vi "integrate_data view.vi"(8 "Y-column names":string[](array[string])=["col0"], 10 "column extension":string[](array[string])=["SCM1_2020Aug_AC.008.txt"], 11 "Graph array":cluster{"output":dbl[], "output":dbl[]}[](array[cluster])=[{"output"=array[591 elements], "output"=array[591 elements]}]) -> ()   [LabVIEW 2025]
uses:
  <vilib>/Analysis/2dsp.llb/Integral Method.ctl
  <vilib>/Analysis/1siggen.llb/Ramp Pattern by Samples.vi
  <vilib>/Analysis/NI_AALBase.lvlib
  <vilib>/gmath/NI_Gmath.lvlib
  <vilib>/Analysis/NI_AALPro.lvlib
panel:
  out "Raw-field, Raw-data, Subtracted, Bkg-field, Bkg-data":string
  out "Integrated (X_interpol. Integ_interpol)":string
  in  "+b":dbl
  in  "*a":dbl=1.0
  out "error":errorcluster
  in  "bkg = Y*a+b":string="-0.02\t1.7128E-5\n-0.02\t1.7128E-5\n-0.02\t1.7128E-5\n-0.02\t1.7128E-5\n-0.02\t1.7128E-5\n-0.02\t1.7128E-5\n-0.02\t1.7128E-5\n-0.02\t1.7128E-5\n-0.02\t1.7128E-5\n-0.02\t1.7128E-5\n-0.02\t1.7128E-5\n-0.0104\t1.7129E-5\n-0.01\t1.7129E-5\n-0.01\t1.7129E-5\n-0.01\t1.7129E-5\n-0.01\t1.7129E-5\n-0.01\t1.7129E-5\n-0.01\t1.7129E-5\n-0.01\t1.7129E-5\n-0.01\t1.7129E-5\n-0.01\t1.7129E-5\n-0.01\t1.7129E-5\n-4E-4\t1.7129E-5\n3.46945E-18\t1.7129E-5\n3.46945E-18\t1.7129E-5\n3.46945E-18\t1.7129E-5\n3.46945E-18\t1.7129E-5\n3.46945E-18\t1.7129E-5\n3.46945E-18\t1.7129E-5\n3.46945E-18\t1.7129E-5\n3.46945E-18\t1.7129E-5\n3.46945E-18\t1.7129E-5\n3.46945E-18\t1.7129E-5\n3.46945E-18\t1.7129E-5\n0.01\t1.713E-5\n0.01\t1.713E-5\n0.01\t1.713E-5\n0.01\t1.713E-5\n0.01\t1.713E-5\n0.01\t1.713E-5\n0.01\t1.713E-5\n0.01\t1.713E-5\n0.01\t1.713E-5\n0.01\t1.713E-5\n0.01\t1.713E-5\n0.02\t1.713E-5\n0.02\t1.713E-5\n0.02\t1.713E-5\n0.02\t1.713E-5\n0.02\t1.713E-5\n0.02\t1.713E-5\n0.02\t1.713E-5\n0.02\t1.713E-5\n0.02\t1.713E-5\n0.02\t1.713E-5\n0.02\t1.713E-5\n0.02\t1.713E-5\n0.02848\t1.7131E-5\n0.03\t1.7131E-5\n0.03\t1.7131E-5\n0.03\t1.7131E-5\n0.03\t1.7131E-5\n0.03\t1.7131E-5\n0.03\t1.7131E-5\n0.03\t1.7131E-5\n0.03\t1.7131E-5\n0.03\t1.7131E-5\n0.03\t1.7131E-5\n0.03\t1.7131E-5\n0.04\t1.7131E-5\n0.04\t1.7131E-5\n0.04\t1.7131E-5\n0.04\t1.7131E-5\n0.04\t1.7131E-5\n0.04\t1.7131E-5\n0.04\t1.7131E-5\n0.04\t1.7131E-5\n0.04\t1.7131E-5\n0.04\t1.7131E-5\n0.04\t1.7131E-5\n0.05\t1.7132E-5\n0.05\t1.7132E-5\n0.05\t1.7132E-5\n0.05\t1.7132E-5\n0.05\t1.7132E-5\n0.05\t1.7132E-5\n0.05\t1.7132E-5\n0.05\t1.7132E-5\n0.05\t1.7132E-5\n0.05\t1.7132E-5\n0.05\t1.7132E-5\n0.05\t1.7132E-5\n0.06\t1.7132E-5\n0.06\t1.7132E-5\n0.06\t1.7132E-5\n0.06\t1.7132E-5\n0.06\t1.7132E-5\n0.06\t1.7132E-5\n0.06\t1.7132E-5\n0.06\t1.7132E-5\n0.06\t1.7132E-5\n0.06\t1.7132E-5\n0.06\t1.7132E-5\n0.06\t1.7132E-5\n0.07\t1.7133E-5\n0.07\t1.7133E-5\n0.07\t1.7133E-5\n0.07\t1.7133E-5\n0.07\t1.7133E-5\n0.07\t1.7133E-5\n0.07\t1.7133E-5\n0.07\t1.7133E-5\n0.07\t1.7133E-5\n0.07\t1.7133E-5\n0.07\t1.7133E-5\n0.08\t1.7133E-5\n0.08\t1.7133E-5\n0.08\t1.7133E-5\n0.08\t1.7133E-5\n0.08\t1.7133E-5\n0.08\t1.7133E-5\n0.08\t1.7133E-5\n0.08\t1.7133E-5\n0.08\t1.7133E-5\n0.08\t1.7133E-5\n0.08\t1.7133E-5\n0.08952\t1.7134E-5\n0.09\t1.7134E-5\n0.09\t1.7134E-5\n0.09\t1.7134E-5\n0.09\t1.7134E-5\n0.09\t1.7134E-5\n0.09\t1.7134E-5\n0.09\t1.7134E-5\n0.09\t1.7134E-5\n0.09\t1.7134E-5\n0.09\t1.7134E-5\n0.09\t1.7134E-5\n0.1\t1.7134E-5\n0.1\t1.7134E-5\n0.1\t1.7134E-5\n0.1\t1.7134E-5\n0.1\t1.7134E-5\n0.1\t1.7134E-5\n0.1\t1.7134E-5\n0.1\t1.7134E-5\n0.1\t1.7134E-5\n0.1\t1.7134E-5\n0.1\t1.7134E-5\n0.1\t1.7134E-5\n0.10948\t1.7134E-5\n0.11\t1.7134E-5\n0.11\t1.7134E-5\n0.11\t1.7134E-5\n0.11\t1.7134E-5\n0.11\t1.7134E-5\n0.11\t1.7134E-5\n0.11\t1.7134E-5\n0.11\t1.7134E-5\n0.11\t1.7134E-5\n0.11\t1.7134E-5\n0.11\t1.7134E-5\n0.12\t1.7135E-5\n0.12\t1.7135E-5\n0.12\t1.7135E-5\n0.12\t1.7135E-5\n0.12\t1.7135E-5\n0.12\t1.7135E-5\n0.12\t1.7135E-5\n0.12\t1.7135E-5\n0.12\t1.7135E-5\n0.12\t1.7135E-5\n0.12\t1.7135E-5\n0.129\t1.7135E-5\n0.13\t1.7135E-5\n0.13\t1.7135E-5\n0.13\t1.7135E-5\n0.13\t1.7135E-5\n0.13\t1.7135E-5\n0.13\t1.7135E-5\n0.13\t1.7135E-5\n0.13\t1.7135E-5\n0.13\t1.7135E-5\n0.13\t1.7135E-5\n0.13\t1.7135E-5\n0.13948\t1.7135E-5\n0.14\t1.7135E-5\n0.14\t1.7135E-5\n0.14\t1.7135E-5\n0.14\t1.7135E-5\n0.14\t1.7135E-5\n0.14\t1.7135E-5\n0.14\t1.7135E-5\n0.14\t1.7135E-5\n0.14\t1.7135E-5\n0.14\t1.7135E-5\n0.14\t1.7135E-5\n0.1496\t1.7136E-5\n0.15\t1.7136E-5\n0.15\t1.7136E-5\n0.15\t1.7136E-5\n0.15\t1.7136E-5\n0.15\t1.7136E-5\n0.15\t1.7136E-5\n0.15\t1.7136E-5\n0.15\t1.7136E-5\n0.15\t1.7136E-5\n0.15\t1.7136E-5\n0.15\t1.7136E-5\n0.16\t1.7136E-5\n0.16\t1.7136E-5\n0.16\t1.7136E-5\n0.16\t1.7136E-5\n0.16\t1.7136E-5\n0.16\t1.7136E-5\n0.16\t1.7136E-5\n0.16\t1.7136E-5\n0.16\t1.7136E-5\n0.16\t1.7136E-5\n0.16\t1.7136E-5\n0.17\t1.7136E-5\n0.17\t1.7136E-5\n0.17\t1.7136E-5\n0.17\t1.7136E-5\n0.17\t1.7136E-5\n0.17\t1.7136E-5\n0.17\t1.7136E-5\n0.17\t1.7136E-5\n0.17\t1.7136E-5\n0.17\t1.7136E-5\n0.17\t1.7136E-5\n0.18\t1.7137E-5\n0.18\t1.7137E-5\n0.18\t1.7137E-5\n0.18\t1.7137E-5\n0.18\t1.7137E-5\n0.18\t1.7137E-5\n0.18\t1.7137E-5\n0.18\t1.7137E-5\n0.18\t1.7137E-5\n0.18\t1.7137E-5\n0.18\t1.7137E-5\n0.18\t1.7137E-5\n0.19\t1.7137E-5\n0.19\t1.7137E-5\n0.19\t1.7137E-5\n0.19\t1.7137E-5\n0.19\t1.7137E-5\n0.19\t1.7137E-5\n0.19\t1.7137E-5\n0.19\t1.7137E-5\n0.19\t1.7137E-5\n0.19\t1.7137E-5\n0.19\t1.7137E-5\n0.19\t1.7137E-5\n0.19952\t1.7137E-5\n0.2\t1.7137E-5\n0.2\t1.7137E-5\n0.2\t1.7137E-5\n0.2\t1.7137E-5\n0.2\t1.7137E-5\n0.2\t1.7137E-5\n0.2\t1.7137E-5\n0.2\t1.7137E-5\n0.2\t1.7137E-5\n0.2\t1.7137E-5\n0.2\t1.7137E-5\n0.20956\t1.7137E-5\n0.21\t1.7137E-5\n0.21\t1.7137E-5\n0.21\t1.7137E-5\n0.21\t1.7137E-5\n0.21\t1.7137E-5\n0.21\t1.7137E-5\n0.21\t1.7137E-5\n0.21\t1.7137E-5\n0.21\t1.7137E-5\n0.21\t1.7137E-5\n0.21\t1.7137E-5\n0.22\t1.7138E-5\n0.22\t1.7138E-5\n0.22\t1.7138E-5\n0.22\t1.7138E-5\n0.22\t1.7138E-5\n0.22\t1.7138E-5\n0.22\t1.7138E-5\n0.22\t1.7138E-5\n0.22\t1.7138E-5\n0.22\t1.7138E-5\n0.22\t1.7138E-5\n0.23\t1.7138E-5\n0.23\t1.7138E-5\n0.23\t1.7138E-5\n0.23\t1.7138E-5\n0.23\t1.7138E-5\n0.23\t1.7138E-5\n0.23\t1.7138E-5\n0.23\t1.7138E-5\n0.23\t1.7138E-5\n0.23\t1.7138E-5\n0.23\t1.7138E-5\n0.23948\t1.7138E-5\n0.24\t1.7138E-5\n0.24\t1.7138E-5\n0.24\t1.7138E-5\n0.24\t1.7138E-5\n0.24\t1.7138E-5\n0.24\t1.7138E-5\n0.24\t1.7138E-5\n0.24\t1.7138E-5\n0.24\t1.7138E-5\n0.24\t1.7138E-5\n0.24\t1.7138E-5\n0.25\t1.7138E-5\n0.25\t1.7138E-5\n0.25\t1.7138E-5\n0.25\t1.7138E-5\n0.25\t1.7138E-5\n0.25\t1.7138E-5\n0.25\t1.7138E-5\n0.25\t1.7138E-5\n0.25\t1.7138E-5\n0.25\t1.7138E-5\n0.25\t1.7138E-5\n0.26\t1.7139E-5\n0.26\t1.7139E-5\n0.26\t1.7139E-5\n0.26\t1.7139E-5\n0.26\t1.7139E-5\n0.26\t1.7139E-5\n0.26\t1.7139E-5\n0.26\t1.7139E-5\n0.26\t1.7139E-5\n0.26\t1.7139E-5\n0.26\t1.7139E-5\n0.26\t1.7139E-5\n0.27\t1.7139E-5\n0.27\t1.7139E-5\n0.27\t1.7139E-5\n0.27\t1.7139E-5\n0.27\t1.7139E-5\n0.27\t1.7139E-5\n0.27\t1.7139E-5\n0.27\t1.7139E-5\n0.27\t1.7139E-5\n0.27\t1.7139E-5\n0.27\t1.7139E-5\n0.27\t1.7139E-5\n0.28\t1.7139E-5\n0.28\t1.7139E-5\n0.28\t1.7139E-5\n0.28\t1.7139E-5\n0.28\t1.7139E-5\n0.28\t1.7139E-5\n0.28\t1.7139E-5\n0.28\t1.7139E-5\n0.28\t1.7139E-5\n0.28\t1.7139E-5\n0.28\t1.7139E-5\n0.28\t1.7139E-5\n0.28848\t1.7139E-5\n0.29\t1.7139E-5\n0.29\t1.7139E-5\n0.29\t1.7139E-5\n0.29\t1.7139E-5\n0.29\t1.7139E-5\n0.29\t1.7139E-5\n0.29\t1.7139E-5\n0.29\t1.7139E-5\n0.29\t1.7139E-5\n0.29\t1.7139E-5\n0.29\t1.7139E-5\n0.3\t1.7139E-5\n0.3\t1.7139E-5\n0.3\t1.7139E-5\n0.3\t1.7139E-5\n0.3\t1.7139E-5\n0.3\t1.7139E-5\n0.3\t1.7139E-5\n0.3\t1.7139E-5\n0.3\t1.7139E-5\n0.3\t1.7139E-5\n0.3\t1.7139E-5\n0.30956\t1.7139E-5\n0.31\t1.7139E-5\n0.31\t1.7139E-5\n0.31\t1.7139E-5\n0.31\t1.7139E-5\n0.31\t1.7139E-5\n0.31\t1.7139E-5\n0.31\t1.7139E-5\n0.31\t1.7139E-5\n0.31\t1.7139E-5\n0.31\t1.7139E-5\n0.31\t1.7139E-5\n0.32\t1.7139E-5\n0.32\t1.7139E-5\n0.32\t1.7139E-5\n0.32\t1.7139E-5\n0.32\t1.7139E-5\n0.32\t1.7139E-5\n0.32\t1.7139E-5\n0.32\t1.7139E-5\n0.32\t1.7139E-5\n0.32\t1.7139E-5\n0.32\t1.7139E-5\n0.33\t1.7139E-5\n0.33\t1.7139E-5\n0.33\t1.7139E-5\n0.33\t1.7139E-5\n0.33\t1.7139E-5\n0.33\t1.7139E-5\n0.33\t1.7139E-5\n0.33\t1.7139E-5\n0.33\t1.7139E-5\n0.33\t1.7139E-5\n0.33\t1.7139E-5\n0.33\t1.7139E-5\n0.33952\t1.714E-5\n0.34\t1.714E-5\n0.34\t1.714E-5\n0.34\t1.714E-5\n0.34\t1.714E-5\n0.34\t1.714E-5\n0.34\t1.714E-5\n0.34\t1.714E-5\n0.34\t1.714E-5\n0.34\t1.714E-5\n0.34\t1.714E-5\n0.34\t1.714E-5\n0.35\t1.714E-5\n0.35\t1.714E-5\n0.35\t1.714E-5\n0.35\t1.714E-5\n0.35\t1.714E-5\n0.35\t1.714E-5\n0.35\t1.714E-5\n0.35\t1.714E-5\n0.35\t1.714E-5\n0.35\t1.714E-5\n0.35\t1.714E-5\n0.36\t1.714E-5\n0.36\t1.714E-5\n0.36\t1.714E-5\n0.36\t1.714E-5\n0.36\t1.714E-5\n0.36\t1.714E-5\n0.36\t1.714E-5\n0.36\t1.714E-5\n0.36\t1.714E-5\n0.36\t1.714E-5\n0.36\t1.714E-5\n0.36\t1.714E-5\n0.37\t1.714E-5\n0.37\t1.714E-5\n0.37\t1.714E-5\n0.37\t1.714E-5\n0.37\t1.714E-5\n0.37\t1.714E-5\n0.37\t1.714E-5\n0.37\t1.714E-5\n0.37\t1.714E-5\n0.37\t1.714E-5\n0.37\t1.714E-5\n0.37\t1.714E-5\n0.3796\t1.714E-5\n0.38\t1.714E-5\n0.38\t1.714E-5\n0.38\t1.714E-5\n0.38\t1.714E-5\n0.38\t1.714E-5\n0.38\t1.714E-5\n0.38\t1.714E-5\n0.38\t1.714E-5\n0.38\t1.714E-5\n0.38\t1.714E-5\n0.38\t1.714E-5\n0.39\t1.714E-5\n0.39\t1.714E-5\n0.39\t1.714E-5\n0.39\t1.714E-5\n0.39\t1.714E-5\n0.39\t1.714E-5\n0.39\t1.714E-5\n0.39\t1.714E-5\n0.39\t1.714E-5\n0.39\t1.714E-5\n0.39\t1.714E-5\n0.39\t1.714E-5\n0.4\t1.714E-5\n0.4\t1.714E-5\n0.4\t1.714E-5\n0.4\t1.714E-5\n0.4\t1.714E-5\n0.4\t1.714E-5\n0.4\t1.714E-5\n0.4\t1.714E-5\n0.4\t1.714E-5\n0.4\t1.714E-5\n0.4\t1.714E-5\n0.41\t1.714E-5\n0.41\t1.714E-5\n0.41\t1.714E-5\n0.41\t1.714E-5\n0.41\t1.714E-5\n0.41\t1.714E-5\n0.41\t1.714E-5\n0.41\t1.714E-5\n0.41\t1.714E-5\n0.41\t1.714E-5\n0.41\t1.714E-5\n0.4196\t1.714E-5\n0.42\t1.714E-5\n0.42\t1.714E-5\n0.42\t1.714E-5\n0.42\t1.714E-5\n0.42\t1.714E-5\n0.42\t1.714E-5\n0.42\t1.714E-5\n0.42\t1.714E-5\n0.42\t1.714E-5\n0.42\t1.714E-5\n0.43\t1.714E-5\n0.43\t1.714E-5\n0.43\t1.714E-5\n0.43\t1.714E-5\n0.43\t1.714E-5\n0.43\t1.714E-5\n0.43\t1.714E-5\n0.43\t1.714E-5\n0.43\t1.714E-5\n0.43\t1.714E-5\n0.43\t1.714E-5\n0.43\t1.714E-5\n0.44\t1.714E-5\n0.44\t1.714E-5\n0.44\t1.714E-5\n0.44\t1.714E-5\n0.44\t1.714E-5\n0.44\t1.714E-5\n0.44\t1.714E-5\n0.44\t1.714E-5\n0.44\t1.714E-5\n0.44\t1.714E-5\n0.44\t1.714E-5\n0.45\t1.714E-5\n0.45\t1.714E-5\n0.45\t1.714E-5\n0.45\t1.714E-5\n0.45\t1.714E-5\n0.45\t1.714E-5\n0.45\t1.714E-5\n0.45\t1.714E-5\n0.45\t1.714E-5\n0.45\t1.714E-5\n0.45\t1.714E-5\n0.45952\t1.714E-5\n0.46\t1.714E-5\n0.46\t1.714E-5\n0.46\t1.714E-5\n0.46\t1.714E-5\n0.46\t1.714E-5\n0.46\t1.714E-5\n0.46\t1.714E-5\n0.46\t1.714E-5\n0.46\t1.714E-5\n0.46\t1.714E-5\n0.46\t1.714E-5\n0.47\t1.7139E-5\n0.47\t1.7139E-5\n0.47\t1.7139E-5\n0.47\t1.7139E-5\n0.47\t1.7139E-5\n0.47\t1.7139E-5\n0.47\t1.7139E-5\n0.47\t1.7139E-5\n0.47\t1.7139E-5\n0.47\t1.7139E-5\n0.47\t1.7139E-5\n0.47\t1.7139E-5\n0.48\t1.7139E-5\n0.48\t1.7139E-5\n0.48\t1.7139E-5\n0.48\t1.7139E-5\n0.48\t1.7139E-5\n0.48\t1.7139E-5\n0.48\t1.7139E-5\n0.48\t1.7139E-5\n0.48\t1.7139E-5\n0.48\t1.7139E-5\n0.48\t1.7139E-5\n0.49\t1.7139E-5\n0.49\t1.7139E-5\n0.49\t1.7139E-5\n0.49\t1.7139E-5\n0.49\t1.7139E-5\n0.49\t1.7139E-5\n0.49\t1.7139E-5\n0.49\t1.7139E-5\n0.49\t1.7139E-5\n0.49\t1.7139E-5\n0.49\t1.7139E-5\n0.49\t1.7139E-5\n0.5\t1.7139E-5\n0.5\t1.7139E-5\n0.5\t1.7139E-5\n0.5\t1.7139E-5\n0.5\t1.7139E-5\n0.5\t1.7139E-5\n0.5\t1.7139E-5\n0.5\t1.7139E-5\n0.5\t1.7139E-5\n0.5\t1.7139E-5\n0.5\t1.7139E-5\n0.51\t1.7139E-5\n0.51\t1.7139E-5\n0.51\t1.7139E-5\n0.51\t1.7139E-5\n0.51\t1.7139E-5\n0.51\t1.7139E-5\n0.51\t1.7139E-5\n0.51\t1.7139E-5\n0.51\t1.7139E-5\n0.51\t1.7139E-5\n0.51\t1.7139E-5\n0.52\t1.7139E-5\n0.52\t1.7139E-5\n0.52\t1.7139E-5\n0.52\t1.7139E-5\n0.52\t1.7139E-5\n0.52\t1.7139E-5\n0.52\t1.7139E-5\n0.52\t1.7139E-5\n0.52\t1.7139E-5\n0.52\t1.7139E-5\n0.52\t1.7139E-5\n0.52\t1.7139E-5\n0.53\t1.7139E-5\n0.53\t1.7139E-5\n0.53\t1.7139E-5\n0.53\t1.7139E-5\n0.53\t1.7139E-5\n0.53\t1.7139E-5\n0.53\t1.7139E-5\n0.53\t1.7139E-5\n0.53\t1.7139E-5\n0.53\t1.7139E-5\n0.53\t1.7139E-5\n0.54\t1.7138E-5\n0.54\t1.7138E-5\n0.54\t1.7138E-5\n0.54\t1.7138E-5\n0.54\t1.7138E-5\n0.54\t1.7138E-5\n0.54\t1.7138E-5\n0.54\t1.7138E-5\n0.54\t1.7138E-5\n0.54\t1.7138E-5\n0.54\t1.7138E-5\n0.5496\t1.7138E-5\n0.55\t1.7138E-5\n0.55\t1.7138E-5\n0.55\t1.7138E-5\n0.55\t1.7138E-5\n0.55\t1.7138E-5\n0.55\t1.7138E-5\n0.55\t1.7138E-5\n0.55\t1.7138E-5\n0.55\t1.7138E-5\n0.55\t1.7138E-5\n0.55\t1.7138E-5\n0.56\t1.7138E-5\n0.56\t1.7138E-5\n0.56\t1.7138E-5\n0.56\t1.7138E-5\n0.56\t1.7138E-5\n0.56\t1.7138E-5\n0.56\t1.7138E-5\n0.56\t1.7138E-5\n0.56\t1.7138E-5\n0.56\t1.7138E-5\n0.56\t1.7138E-5\n0.56952\t1.7138E-5\n0.57\t1.7138E-5\n0.57\t1.7138E-5\n0.57\t1.7138E-5\n0.57\t1.7138E-5\n0.57\t1.7138E-5\n0.57\t1.7138E-5\n0.57\t1.7138E-5\n0.57\t1.7138E-5\n0.57\t1.7138E-5\n0.57\t1.7138E-5\n0.57\t1.7138E-5\n0.57952\t1.7138E-5\n0.58\t1.7138E-5\n0.58\t1.7138E-5\n0.58\t1.7138E-5\n0.58\t1.7138E-5\n0.58\t1.7138E-5\n0.58\t1.7138E-5\n0.58\t1.7138E-5\n0.58\t1.7138E-5\n0.58\t1.7138E-5\n0.58\t1.7138E-5\n0.58\t1.7138E-5\n0.59\t1.7137E-5\n0.59\t1.7137E-5\n0.59\t1.7137E-5\n0.59\t1.7137E-5\n0.59\t1.7137E-5\n0.59\t1.7137E-5\n0.59\t1.7137E-5\n0.59\t1.7137E-5\n0.59\t1.7137E-5\n0.59\t1.7137E-5\n0.59\t1.7137E-5\n0.6\t1.7137E-5\n0.6\t1.7137E-5\n0.6\t1.7137E-5\n0.6\t1.7137E-5\n0.6\t1.7137E-5\n0.6\t1.7137E-5\n0.6\t1.7137E-5\n0.6\t1.7137E-5\n0.6\t1.7137E-5\n0.6\t1.7137E-5\n0.6\t1.7137E-5\n0.60952\t1.7137E-5\n0.61\t1.7137E-5\n0.61\t1.7137E-5\n0.61\t1.7137E-5\n0.61\t1.7137E-5\n0.61\t1.7137E-5\n0.61\t1.7137E-5\n0.61\t1.7137E-5\n0.61\t1.7137E-5\n0.61\t1.7137E-5\n0.61\t1.7137E-5\n0.61\t1.7137E-5\n0.61952\t1.7137E-5\n0.62\t1.7137E-5\n0.62\t1.7137E-5\n0.62\t1.7137E-5\n0.62\t1.7137E-5\n0.62\t1.7137E-5\n0.62\t1.7137E-5\n0.62\t1.7137E-5\n0.62\t1.7137E-5\n0.62\t1.7137E-5\n0.62\t1.7137E-5\n0.62\t1.7137E-5\n0.62956\t1.7136E-5\n0.63\t1.7136E-5\n0.63\t1.7136E-5\n0.63\t1.7136E-5\n0.63\t1.7136E-5\n0.63\t1.7136E-5\n0.63\t1.7136E-5\n0.63\t1.7136E-5\n0.63\t1.7136E-5\n0.63\t1.7136E-5\n0.63\t1.7136E-5\n0.63\t1.7136E-5\n0.63952\t1.7136E-5\n0.64\t1.7136E-5\n0.64\t1.7136E-5\n0.64\t1.7136E-5\n0.64\t1.7136E-5\n0.64\t1.7136E-5\n0.64\t1.7136E-5\n0.64\t1.7136E-5\n0.64\t1.7136E-5\n0.64\t1.7136E-5\n0.64\t1.7136E-5\n0.64\t1.7136E-5\n0.65\t1.7136E-5\n0.65\t1.7136E-5\n0.65\t1.7136E-5\n0.65\t1.7136E-5\n0.65\t1.7136E-5\n0.65\t1.7136E-5\n0.65\t1.7136E-5\n0.65\t1.7136E-5\n0.65\t1.7136E-5\n0.65\t1.7136E-5\n0.65\t1.7136E-5\n0.66\t1.7135E-5\n0.66\t1.7135E-5\n0.66\t1.7135E-5\n0.66\t1.7135E-5\n0.66\t1.7135E-5\n0.66\t1.7135E-5\n0.66\t1.7135E-5\n0.66\t1.7135E-5\n0.66\t1.7135E-5\n0.66\t1.7135E-5\n0.66\t1.7135E-5\n0.66\t1.7135E-5\n0.67\t1.7135E-5\n0.67\t1.7135E-5\n0.67\t1.7135E-5\n0.67\t1.7135E-5\n0.67\t1.7135E-5\n0.67\t1.7135E-5\n0.67\t1.7135E-5\n0.67\t1.7135E-5\n0.67\t1.7135E-5\n0.67\t1.7135E-5\n0.67\t1.7135E-5\n0.67\t1.7135E-5\n0.68\t1.7135E-5\n0.68\t1.7135E-5\n0.68\t1.7135E-5\n0.68\t1.7135E-5\n0.68\t1.7135E-5\n0.68\t1.7135E-5\n0.68\t1.7135E-5\n0.68\t1.7135E-5\n0.68\t1.7135E-5\n0.68\t1.7135E-5\n0.68\t1.7135E-5\n0.69\t1.7134E-5\n0.69\t1.7134E-5\n0.69\t1.7134E-5\n0.69\t1.7134E-5\n0.69\t1.7134E-5\n0.69\t1.7134E-5\n0.69\t1.7134E-5\n0.69\t1.7134E-5\n0.69\t1.7134E-5\n0.69\t1.7134E-5\n0.69\t1.7134E-5\n0.69944\t1.7134E-5\n0.7\t1.7134E-5\n0.7\t1.7134E-5\n0.7\t1.7134E-5\n0.7\t1.7134E-5\n0.7\t1.7134E-5\n0.7\t1.7134E-5\n0.7\t1.7134E-5\n0.7\t1.7134E-5\n0.7\t1.7134E-5\n0.7\t1.7134E-5\n0.7\t1.7134E-5\n0.71\t1.7133E-5\n0.71\t1.7133E-5\n0.71\t1.7133E-5\n0.71\t1.7133E-5\n0.71\t1.7133E-5\n0.71\t1.7133E-5\n0.71\t1.7133E-5\n0.71\t1.7133E-5\n0.71\t1.7133E-5\n0.71\t1.7133E-5\n0.71\t1.7133E-5\n0.71\t1.7133E-5\n0.72\t1.7133E-5\n0.72\t1.7133E-5\n0.72\t1.7133E-5\n0.72\t1.7133E-5\n0.72\t1.7133E-5\n0.72\t1.7133E-5\n0.72\t1.7133E-5\n0.72\t1.7133E-5\n0.72\t1.7133E-5\n0.72\t1.7133E-5\n0.72\t1.7133E-5\n0.72\t1.7133E-5\n0.7296\t1.7133E-5\n0.73\t1.7133E-5\n0.73\t1.7133E-5\n0.73\t1.7133E-5\n0.73\t1.7133E-5\n0.73\t1.7133E-5\n0.73\t1.7133E-5\n0.73\t1.7133E-5\n0.73\t1.7133E-5\n0.73\t1.7133E-5\n0.73\t1.7133E-5\n0.74\t1.7132E-5\n0.74\t1.7132E-5\n0.74\t1.7132E-5\n0.74\t1.7132E-5\n0.74\t1.7132E-5\n0.74\t1.7132E-5\n0.74\t1.7132E-5\n0.74\t1.7132E-5\n0.74\t1.7132E-5\n0.74\t1.7132E-5\n0.74\t1.7132E-5\n0.74952\t1.7132E-5\n0.75\t1.7132E-5\n0.75\t1.7132E-5\n0.75\t1.7132E-5\n0.75\t1.7132E-5\n0.75\t1.7132E-5\n0.75\t1.7132E-5\n0.75\t1.7132E-5\n0.75\t1.7132E-5\n0.75\t1.7132E-5\n0.75\t1.7132E-5\n0.75\t1.7132E-5\n0.76\t1.7131E-5\n0.76\t1.7131E-5\n0.76\t1.7131E-5\n0.76\t1.7131E-5\n0.76\t1.7131E-5\n0.76\t1.7131E-5\n0.76\t1.7131E-5\n0.76\t1.7131E-5\n0.76\t1.7131E-5\n0.76\t1.7131E-5\n0.76\t1.7131E-5\n0.76952\t1.7131E-5\n0.77\t1.7131E-5\n0.77\t1.7131E-5\n0.77\t1.7131E-5\n0.77\t1.7131E-5\n0.77\t1.7131E-5\n0.77\t1.7131E-5\n0.77\t1.7131E-5\n0.77\t1.7131E-5\n0.77\t1.7131E-5\n0.77\t1.7131E-5\n0.77\t1.7131E-5\n0.78\t1.713E-5\n0.78\t1.713E-5\n0.78\t1.713E-5\n0.78\t1.713E-5\n0.78\t1.713E-5\n0.78\t1.713E-5\n0.78\t1.713E-5\n0.78\t1.713E-5\n0.78\t1.713E-5\n0.78\t1.713E-5\n0.78\t1.713E-5\n0.7896\t1.713E-5\n0.79\t1.713E-5\n0.79\t1.713E-5\n0.79\t1.713E-5\n0.79\t1.713E-5\n0.79\t1.713E-5\n0.79\t1.713E-5\n0.79\t1.713E-5\n0.79\t1.713E-5\n0.79\t1.713E-5\n0.79\t1.713E-5\n0.79\t1.713E-5\n0.8\t1.7129E-5\n0.8\t1.7129E-5\n0.8\t1.7129E-5\n0.8\t1.7129E-5\n0.8\t1.7129E-5\n0.8\t1.7129E-5\n0.8\t1.7129E-5\n0.8\t1.7129E-5\n0.8\t1.7129E-5\n0.8\t1.7129E-5\n0.8\t1.7129E-5\n0.80944\t1.7129E-5\n0.81\t1.7129E-5\n0.81\t1.7129E-5\n0.81\t1.7129E-5\n0.81\t1.7129E-5\n0.81\t1.7129E-5\n0.81\t1.7129E-5\n0.81\t1.7129E-5\n0.81\t1.7129E-5\n0.81\t1.7129E-5\n0.81\t1.7129E-5\n0.81\t1.7129E-5\n0.82\t1.7128E-5\n0.82\t1.7128E-5\n0.82\t1.7128E-5\n0.82\t1.7128E-5\n0.82\t1.7128E-5\n0.82\t1.7128E-5\n0.82\t1.7128E-5\n0.82\t1.7128E-5\n0.82\t1.7128E-5\n0.82\t1.7128E-5\n0.82\t1.7128E-5\n0.8296\t1.7128E-5\n0.83\t1.7128E-5\n0.83\t1.7128E-5\n0.83\t1.7128E-5\n0.83\t1.7128E-5\n0.83\t1.7128E-5\n0.83\t1.7128E-5\n0.83\t1.7128E-5\n0.83\t1.7128E-5\n0.83\t1.7128E-5\n0.83\t1.7128E-5\n0.83\t1.7128E-5\n0.84\t1.7127E-5\n0.84\t1.7127E-5\n0.84\t1.7127E-5\n0.84\t1.7127E-5\n0.84\t1.7127E-5\n0.84\t1.7127E-5\n0.84\t1.7127E-5\n0.84\t1.7127E-5\n0.84\t1.7127E-5\n0.84\t1.7127E-5\n0.84\t1.7127E-5\n0.84952\t1.7126E-5\n0.85\t1.7126E-5\n0.85\t1.7126E-5\n0.85\t1.7126E-5\n0.85\t1.7126E-5\n0.85\t1.7126E-5\n0.85\t1.7126E-5\n0.85\t1.7126E-5\n0.85\t1.7126E-5\n0.85\t1.7126E-5\n0.85\t1.7126E-5\n0.85\t1.7126E-5\n0.85944\t1.7126E-5\n0.86\t1.7126E-5\n0.86\t1.7126E-5\n0.86\t1.7126E-5\n0.86\t1.7126E-5\n0.86\t1.7126E-5\n0.86\t1.7126E-5\n0.86\t1.7126E-5\n0.86\t1.7126E-5\n0.86\t1.7126E-5\n0.86\t1.7126E-5\n0.86\t1.7126E-5\n0.87\t1.7125E-5\n0.87\t1.7125E-5\n0.87\t1.7125E-5\n0.87\t1.7125E-5\n0.87\t1.7125E-5\n0.87\t1.7125E-5\n0.87\t1.7125E-5\n0.87\t1.7125E-5\n0.87\t1.7125E-5\n0.87\t1.7125E-5\n0.87\t1.7125E-5\n0.88\t1.7125E-5\n0.88\t1.7125E-5\n0.88\t1.7125E-5\n0.88\t1.7125E-5\n0.88\t1.7125E-5\n0.88\t1.7125E-5\n0.88\t1.7125E-5\n0.88\t1.7125E-5\n0.88\t1.7125E-5\n0.88\t1.7125E-5\n0.88\t1.7125E-5\n0.88952\t1.7124E-5\n0.89\t1.7124E-5\n0.89\t1.7124E-5\n0.89\t1.7124E-5\n0.89\t1.7124E-5\n0.89\t1.7124E-5\n0.89\t1.7124E-5\n0.89\t1.7124E-5\n0.89\t1.7124E-5\n0.89\t1.7124E-5\n0.89\t1.7124E-5\n0.89\t1.7124E-5\n0.9\t1.7123E-5\n0.9\t1.7123E-5\n0.9\t1.7123E-5\n0.9\t1.7123E-5\n0.9\t1.7123E-5\n0.9\t1.7123E-5\n0.9\t1.7123E-5\n0.9\t1.7123E-5\n0.9\t1.7123E-5\n0.9\t1.7123E-5\n0.9\t1.7123E-5\n0.90996\t1.7123E-5\n0.91\t1.7123E-5\n0.91\t1.7123E-5\n0.91\t1.7123E-5\n0.91\t1.7123E-5\n0.91\t1.7123E-5\n0.91\t1.7123E-5\n0.91\t1.7123E-5\n0.91\t1.7123E-5\n0.91\t1.7123E-5\n0.91\t1.7123E-5\n0.91\t1.7123E-5\n0.92\t1.7122E-5\n0.92\t1.7122E-5\n0.92\t1.7122E-5\n0.92\t1.7122E-5\n0.92\t1.7122E-5\n0.92\t1.7122E-5\n0.92\t1.7122E-5\n0.92\t1.7122E-5\n0.92\t1.7122E-5\n0.92\t1.7122E-5\n0.92\t1.7122E-5\n0.92\t1.7122E-5\n0.92948\t1.7121E-5\n0.93\t1.7121E-5\n0.93\t1.7121E-5\n0.93\t1.7121E-5\n0.93\t1.7121E-5\n0.93\t1.7121E-5\n0.93\t1.7121E-5\n0.93\t1.7121E-5\n0.93\t1.7121E-5\n0.93\t1.7121E-5\n0.93\t1.7121E-5\n0.93\t1.7121E-5\n0.93832\t1.7121E-5\n0.94\t1.7121E-5\n0.94\t1.7121E-5\n0.94\t1.7121E-5\n0.94\t1.7121E-5\n0.94\t1.7121E-5\n0.94\t1.7121E-5\n0.94\t1.7121E-5\n0.94\t1.7121E-5\n0.94\t1.7121E-5\n0.94\t1.7121E-5\n0.94\t1.7121E-5\n0.95\t1.712E-5\n0.95\t1.712E-5\n0.95\t1.712E-5\n0.95\t1.712E-5\n0.95\t1.712E-5\n0.95\t1.712E-5\n0.95\t1.712E-5\n0.95\t1.712E-5\n0.95\t1.712E-5\n0.95\t1.712E-5\n0.95\t1.712E-5\n0.95\t1.712E-5\n0.95896\t1.7119E-5\n0.96\t1.7119E-5\n0.96\t1.7119E-5\n0.96\t1.7119E-5\n0.96\t1.7119E-5\n0.96\t1.7119E-5\n0.96\t1.7119E-5\n0.96\t1.7119E-5\n0.96\t1.7119E-5\n0.96\t1.7119E-5\n0.96\t1.7119E-5\n0.96\t1.7119E-5\n0.96952\t1.7118E-5\n0.97\t1.7118E-5\n0.97\t1.7118E-5\n0.97\t1.7118E-5\n0.97\t1.7118E-5\n0.97\t1.7118E-5\n0.97\t1.7118E-5\n0.97\t1.7118E-5\n0.97\t1.7118E-5\n0.97\t1.7118E-5\n0.97\t1.7118E-5\n0.97\t1.7118E-5\n0.98\t1.7118E-5\n0.98\t1.7118E-5\n0.98\t1.7118E-5\n0.98\t1.7118E-5\n0.98\t1.7118E-5\n0.98\t1.7118E-5\n0.98\t1.7118E-5\n0.98\t1.7118E-5\n0.98\t1.7118E-5\n0.98\t1.7118E-5\n0.98\t1.7118E-5\n0.99\t1.7117E-5\n0.99\t1.7117E-5\n0.99\t1.7117E-5\n0.99\t1.7117E-5\n0.99\t1.7117E-5\n0.99\t1.7117E-5\n0.99\t1.7117E-5\n0.99\t1.7117E-5\n0.99\t1.7117E-5\n0.99\t1.7117E-5\n0.99\t1.7117E-5\n0.99\t1.7117E-5\n0.99956\t1.7116E-5\n1\t1.7116E-5\n1\t1.7116E-5\n1\t1.7116E-5\n1\t1.7116E-5\n1\t1.7116E-5\n1\t1.7116E-5\n1\t1.7116E-5\n1\t1.7116E-5\n1\t1.7116E-5\n1\t1.7116E-5\n1\t1.7116E-5\n1.01\t1.7115E-5\n1.01\t1.7115E-5\n1.01\t1.7115E-5\n1.01\t1.7115E-5\n1.01\t1.7115E-5\n1.01\t1.7115E-5\n1.01\t1.7115E-5\n1.01\t1.7115E-5\n1.01\t1.7115E-5\n1.01\t1.7115E-5\n1.01\t1.7115E-5\n1.02\t1.7115E-5\n1.02\t1.7115E-5\n1.02\t1.7115E-5\n1.02\t1.7115E-5\n1.02\t1.7115E-5\n1.02\t1.7115E-5\n1.02\t1.7115E-5\n1.02\t1.7115E-5\n1.02\t1.7115E-5\n1.02\t1.7115E-5\n1.02\t1.7115E-5\n1.03\t1.7114E-5\n1.03\t1.7114E-5\n1.03\t1.7114E-5\n1.03\t1.7114E-5\n1.03\t1.7114E-5\n1.03\t1.7114E-5\n1.03\t1.7114E-5\n1.03\t1.7114E-5\n1.03\t1.7114E-5\n1.03\t1.7114E-5\n1.03\t1.7114E-5\n1.04\t1.7113E-5\n1.04\t1.7113E-5\n1.04\t1.7113E-5\n1.04\t1.7113E-5\n1.04\t1.7113E-5\n1.04\t1.7113E-5\n1.04\t1.7113E-5\n1.04\t1.7113E-5\n1.04\t1.7113E-5\n1.04\t1.7113E-5\n1.04\t1.7113E-5\n1.04956\t1.7112E-5\n1.05\t1.7112E-5\n1.05\t1.7112E-5\n1.05\t1.7112E-5\n1.05\t1.7112E-5\n1.05\t1.7112E-5\n1.05\t1.7112E-5\n1.05\t1.7112E-5\n1.05\t1.7112E-5\n1.05\t1.7112E-5\n1.05\t1.7112E-5\n1.05\t1.7112E-5\n1.06\t1.7111E-5\n1.06\t1.7111E-5\n1.06\t1.7111E-5\n1.06\t1.7111E-5\n1.06\t1.7111E-5\n1.06\t1.7111E-5\n1.06\t1.7111E-5\n1.06\t1.7111E-5\n1.06\t1.7111E-5\n1.06\t1.7111E-5\n1.06\t1.7111E-5\n1.07\t1.711E-5\n1.07\t1.711E-5\n1.07\t1.711E-5\n1.07\t1.711E-5\n1.07\t1.711E-5\n1.07\t1.711E-5\n1.07\t1.711E-5\n1.07\t1.711E-5\n1.07\t1.711E-5\n1.07\t1.711E-5\n1.07\t1.711E-5\n1.08\t1.7109E-5\n1.08\t1.7109E-5\n1.08\t1.7109E-5\n1.08\t1.7109E-5\n1.08\t1.7109E-5\n1.08\t1.7109E-5\n1.08\t1.7109E-5\n1.08\t1.7109E-5\n1.08\t1.7109E-5\n1.08\t1.7109E-5\n1.08\t1.7109E-5\n1.08\t1.7109E-5\n1.08956\t1.7109E-5\n1.09\t1.7109E-5\n1.09\t1.7109E-5\n1.09\t1.7109E-5\n1.09\t1.7109E-5\n1.09\t1.7109E-5\n1.09\t1.7109E-5\n1.09\t1.7109E-5\n1.09\t1.7109E-5\n1.09\t1.7109E-5\n1.09\t1.7109E-5\n1.1\t1.7108E-5\n1.1\t1.7108E-5\n1.1\t1.7108E-5\n1.1\t1.7108E-5\n1.1\t1.7108E-5\n1.1\t1.7108E-5\n1.1\t1.7108E-5\n1.1\t1.7108E-5\n1.1\t1.7108E-5\n1.1\t1.7108E-5\n1.1\t1.7108E-5\n1.1\t1.7108E-5\n1.10952\t1.7107E-5\n1.11\t1.7107E-5\n1.11\t1.7107E-5\n1.11\t1.7107E-5\n1.11\t1.7107E-5\n1.11\t1.7107E-5\n1.11\t1.7107E-5\n1.11\t1.7107E-5\n1.11\t1.7107E-5\n1.11\t1.7107E-5\n1.11\t1.7107E-5\n1.11\t1.7107E-5\n1.12\t1.7106E-5\n1.12\t1.7106E-5\n1.12\t1.7106E-5\n1.12\t1.7106E-5\n1.12\t1.7106E-5\n1.12\t1.7106E-5\n1.12\t1.7106E-5\n1.12\t1.7106E-5\n1.12\t1.7106E-5\n1.12\t1.7106E-5\n1.12\t1.7106E-5\n1.12948\t1.7105E-5\n1.13\t1.7105E-5\n1.13\t1.7105E-5\n1.13\t1.7105E-5\n1.13\t1.7105E-5\n1.13\t1.7105E-5\n1.13\t1.7105E-5\n1.13\t1.7105E-5\n1.13\t1.7105E-5\n1.13\t1.7105E-5\n1.13\t1.7105E-5\n1.13\t1.7105E-5\n1.13948\t1.7104E-5\n1.14\t1.7104E-5\n1.14\t1.7104E-5\n1.14\t1.7104E-5\n1.14\t1.7104E-5\n1.14\t1.7104E-5\n1.14\t1.7104E-5\n1.14\t1.7104E-5\n1.14\t1.7104E-5\n1.14\t1.7104E-5\n1.14\t1.7104E-5\n1.14\t1.7104E-5\n1.15\t1.7103E-5\n1.15\t1.7103E-5\n1.15\t1.7103E-5\n1.15\t1.7103E-5\n1.15\t1.7103E-5\n1.15\t1.7103E-5\n1.15\t1.7103E-5\n1.15\t1.7103E-5\n1.15\t1.7103E-5\n1.15\t1.7103E-5\n1.15\t1.7103E-5\n1.16\t1.7102E-5\n1.16\t1.7102E-5\n1.16\t1.7102E-5\n1.16\t1.7102E-5\n1.16\t1.7102E-5\n1.16\t1.7102E-5\n1.16\t1.7102E-5\n1.16\t1.7102E-5\n1.16\t1.7102E-5\n1.16\t1.7102E-5\n1.16\t1.7102E-5\n1.16952\t1.7101E-5\n1.17\t1.7101E-5\n1.17\t1.7101E-5\n1.17\t1.7101E-5\n1.17\t1.7101E-5\n1.17\t1.7101E-5\n1.17\t1.7101E-5\n1.17\t1.7101E-5\n1.17\t1.7101E-5\n1.17\t1.7101E-5\n1.17\t1.7101E-5\n1.17\t1.7101E-5\n1.18\t1.71E-5\n1.18\t1.71E-5\n1.18\t1.71E-5\n1.18\t1.71E-5\n1.18\t1.71E-5\n1.18\t1.71E-5\n1.18\t1.71E-5\n1.18\t1.71E-5\n1.18\t1.71E-5\n1.18\t1.71E-5\n1.18\t1.71E-5\n1.1896\t1.7099E-5\n1.19\t1.7099E-5\n1.19\t1.7099E-5\n1.19\t1.7099E-5\n1.19\t1.7099E-5\n1.19\t1.7099E-5\n1.19\t1.7099E-5\n1.19\t1.7099E-5\n1.19\t1.7099E-5\n1.19\t1.7099E-5\n1.19\t1.7099E-5\n1.19\t1.7099E-5\n1.2\t1.7098E-5\n1.2\t1.7098E-5\n1.2\t1.7098E-5\n1.2\t1.7098E-5\n1.2\t1.7098E-5\n1.2\t1.7098E-5\n1.2\t1.7098E-5\n1.2\t1.7098E-5\n1.2\t1.7098E-5\n1.2\t1.7098E-5\n1.2\t1.7098E-5\n1.21\t1.7097E-5\n1.21\t1.7097E-5\n1.21\t1.7097E-5\n1.21\t1.7097E-5\n1.21\t1.7097E-5\n1.21\t1.7097E-5\n1.21\t1.7097E-5\n1.21\t1.7097E-5\n1.21\t1.7097E-5\n1.21\t1.7097E-5\n1.21\t1.7097E-5\n1.21\t1.7097E-5\n1.22\t1.7096E-5\n1.22\t1.7096E-5\n1.22\t1.7096E-5\n1.22\t1.7096E-5\n1.22\t1.7096E-5\n1.22\t1.7096E-5\n1.22\t1.7096E-5\n1.22\t1.7096E-5\n1.22\t1.7096E-5\n1.22\t1.7096E-5\n1.22\t1.7096E-5\n1.23\t1.7095E-5\n1.23\t1.7095E-5\n1.23\t1.7095E-5\n1.23\t1.7095E-5\n1.23\t1.7095E-5\n1.23\t1.7095E-5\n1.23\t1.7095E-5\n1.23\t1.7095E-5\n1.23\t1.7095E-5\n1.23\t1.7095E-5\n1.23\t1.7095E-5\n1.24\t1.7093E-5\n1.24\t1.7093E-5\n1.24\t1.7093E-5\n1.24\t1.7093E-5\n1.24\t1.7093E-5\n1.24\t1.7093E-5\n1.24\t1.7093E-5\n1.24\t1.7093E-5\n1.24\t1.7093E-5\n1.24\t1.7093E-5\n1.24\t1.7093E-5\n1.25\t1.7092E-5\n1.25\t1.7092E-5\n1.25\t1.7092E-5\n1.25\t1.7092E-5\n1.25\t1.7092E-5\n1.25\t1.7092E-5\n1.25\t1.7092E-5\n1.25\t1.7092E-5\n1.25\t1.7092E-5\n1.25\t1.7092E-5\n1.25\t1.7092E-5\n1.26\t1.7091E-5\n1.26\t1.7091E-5\n1.26\t1.7091E-5\n1.26\t1.7091E-5\n1.26\t1.7091E-5\n1.26\t1.7091E-5\n1.26\t1.7091E-5\n1.26\t1.7091E-5\n1.26\t1.7091E-5\n1.26\t1.7091E-5\n1.26\t1.7091E-5\n1.26948\t1.709E-5\n1.27\t1.709E-5\n1.27\t1.709E-5\n1.27\t1.709E-5\n1.27\t1.709E-5\n1.27\t1.709E-5\n1.27\t1.709E-5\n1.27\t1.709E-5\n1.27\t1.709E-5\n1.27\t1.709E-5\n1.27\t1.709E-5\n1.27\t1.709E-5\n1.28\t1.7089E-5\n1.28\t1.7089E-5\n1.28\t1.7089E-5\n1.28\t1.7089E-5\n1.28\t1.7089E-5\n1.28\t1.7089E-5\n1.28\t1.7089E-5\n1.28\t1.7089E-5\n1.28\t1.7089E-5\n1.28\t1.7089E-5\n1.28\t1.7089E-5\n1.28\t1.7089E-5\n1.29\t1.7088E-5\n1.29\t1.7088E-5\n1.29\t1.7088E-5\n1.29\t1.7088E-5\n1.29\t1.7088E-5\n1.29\t1.7088E-5\n1.29\t1.7088E-5\n1.29\t1.7088E-5\n1.29\t1.7088E-5\n1.29\t1.7088E-5\n1.29\t1.7088E-5\n1.3\t1.7087E-5\n1.3\t1.7087E-5\n1.3\t1.7087E-5\n1.3\t1.7087E-5\n1.3\t1.7087E-5\n1.3\t1.7087E-5\n1.3\t1.7087E-5\n1.3\t1.7087E-5\n1.3\t1.7087E-5\n1.3\t1.7087E-5\n1.3\t1.7087E-5\n1.31\t1.7085E-5\n1.31\t1.7085E-5\n1.31\t1.7085E-5\n1.31\t1.7085E-5\n1.31\t1.7085E-5\n1.31\t1.7085E-5\n1.31\t1.7085E-5\n1.31\t1.7085E-5\n1.31\t1.7085E-5\n1.31\t1.7085E-5\n1.31\t1.7085E-5\n1.31\t1.7085E-5\n1.32\t1.7084E-5\n1.32\t1.7084E-5\n1.32\t1.7084E-5\n1.32\t1.7084E-5\n1.32\t1.7084E-5\n1.32\t1.7084E-5\n1.32\t1.7084E-5\n1.32\t1.7084E-5\n1.32\t1.7084E-5\n1.32\t1.7084E-5\n1.32\t1.7084E-5\n1.32952\t1.7083E-5\n1.33\t1.7083E-5\n1.33\t1.7083E-5\n1.33\t1.7083E-5\n1.33\t1.7083E-5\n1.33\t1.7083E-5\n1.33\t1.7083E-5\n1.33\t1.7083E-5\n1.33\t1.7083E-5\n1.33\t1.7083E-5\n1.33\t1.7083E-5\n1.33\t1.7083E-5\n1.34\t1.7082E-5\n1.34\t1.7082E-5\n1.34\t1.7082E-5\n1.34\t1.7082E-5\n1.34\t1.7082E-5\n1.34\t1.7082E-5\n1.34\t1.7082E-5\n1.34\t1.7082E-5\n1.34\t1.7082E-5\n1.34\t1.7082E-5\n1.34\t1.7082E-5\n1.34\t1.7082E-5\n1.35\t1.7081E-5\n1.35\t1.7081E-5\n1.35\t1.7081E-5\n1.35\t1.7081E-5\n1.35\t1.7081E-5\n1.35\t1.7081E-5\n1.35\t1.7081E-5\n1.35\t1.7081E-5\n1.35\t1.7081E-5\n1.35\t1.7081E-5\n1.35\t1.7081E-5\n1.35\t1.7081E-5\n1.36\t1.7079E-5\n1.36\t1.7079E-5\n1.36\t1.7079E-5\n1.36\t1.7079E-5\n1.36\t1.7079E-5\n1.36\t1.7079E-5\n1.36\t1.7079E-5\n1.36\t1.7079E-5\n1.36\t1.7079E-5\n1.36\t1.7079E-5\n1.36\t1.7079E-5\n1.37\t1.7078E-5\n1.37\t1.7078E-5\n1.37\t1.7078E-5\n1.37\t1.7078E-5\n1.37\t1.7078E-5\n1.37\t1.7078E-5\n1.37\t1.7078E-5\n1.37\t1.7078E-5\n1.37\t1.7078E-5\n1.37\t1.7078E-5\n1.37\t1.7078E-5\n1.38\t1.7077E-5\n1.38\t1.7077E-5\n1.38\t1.7077E-5\n1.38\t1.7077E-5\n1.38\t1.7077E-5\n1.38\t1.7077E-5\n1.38\t1.7077E-5\n1.38\t1.7077E-5\n1.38\t1.7077E-5\n1.38\t1.7077E-5\n1.38\t1.7077E-5\n1.38948\t1.7076E-5\n1.39\t1.7076E-5\n1.39\t1.7076E-5\n1.39\t1.7076E-5\n1.39\t1.7076E-5\n1.39\t1.7076E-5\n1.39\t1.7076E-5\n1.39\t1.7076E-5\n1.39\t1.7076E-5\n1.39\t1.7076E-5\n1.39\t1.7076E-5\n1.39\t1.7076E-5\n1.3996\t1.7074E-5\n1.4\t1.7074E-5\n1.4\t1.7074E-5\n1.4\t1.7074E-5\n1.4\t1.7074E-5\n1.4\t1.7074E-5\n1.4\t1.7074E-5\n1.4\t1.7074E-5\n1.4\t1.7074E-5\n1.4\t1.7074E-5\n1.4\t1.7074E-5\n1.4\t1.7074E-5\n1.41\t1.7073E-5\n1.41\t1.7073E-5\n1.41\t1.7073E-5\n1.41\t1.7073E-5\n1.41\t1.7073E-5\n1.41\t1.7073E-5\n1.41\t1.7073E-5\n1.41\t1.7073E-5\n1.41\t1.7073E-5\n1.41\t1.7073E-5\n1.41\t1.7073E-5\n1.42\t1.7072E-5\n1.42\t1.7072E-5\n1.42\t1.7072E-5\n1.42\t1.7072E-5\n1.42\t1.7072E-5\n1.42\t1.7072E-5\n1.42\t1.7072E-5\n1.42\t1.7072E-5\n1.42\t1.7072E-5\n1.42\t1.7072E-5\n1.42\t1.7072E-5\n1.42952\t1.707E-5\n1.43\t1.707E-5\n1.43\t1.707E-5\n1.43\t1.707E-5\n1.43\t1.707E-5\n1.43\t1.707E-5\n1.43\t1.707E-5\n1.43\t1.707E-5\n1.43\t1.707E-5\n1.43\t1.707E-5\n1.43\t1.707E-5\n1.43\t1.707E-5\n1.44\t1.7069E-5\n1.44\t1.7069E-5\n1.44\t1.7069E-5\n1.44\t1.7069E-5\n1.44\t1.7069E-5\n1.44\t1.7069E-5\n1.44\t1.7069E-5\n1.44\t1.7069E-5\n1.44\t1.7069E-5\n1.44\t1.7069E-5\n1.44\t1.7069E-5\n1.45\t1.7068E-5\n1.45\t1.7068E-5\n1.45\t1.7068E-5\n1.45\t1.7068E-5\n1.45\t1.7068E-5\n1.45\t1.7068E-5\n1.45\t1.7068E-5\n1.45\t1.7068E-5\n1.45\t1.7068E-5\n1.45\t1.7068E-5\n1.45\t1.7068E-5\n1.45956\t1.7066E-5\n1.46\t1.7066E-5\n1.46\t1.7066E-5\n1.46\t1.7066E-5\n1.46\t1.7066E-5\n1.46\t1.7066E-5\n1.46\t1.7066E-5\n1.46\t1.7066E-5\n1.46\t1.7066E-5\n1.46\t1.7066E-5\n1.46\t1.7066E-5\n1.46\t1.7066E-5\n1.47\t1.7065E-5\n1.47\t1.7065E-5\n1.47\t1.7065E-5\n1.47\t1.7065E-5\n1.47\t1.7065E-5\n1.47\t1.7065E-5\n1.47\t1.7065E-5\n1.47\t1.7065E-5\n1.47\t1.7065E-5\n1.47\t1.7065E-5\n1.47\t1.7065E-5\n1.48\t1.7063E-5\n1.48\t1.7063E-5\n1.48\t1.7063E-5\n1.48\t1.7063E-5\n1.48\t1.7063E-5\n1.48\t1.7063E-5\n1.48\t1.7063E-5\n1.48\t1.7063E-5\n1.48\t1.7063E-5\n1.48\t1.7063E-5\n1.48\t1.7063E-5\n1.49\t1.7062E-5\n1.49\t1.7062E-5\n1.49\t1.7062E-5\n1.49\t1.7062E-5\n1.49\t1.7062E-5\n1.49\t1.7062E-5\n1.49\t1.7062E-5\n1.49\t1.7062E-5\n1.49\t1.7062E-5\n1.49\t1.7062E-5\n1.49\t1.7062E-5\n1.49\t1.7062E-5\n1.5\t1.706E-5\n1.5\t1.706E-5\n1.5\t1.706E-5\n1.5\t1.706E-5\n1.5\t1.706E-5\n1.5\t1.706E-5\n1.5\t1.706E-5\n1.5\t1.706E-5\n1.5\t1.706E-5\n1.5\t1.706E-5\n1.5\t1.706E-5\n1.51\t1.7059E-5\n1.51\t1.7059E-5\n1.51\t1.7059E-5\n1.51\t1.7059E-5\n1.51\t1.7059E-5\n1.51\t1.7059E-5\n1.51\t1.7059E-5\n1.51\t1.7059E-5\n1.51\t1.7059E-5\n1.51\t1.7059E-5\n1.51\t1.7059E-5\n1.51952\t1.7058E-5\n1.52\t1.7058E-5\n1.52\t1.7058E-5\n1.52\t1.7058E-5\n1.52\t1.7058E-5\n1.52\t1.7058E-5\n1.52\t1.7058E-5\n1.52\t1.7058E-5\n1.52\t1.7058E-5\n1.52\t1.7058E-5\n1.52\t1.7058E-5\n1.52\t1.7058E-5\n1.53\t1.7056E-5\n1.53\t1.7056E-5\n1.53\t1.7056E-5\n1.53\t1.7056E-5\n1.53\t1.7056E-5\n1.53\t1.7056E-5\n1.53\t1.7056E-5\n1.53\t1.7056E-5\n1.53\t1.7056E-5\n1.53\t1.7056E-5\n1.53\t1.7056E-5\n1.54\t1.7055E-5\n1.54\t1.7055E-5\n1.54\t1.7055E-5\n1.54\t1.7055E-5\n1.54\t1.7055E-5\n1.54\t1.7055E-5\n1.54\t1.7055E-5\n1.54\t1.7055E-5\n1.54\t1.7055E-5\n1.54\t1.7055E-5\n1.54\t1.7055E-5\n1.55\t1.7053E-5\n1.55\t1.7053E-5\n1.55\t1.7053E-5\n1.55\t1.7053E-5\n1.55\t1.7053E-5\n1.55\t1.7053E-5\n1.55\t1.7053E-5\n1.55\t1.7053E-5\n1.55\t1.7053E-5\n1.55\t1.7053E-5\n1.55\t1.7053E-5\n1.55952\t1.7052E-5\n1.56\t1.7052E-5\n1.56\t1.7052E-5\n1.56\t1.7052E-5\n1.56\t1.7052E-5\n1.56\t1.7052E-5\n1.56\t1.7052E-5\n1.56\t1.7052E-5\n1.56\t1.7052E-5\n1.56\t1.7052E-5\n1.56\t1.7052E-5\n1.56\t1.7052E-5\n1.56948\t1.705E-5\n1.57\t1.705E-5\n1.57\t1.705E-5\n1.57\t1.705E-5\n1.57\t1.705E-5\n1.57\t1.705E-5\n1.57\t1.705E-5\n1.57\t1.705E-5\n1.57\t1.705E-5\n1.57\t1.705E-5\n1.57\t1.705E-5\n1.57\t1.705E-5\n1.58\t1.7049E-5\n1.58\t1.7049E-5\n1.58\t1.7049E-5\n1.58\t1.7049E-5\n1.58\t1.7049E-5\n1.58\t1.7049E-5\n1.58\t1.7049E-5\n1.58\t1.7049E-5\n1.58\t1.7049E-5\n1.58\t1.7049E-5\n1.58\t1.7049E-5\n1.58\t1.7049E-5\n1.63\t1.7041E-5\n1.63\t1.7041E-5\n1.63\t1.7041E-5\n1.63\t1.7041E-5\n1.63\t1.7041E-5\n1.63\t1.7041E-5\n1.63\t1.7041E-5\n1.63\t1.7041E-5\n1.63\t1.7041E-5\n1.63\t1.7041E-5\n1.63\t1.7041E-5\n1.68\t1.7032E-5\n1.68\t1.7032E-5\n1.68\t1.7032E-5\n1.68\t1.7032E-5\n1.68\t1.7032E-5\n1.68\t1.7032E-5\n1.68\t1.7032E-5\n1.68\t1.7032E-5\n1.68\t1.7032E-5\n1.68\t1.7032E-5\n1.68\t1.7032E-5\n1.73\t1.7024E-5\n1.73\t1.7024E-5\n1.73\t1.7024E-5\n1.73\t1.7024E-5\n1.73\t1.7024E-5\n1.73\t1.7024E-5\n1.73\t1.7024E-5\n1.73\t1.7024E-5\n1.73\t1.7024E-5\n1.73\t1.7024E-5\n1.73\t1.7024E-5\n1.78\t1.7015E-5\n1.78\t1.7015E-5\n1.78\t1.7015E-5\n1.78\t1.7015E-5\n1.78\t1.7015E-5\n1.78\t1.7015E-5\n1.78\t1.7015E-5\n1.78\t1.7015E-5\n1.78\t1.7015E-5\n1.78\t1.7015E-5\n1.78\t1.7015E-5\n1.78\t1.7015E-5\n1.83\t1.7006E-5\n1.83\t1.7006E-5\n1.83\t1.7006E-5\n1.83\t1.7006E-5\n1.83\t1.7006E-5\n1.83\t1.7006E-5\n1.83\t1.7006E-5\n1.83\t1.7006E-5\n1.83\t1.7006E-5\n1.83\t1.7006E-5\n1.83\t1.7006E-5\n1.88\t1.6996E-5\n1.88\t1.6996E-5\n1.88\t1.6996E-5\n1.88\t1.6996E-5\n1.88\t1.6996E-5\n1.88\t1.6996E-5\n1.88\t1.6996E-5\n1.88\t1.6996E-5\n1.88\t1.6996E-5\n1.88\t1.6996E-5\n1.88\t1.6996E-5\n1.93\t1.6987E-5\n1.93\t1.6987E-5\n1.93\t1.6987E-5\n1.93\t1.6987E-5\n1.93\t1.6987E-5\n1.93\t1.6987E-5\n1.93\t1.6987E-5\n1.93\t1.6987E-5\n1.93\t1.6987E-5\n1.93\t1.6987E-5\n1.93\t1.6987E-5\n1.98\t1.6976E-5\n1.98\t1.6976E-5\n1.98\t1.6976E-5\n1.98\t1.6976E-5\n1.98\t1.6976E-5\n1.98\t1.6976E-5\n1.98\t1.6976E-5\n1.98\t1.6976E-5\n1.98\t1.6976E-5\n1.98\t1.6976E-5\n1.98\t1.6976E-5\n1.98\t1.6976E-5\n2.03\t1.6966E-5\n2.03\t1.6966E-5\n2.03\t1.6966E-5\n2.03\t1.6966E-5\n2.03\t1.6966E-5\n2.03\t1.6966E-5\n2.03\t1.6966E-5\n2.03\t1.6966E-5\n2.03\t1.6966E-5\n2.03\t1.6966E-5\n2.03\t1.6966E-5\n2.08\t1.6955E-5\n2.08\t1.6955E-5\n2.08\t1.6955E-5\n2.08\t1.6955E-5\n2.08\t1.6955E-5\n2.08\t1.6955E-5\n2.08\t1.6955E-5\n2.08\t1.6955E-5\n2.08\t1.6955E-5\n2.08\t1.6955E-5\n2.08\t1.6955E-5\n2.08\t1.6955E-5\n2.13\t1.6944E-5\n2.13\t1.6944E-5\n2.13\t1.6944E-5\n2.13\t1.6944E-5\n2.13\t1.6944E-5\n2.13\t1.6944E-5\n2.13\t1.6944E-5\n2.13\t1.6944E-5\n2.13\t1.6944E-5\n2.13\t1.6944E-5\n2.13\t1.6944E-5\n2.17948\t1.6933E-5\n2.18\t1.6932E-5\n2.18\t1.6932E-5\n2.18\t1.6932E-5\n2.18\t1.6932E-5\n2.18\t1.6932E-5\n2.18\t1.6932E-5\n2.18\t1.6932E-5\n2.18\t1.6932E-5\n2.18\t1.6932E-5\n2.18\t1.6932E-5\n2.18\t1.6932E-5\n2.23\t1.6921E-5\n2.23\t1.6921E-5\n2.23\t1.6921E-5\n2.23\t1.6921E-5\n2.23\t1.6921E-5\n2.23\t1.6921E-5\n2.23\t1.6921E-5\n2.23\t1.6921E-5\n2.23\t1.6921E-5\n2.23\t1.6921E-5\n2.23\t1.6921E-5\n2.23\t1.6921E-5\n2.28\t1.6909E-5\n2.28\t1.6909E-5\n2.28\t1.6909E-5\n2.28\t1.6909E-5\n2.28\t1.6909E-5\n2.28\t1.6909E-5\n2.28\t1.6909E-5\n2.28\t1.6909E-5\n2.28\t1.6909E-5\n2.28\t1.6909E-5\n2.28\t1.6909E-5\n2.28\t1.6909E-5\n2.33\t1.6896E-5\n2.33\t1.6896E-5\n2.33\t1.6896E-5\n2.33\t1.6896E-5\n2.33\t1.6896E-5\n2.33\t1.6896E-5\n2.33\t1.6896E-5\n2.33\t1.6896E-5\n2.33\t1.6896E-5\n2.33\t1.6896E-5\n2.33\t1.6896E-5\n2.3796\t1.6883E-5\n2.38\t1.6883E-5\n2.38\t1.6883E-5\n2.38\t1.6883E-5\n2.38\t1.6883E-5\n2.38\t1.6883E-5\n2.38\t1.6883E-5\n2.38\t1.6883E-5\n2.38\t1.6883E-5\n2.38\t1.6883E-5\n2.38\t1.6883E-5\n2.38\t1.6883E-5\n2.43\t1.687E-5\n2.43\t1.687E-5\n2.43\t1.687E-5\n2.43\t1.687E-5\n2.43\t1.687E-5\n2.43\t1.687E-5\n2.43\t1.687E-5\n2.43\t1.687E-5\n2.43\t1.687E-5\n2.43\t1.687E-5\n2.43\t1.687E-5\n2.48\t1.6857E-5\n2.48\t1.6857E-5\n2.48\t1.6857E-5\n2.48\t1.6857E-5\n2.48\t1.6857E-5\n2.48\t1.6857E-5\n2.48\t1.6857E-5\n2.48\t1.6857E-5\n2.48\t1.6857E-5\n2.48\t1.6857E-5\n2.48\t1.6857E-5\n2.52952\t1.6843E-5\n2.53\t1.6843E-5\n2.53\t1.6843E-5\n2.53\t1.6843E-5\n2.53\t1.6843E-5\n2.53\t1.6843E-5\n2.53\t1.6843E-5\n2.53\t1.6843E-5\n2.53\t1.6843E-5\n2.53\t1.6843E-5\n2.53\t1.6843E-5\n2.53\t1.6843E-5\n2.58\t1.6829E-5\n2.58\t1.6829E-5\n2.58\t1.6829E-5\n2.58\t1.6829E-5\n2.58\t1.6829E-5\n2.58\t1.6829E-5\n2.58\t1.6829E-5\n2.58\t1.6829E-5\n2.58\t1.6829E-5\n2.58\t1.6829E-5\n2.58\t1.6829E-5\n2.63\t1.6814E-5\n2.63\t1.6814E-5\n2.63\t1.6814E-5\n2.63\t1.6814E-5\n2.63\t1.6814E-5\n2.63\t1.6814E-5\n2.63\t1.6814E-5\n2.63\t1.6814E-5\n2.63\t1.6814E-5\n2.63\t1.6814E-5\n2.63\t1.6814E-5\n2.67956\t1.68E-5\n2.68\t1.68E-5\n2.68\t1.68E-5\n2.68\t1.68E-5\n2.68\t1.68E-5\n2.68\t1.68E-5\n2.68\t1.68E-5\n2.68\t1.68E-5\n2.68\t1.68E-5\n2.68\t1.68E-5\n2.68\t1.68E-5\n2.68\t1.68E-5\n2.73\t1.6785E-5\n2.73\t1.6785E-5\n2.73\t1.6785E-5\n2.73\t1.6785E-5\n2.73\t1.6785E-5\n2.73\t1.6785E-5\n2.73\t1.6785E-5\n2.73\t1.6785E-5\n2.73\t1.6785E-5\n2.73\t1.6785E-5\n2.73\t1.6785E-5\n2.78\t1.6769E-5\n2.78\t1.6769E-5\n2.78\t1.6769E-5\n2.78\t1.6769E-5\n2.78\t1.6769E-5\n2.78\t1.6769E-5\n2.78\t1.6769E-5\n2.78\t1.6769E-5\n2.78\t1.6769E-5\n2.78\t1.6769E-5\n2.78\t1.6769E-5\n2.78\t1.6769E-5\n2.83\t1.6754E-5\n2.83\t1.6754E-5\n2.83\t1.6754E-5\n2.83\t1.6754E-5\n2.83\t1.6754E-5\n2.83\t1.6754E-5\n2.83\t1.6754E-5\n2.83\t1.6754E-5\n2.83\t1.6754E-5\n2.83\t1.6754E-5\n2.83\t1.6754E-5\n2.88\t1.6738E-5\n2.88\t1.6738E-5\n2.88\t1.6738E-5\n2.88\t1.6738E-5\n2.88\t1.6738E-5\n2.88\t1.6738E-5\n2.88\t1.6738E-5\n2.88\t1.6738E-5\n2.88\t1.6738E-5\n2.88\t1.6738E-5\n2.88\t1.6738E-5\n2.88\t1.6738E-5\n2.93\t1.6721E-5\n2.93\t1.6721E-5\n2.93\t1.6721E-5\n2.93\t1.6721E-5\n2.93\t1.6721E-5\n2.93\t1.6721E-5\n2.93\t1.6721E-5\n2.93\t1.6721E-5\n2.93\t1.6721E-5\n2.93\t1.6721E-5\n2.93\t1.6721E-5\n2.93\t1.6721E-5\n2.98\t1.6704E-5\n2.98\t1.6704E-5\n2.98\t1.6704E-5\n2.98\t1.6704E-5\n2.98\t1.6704E-5\n2.98\t1.6704E-5\n2.98\t1.6704E-5\n2.98\t1.6704E-5\n2.98\t1.6704E-5\n2.98\t1.6704E-5\n2.98\t1.6704E-5\n2.98\t1.6704E-5\n2.98\t1.6704E-5\n2.98\t1.6704E-5\n2.98\t1.6704E-5\n2.98\t1.6704E-5\n2.98\t1.6704E-5\n2.98\t1.6704E-5\n2.98\t1.6704E-5\n2.98\t1.6704E-5\n2.98\t1.6704E-5\n2.98\t1.6704E-5\n2.98\t1.6704E-5\n2.98\t1.6704E-5\n2.98\t1.6704E-5\n2.98\t1.6704E-5\n2.98\t1.6704E-5\n2.98\t1.6704E-5\n2.98\t1.6704E-5\n2.98\t1.6704E-5\n2.98\t1.6704E-5\n2.98\t1.6704E-5\n2.98\t1.6704E-5\n2.98\t1.6704E-5\n2.98\t1.6704E-5\n2.98\t1.6704E-5\n2.98\t1.6704E-5\n2.98\t1.6704E-5\n2.98\t1.6704E-5\n2.98\t1.6704E-5\n2.98\t1.6704E-5\n2.98\t1.6704E-5\n2.98\t1.6704E-5\n2.98\t1.6704E-5\n2.98\t1.6704E-5\n2.98\t1.6704E-5\n2.98\t1.6704E-5\n2.98145\t1.6704E-5\n2.98441\t1.6703E-5\n2.98633\t1.6702E-5\n2.98885\t1.6701E-5\n2.99181\t1.67E-5\n2.99421\t1.67E-5\n2.99709\t1.6699E-5\n2.99913\t1.6698E-5\n3.00157\t1.6697E-5\n3.00445\t1.6696E-5\n3.00689\t1.6695E-5\n3.00893\t1.6695E-5\n3.01149\t1.6694E-5\n3.01577\t1.6692E-5\n3.01766\t1.6692E-5\n3.02133\t1.669E-5\n3.0231\t1.669E-5\n3.02653\t1.6689E-5\n3.0287\t1.6688E-5\n3.03094\t1.6687E-5\n3.0329\t1.6686E-5\n3.03678\t1.6685E-5\n3.03774\t1.6685E-5\n3.04014\t1.6684E-5\n3.04342\t1.6683E-5\n3.04586\t1.6682E-5\n3.0483\t1.6681E-5\n3.05054\t1.668E-5\n3.0531\t1.6679E-5\n3.05546\t1.6679E-5\n3.0593\t1.6677E-5\n3.0603\t1.6677E-5\n3.06234\t1.6676E-5\n3.06558\t1.6675E-5\n3.0681\t1.6674E-5\n3.07058\t1.6673E-5\n3.07494\t1.6672E-5\n3.0759\t1.6672E-5\n3.07774\t1.6671E-5\n3.08222\t1.6669E-5\n3.08322\t1.6669E-5\n3.08526\t1.6668E-5\n3.08714\t1.6668E-5\n3.08922\t1.6667E-5\n3.09222\t1.6666E-5\n3.0947\t1.6665E-5\n3.09698\t1.6664E-5\n3.09894\t1.6663E-5\n3.1015\t1.6663E-5\n3.10466\t1.6661E-5\n3.10706\t1.6661E-5\n3.10898\t1.666E-5\n3.11158\t1.6659E-5\n3.11406\t1.6658E-5\n3.11686\t1.6657E-5\n3.11942\t1.6656E-5\n3.12138\t1.6655E-5\n3.12418\t1.6654E-5\n3.1267\t1.6654E-5\n3.1297\t1.6653E-5\n3.13222\t1.6652E-5\n3.13466\t1.6651E-5\n3.1365\t1.665E-5\n3.1395\t1.6649E-5\n3.14142\t1.6648E-5\n3.14482\t1.6647E-5\n3.1467\t1.6646E-5\n3.14974\t1.6645E-5\n3.15214\t1.6644E-5\n3.15402\t1.6644E-5\n3.15762\t1.6643E-5\n3.15951\t1.6642E-5\n3.16142\t1.6641E-5\n3.1639\t1.664E-5\n3.16678\t1.6639E-5\n3.17019\t1.6638E-5\n3.17179\t1.6637E-5\n3.17479\t1.6636E-5\n3.17719\t1.6635E-5\n3.17919\t1.6635E-5\n3.18263\t1.6633E-5\n3.18451\t1.6633E-5\n3.18647\t1.6632E-5\n3.18891\t1.6631E-5\n3.19187\t1.663E-5\n3.19539\t1.6629E-5\n3.19719\t1.6628E-5\n3.19907\t1.6627E-5\n3.20159\t1.6627E-5\n3.20455\t1.6625E-5\n3.20643\t1.6625E-5\n3.20895\t1.6624E-5\n3.21187\t1.6623E-5\n3.21427\t1.6622E-5\n3.21623\t1.6621E-5\n3.21919\t1.662E-5\n3.22155\t1.6619E-5\n3.22459\t1.6618E-5\n3.22699\t1.6617E-5\n3.22887\t1.6616E-5\n3.23183\t1.6615E-5\n3.23431\t1.6614E-5\n3.23627\t1.6614E-5\n3.23987\t1.6612E-5\n3.24171\t1.6612E-5\n3.24463\t1.6611E-5\n3.24727\t1.661E-5\n3.24911\t1.6609E-5\n3.25255\t1.6608E-5\n3.25447\t1.6607E-5\n3.25707\t1.6606E-5\n3.25939\t1.6605E-5\n3.26155\t1.6604E-5\n3.26403\t1.6603E-5\n3.26691\t1.6602E-5\n3.26887\t1.6602E-5\n3.27135\t1.6601E-5\n3.27427\t1.66E-5\n3.27679\t1.6599E-5\n3.27935\t1.6598E-5\n3.28239\t1.6597E-5\n3.28435\t1.6596E-5\n3.28632\t1.6595E-5\n3.28964\t1.6594E-5\n3.29159\t1.6593E-5\n3.29508\t1.6592E-5\n3.29691\t1.6591E-5\n3.29888\t1.659E-5\n3.30143\t1.6589E-5\n3.30383\t1.6588E-5\n3.30736\t1.6587E-5\n3.30895\t1.6586E-5\n3.3118\t1.6585E-5\n3.31388\t1.6585E-5\n3.3168\t1.6583E-5\n3.31916\t1.6583E-5\n3.3222\t1.6581E-5\n3.32524\t1.658E-5\n3.32712\t1.658E-5\n3.32904\t1.6579E-5\n3.33156\t1.6578E-5\n3.33396\t1.6577E-5\n3.33828\t1.6575E-5\n3.33916\t1.6575E-5\n3.34212\t1.6574E-5\n3.34476\t1.6573E-5\n3.3466\t1.6572E-5\n3.34904\t1.6571E-5\n3.35156\t1.657E-5\n3.35456\t1.6569E-5\n3.35696\t1.6568E-5\n3.35868\t1.6567E-5\n3.3616\t1.6566E-5\n3.36452\t1.6565E-5\n3.36664\t1.6564E-5\n3.36904\t1.6563E-5\n3.37208\t1.6562E-5\n3.37516\t1.6561E-5\n3.37664\t1.656E-5\n3.37952\t1.6559E-5\n3.38212\t1.6558E-5\n3.384\t1.6558E-5\n3.38744\t1.6556E-5\n3.3894\t1.6555E-5\n3.3914\t1.6555E-5\n3.39476\t1.6553E-5\n3.39676\t1.6553E-5\n3.4002\t1.6551E-5\n3.40204\t1.6551E-5\n3.40396\t1.655E-5\n3.40652\t1.6549E-5\n3.4094\t1.6548E-5\n3.4114\t1.6547E-5\n3.41456\t1.6546E-5\n3.41652\t1.6545E-5\n3.41904\t1.6544E-5\n3.42208\t1.6543E-5\n3.4248\t1.6542E-5\n3.42736\t1.6541E-5\n3.4292\t1.654E-5\n3.43213\t1.6539E-5\n3.43409\t1.6538E-5\n3.43713\t1.6537E-5\n3.43912\t1.6536E-5\n3.44221\t1.6535E-5\n3.44461\t1.6534E-5\n3.44653\t1.6533E-5\n3.44961\t1.6532E-5\n3.45209\t1.6531E-5\n3.45393\t1.653E-5\n3.45749\t1.6529E-5\n3.45897\t1.6528E-5\n3.46177\t1.6527E-5\n3.46425\t1.6526E-5\n3.46717\t1.6525E-5\n3.46961\t1.6524E-5\n3.47157\t1.6523E-5\n3.47457\t1.6522E-5\n3.47697\t1.6521E-5\n3.47893\t1.652E-5\n3.48237\t1.6519E-5\n3.48393\t1.6518E-5\n3.48689\t1.6517E-5\n3.48937\t1.6516E-5\n3.49181\t1.6515E-5\n3.49441\t1.6514E-5\n3.49637\t1.6513E-5\n3.49945\t1.6512E-5\n3.50181\t1.6511E-5\n3.50473\t1.651E-5\n3.50709\t1.6509E-5\n3.50909\t1.6508E-5\n3.51209\t1.6507E-5\n3.51485\t1.6505E-5\n3.51689\t1.6505E-5\n3.51893\t1.6504E-5\n3.52217\t1.6502E-5\n3.52429\t1.6502E-5\n3.52673\t1.6501E-5\n3.52957\t1.6499E-5\n3.53329\t1.6498E-5\n3.53417\t1.6498E-5\n3.53709\t1.6496E-5\n3.53965\t1.6495E-5\n3.54157\t1.6494E-5\n3.54465\t1.6493E-5\n3.54729\t1.6492E-5\n3.54917\t1.6491E-5\n3.55169\t1.649E-5\n3.55425\t1.6489E-5\n3.55777\t1.6488E-5\n3.55925\t1.6487E-5\n3.56233\t1.6486E-5\n3.56473\t1.6485E-5\n3.56661\t1.6484E-5\n3.5709\t1.6482E-5\n3.57246\t1.6482E-5\n3.57578\t1.648E-5\n3.57774\t1.648E-5\n3.58082\t1.6478E-5\n3.5817\t1.6478E-5\n3.58426\t1.6477E-5\n3.58674\t1.6476E-5\n3.59022\t1.6474E-5\n3.5923\t1.6473E-5\n3.59414\t1.6473E-5\n3.59666\t1.6472E-5\n3.59982\t1.647E-5\n3.60174\t1.647E-5\n3.60414\t1.6469E-5\n3.60722\t1.6467E-5\n3.60966\t1.6466E-5\n3.61154\t1.6465E-5\n3.61462\t1.6464E-5\n3.61702\t1.6463E-5\n3.6189\t1.6462E-5\n3.6229\t1.6461E-5\n3.62438\t1.646E-5\n3.62686\t1.6459E-5\n3.6293\t1.6458E-5\n3.63186\t1.6457E-5\n3.6339\t1.6456E-5\n3.63694\t1.6455E-5\n3.6389\t1.6454E-5\n3.64186\t1.6453E-5\n3.64446\t1.6452E-5\n3.64694\t1.6451E-5\n3.6497\t1.6449E-5\n3.65222\t1.6448E-5\n3.6541\t1.6447E-5\n3.65698\t1.6446E-5\n3.65962\t1.6445E-5\n3.6615\t1.6444E-5\n3.66498\t1.6443E-5\n3.66694\t1.6442E-5\n3.66894\t1.6441E-5\n3.67102\t1.644E-5\n3.6749\t1.6439E-5\n3.67682\t1.6438E-5\n3.67966\t1.6437E-5\n3.68174\t1.6436E-5\n3.68414\t1.6435E-5\n3.68706\t1.6433E-5\n3.68966\t1.6432E-5\n3.69154\t1.6431E-5\n3.69443\t1.643E-5\n3.69694\t1.6429E-5\n3.69854\t1.6428E-5\n3.70191\t1.6427E-5\n3.70495\t1.6426E-5\n3.70643\t1.6425E-5\n3.70935\t1.6424E-5\n3.71267\t1.6422E-5\n3.71603\t1.6421E-5\n3.71835\t1.642E-5\n3.72139\t1.6419E-5\n3.72283\t1.6418E-5\n3.72675\t1.6416E-5\n3.72815\t1.6416E-5\n3.73107\t1.6414E-5\n3.73371\t1.6413E-5\n3.73539\t1.6412E-5\n3.73783\t1.6411E-5\n3.74223\t1.6409E-5\n3.74307\t1.6409E-5\n3.74595\t1.6408E-5\n3.74939\t1.6406E-5\n3.75031\t1.6406E-5\n3.75315\t1.6405E-5\n3.75591\t1.6403E-5\n3.75843\t1.6402E-5\n3.76027\t1.6402E-5\n3.76299\t1.64E-5\n3.76547\t1.6399E-5\n3.76839\t1.6398E-5\n3.77179\t1.6397E-5\n3.77275\t1.6396E-5\n3.77535\t1.6395E-5\n3.77671\t1.6394E-5\n3.77975\t1.6393E-5\n3.78163\t1.6392E-5\n3.78367\t1.6391E-5\n3.78887\t1.6389E-5\n3.79023\t1.6388E-5\n3.79415\t1.6387E-5\n3.79511\t1.6386E-5\n3.79827\t1.6385E-5\n3.79911\t1.6384E-5\n3.80211\t1.6383E-5\n3.80451\t1.6382E-5\n3.80639\t1.6381E-5\n3.80991\t1.638E-5\n3.81175\t1.6379E-5\n3.81475\t1.6377E-5\n3.81739\t1.6376E-5\n3.81923\t1.6375E-5\n3.82263\t1.6374E-5\n3.82471\t1.6373E-5\n3.82659\t1.6372E-5\n3.82899\t1.6371E-5\n3.83152\t1.637E-5\n3.835\t1.6368E-5\n3.83688\t1.6368E-5\n3.83996\t1.6366E-5\n3.8414\t1.6366E-5\n3.84419\t1.6364E-5\n3.84788\t1.6363E-5\n3.8498\t1.6362E-5\n3.85168\t1.6361E-5\n3.85416\t1.636E-5\n3.85664\t1.6359E-5\n3.86008\t1.6357E-5\n3.86208\t1.6356E-5\n3.864\t1.6355E-5\n3.867\t1.6354E-5\n3.86896\t1.6353E-5\n3.87244\t1.6352E-5\n3.87392\t1.6351E-5\n3.87696\t1.6349E-5\n3.87904\t1.6349E-5\n3.882\t1.6347E-5\n3.88444\t1.6346E-5\n3.88656\t1.6345E-5\n3.8894\t1.6344E-5\n3.892\t1.6343E-5\n3.894\t1.6342E-5\n3.89652\t1.6341E-5\n3.899\t1.6339E-5\n3.902\t1.6338E-5\n3.904\t1.6337E-5\n3.90704\t1.6336E-5\n3.909\t1.6335E-5\n3.91136\t1.6334E-5\n3.91436\t1.6332E-5\n3.91688\t1.6331E-5\n3.91972\t1.633E-5\n3.92164\t1.6329E-5\n3.92404\t1.6328E-5\n3.92692\t1.6327E-5\n3.92912\t1.6326E-5\n3.93156\t1.6324E-5\n3.9344\t1.6323E-5\n3.93696\t1.6322E-5\n3.93892\t1.6321E-5\n3.9418\t1.632E-5\n3.945\t1.6318E-5\n3.9468\t1.6317E-5\n3.9492\t1.6316E-5\n3.9518\t1.6315E-5\n3.95424\t1.6314E-5\n3.95704\t1.6313E-5\n3.959\t1.6312E-5\n3.96144\t1.6311E-5\n3.96429\t1.6309E-5\n3.9668\t1.6308E-5\n3.96973\t1.6307E-5\n3.97168\t1.6306E-5\n3.97429\t1.6305E-5\n3.9764\t1.6304E-5\n3.97933\t1.6302E-5\n3.98329\t1.63E-5\n3.98473\t1.63E-5\n3.98713\t1.6299E-5\n3.98909\t1.6298E-5\n3.99225\t1.6296E-5\n3.99417\t1.6295E-5\n3.99721\t1.6294E-5\n3.99957\t1.6293E-5\n4.00145\t1.6292E-5\n4.00565\t1.629E-5\n4.00833\t1.6289E-5\n4.00921\t1.6288E-5\n4.01173\t1.6287E-5\n4.01465\t1.6286E-5\n4.01653\t1.6285E-5\n4.01901\t1.6284E-5\n4.02193\t1.6282E-5\n4.02429\t1.6281E-5\n4.02741\t1.628E-5\n4.02889\t1.6279E-5\n4.03213\t1.6277E-5\n4.03493\t1.6276E-5\n4.03729\t1.6275E-5\n4.03917\t1.6274E-5\n4.04281\t1.6272E-5\n4.04389\t1.6272E-5\n4.04673\t1.627E-5\n4.04929\t1.6269E-5\n4.05221\t1.6268E-5\n4.05409\t1.6267E-5\n4.05665\t1.6266E-5\n4.05921\t1.6264E-5\n4.06181\t1.6263E-5\n4.06493\t1.6262E-5\n4.06677\t1.6261E-5\n4.06917\t1.626E-5\n4.07225\t1.6258E-5\n4.07469\t1.6257E-5\n4.07657\t1.6256E-5\n4.07945\t1.6255E-5\n4.08153\t1.6254E-5\n4.08441\t1.6252E-5\n4.08749\t1.6251E-5\n4.08937\t1.625E-5\n4.09221\t1.6249E-5\n4.09481\t1.6247E-5\n4.09669\t1.6246E-5\n4.10014\t1.6245E-5\n4.1029\t1.6243E-5\n4.10573\t1.6242E-5\n4.1091\t1.624E-5\n4.1103\t1.624E-5\n4.11317\t1.6238E-5\n4.11598\t1.6237E-5\n4.11802\t1.6236E-5\n4.12142\t1.6234E-5\n4.12434\t1.6233E-5\n4.1253\t1.6233E-5\n4.12874\t1.6231E-5\n4.12958\t1.6231E-5\n4.13334\t1.6229E-5\n4.1357\t1.6228E-5\n4.13962\t1.6226E-5\n4.1405\t1.6225E-5\n4.1429\t1.6224E-5\n4.14682\t1.6222E-5\n4.14778\t1.6222E-5\n4.15082\t1.622E-5\n4.15314\t1.6219E-5\n4.15562\t1.6218E-5\n4.15778\t1.6217E-5\n4.16166\t1.6215E-5\n4.1627\t1.6214E-5\n4.16578\t1.6213E-5\n4.16666\t1.6212E-5\n4.17022\t1.6211E-5\n4.17214\t1.621E-5\n4.17402\t1.6209E-5\n4.17658\t1.6207E-5\n4.17958\t1.6206E-5\n4.18146\t1.6205E-5\n4.18398\t1.6204E-5\n4.18694\t1.6202E-5\n4.18934\t1.6201E-5\n4.19242\t1.62E-5\n4.19394\t1.6199E-5\n4.19642\t1.6198E-5\n4.20018\t1.6196E-5\n4.2031\t1.6194E-5\n4.20694\t1.6192E-5\n4.2079\t1.6192E-5\n4.2103\t1.6191E-5\n4.21286\t1.6189E-5\n4.21606\t1.6188E-5\n4.21834\t1.6187E-5\n4.22082\t1.6185E-5\n4.2239\t1.6184E-5\n4.22574\t1.6183E-5\n4.2281\t1.6182E-5\n4.23091\t1.618E-5\n4.23282\t1.6179E-5\n4.23638\t1.6178E-5\n4.23807\t1.6177E-5\n4.24094\t1.6175E-5\n4.24319\t1.6174E-5\n4.24547\t1.6173E-5\n4.24835\t1.6172E-5\n4.25067\t1.6171E-5\n4.25267\t1.617E-5\n4.25547\t1.6168E-5\n4.25991\t1.6166E-5\n4.26083\t1.6165E-5\n4.26275\t1.6164E-5\n4.26671\t1.6162E-5\n4.26767\t1.6162E-5\n4.27075\t1.616E-5\n4.27423\t1.6159E-5\n4.27523\t1.6158E-5\n4.27671\t1.6157E-5\n4.27911\t1.6156E-5\n4.28283\t1.6154E-5\n4.28615\t1.6153E-5\n4.28843\t1.6151E-5\n4.29095\t1.615E-5\n4.29335\t1.6149E-5\n4.29567\t1.6148E-5\n4.29827\t1.6146E-5\n4.30059\t1.6145E-5\n4.30447\t1.6143E-5\n4.30583\t1.6143E-5\n4.30727\t1.6142E-5\n4.30915\t1.6141E-5\n4.31171\t1.614E-5\n4.31415\t1.6138E-5\n4.31703\t1.6137E-5\n4.31955\t1.6136E-5\n4.32151\t1.6135E-5\n4.32451\t1.6133E-5\n4.32695\t1.6132E-5\n4.32891\t1.6131E-5\n4.33187\t1.6129E-5\n4.33559\t1.6127E-5\n4.33895\t1.6126E-5\n4.34175\t1.6124E-5\n4.34291\t1.6124E-5\n4.34515\t1.6122E-5\n4.34955\t1.612E-5\n4.35047\t1.612E-5\n4.35387\t1.6118E-5\n4.35671\t1.6116E-5\n4.35779\t1.6116E-5\n4.35931\t1.6115E-5\n4.36175\t1.6114E-5\n4.36479\t1.6112E-5\n4.36715\t1.6111E-5\n4.36903\t1.611E-5\n4.37199\t1.6109E-5\n4.37456\t1.6107E-5\n4.37643\t1.6106E-5\n4.38007\t1.6104E-5\n4.38196\t1.6103E-5\n4.38408\t1.6102E-5\n4.38792\t1.61E-5\n4.3908\t1.6099E-5\n4.39424\t1.6097E-5\n4.3952\t1.6096E-5\n4.39804\t1.6095E-5\n4.40088\t1.6093E-5\n4.40332\t1.6092E-5\n4.40532\t1.6091E-5\n4.40764\t1.609E-5\n4.40964\t1.6089E-5\n4.41152\t1.6088E-5\n4.41396\t1.6087E-5\n4.41696\t1.6085E-5\n4.41892\t1.6084E-5\n4.42188\t1.6082E-5\n4.42492\t1.6081E-5\n4.42732\t1.608E-5\n4.42924\t1.6079E-5\n4.43344\t1.6076E-5\n4.43432\t1.6076E-5\n4.43736\t1.6074E-5\n4.44\t1.6073E-5\n4.44144\t1.6072E-5\n4.44432\t1.6071E-5\n4.44652\t1.6069E-5\n4.44944\t1.6068E-5\n4.45148\t1.6067E-5\n4.45448\t1.6065E-5\n4.45764\t1.6064E-5\n4.45912\t1.6063E-5\n4.46232\t1.6061E-5\n4.46372\t1.606E-5\n4.46656\t1.6059E-5\n4.47024\t1.6057E-5\n4.47168\t1.6056E-5\n4.47464\t1.6055E-5\n4.47716\t1.6053E-5\n4.47908\t1.6052E-5\n4.48256\t1.605E-5\n4.4846\t1.6049E-5\n4.48652\t1.6048E-5\n4.48892\t1.6047E-5\n4.49188\t1.6045E-5\n4.49385\t1.6044E-5\n4.49672\t1.6043E-5\n4.49897\t1.6042E-5\n4.50156\t1.604E-5\n4.50384\t1.6039E-5\n4.50692\t1.6037E-5\n4.50885\t1.6036E-5\n4.512\t1.6035E-5\n4.51457\t1.6033E-5\n4.51648\t1.6032E-5\n4.51997\t1.603E-5\n4.52149\t1.6029E-5\n4.52441\t1.6028E-5\n4.52685\t1.6027E-5\n4.52985\t1.6025E-5\n4.53221\t1.6024E-5\n4.53417\t1.6023E-5\n4.53713\t1.6021E-5\n4.53917\t1.602E-5\n4.54209\t1.6018E-5\n4.54477\t1.6017E-5\n4.54673\t1.6016E-5\n4.54917\t1.6015E-5\n4.55337\t1.6012E-5\n4.55493\t1.6011E-5\n4.55925\t1.6009E-5\n4.56017\t1.6009E-5\n4.56297\t1.6007E-5\n4.56581\t1.6005E-5\n4.56829\t1.6004E-5\n4.57021\t1.6003E-5\n4.57453\t1.6001E-5\n4.57545\t1.6E-5\n4.57865\t1.5998E-5\n4.57989\t1.5998E-5\n4.58185\t1.5997E-5\n4.58405\t1.5996E-5\n4.58653\t1.5994E-5\n4.59009\t1.5992E-5\n4.59197\t1.5991E-5\n4.59481\t1.599E-5\n4.59733\t1.5988E-5\n4.59921\t1.5987E-5\n4.60269\t1.5985E-5\n4.60473\t1.5984E-5\n4.60661\t1.5983E-5\n4.60901\t1.5982E-5\n4.61213\t1.598E-5\n4.61437\t1.5979E-5\n4.61677\t1.5978E-5\n4.61989\t1.5976E-5\n4.62225\t1.5975E-5\n4.62417\t1.5973E-5\n4.62721\t1.5972E-5\n4.62966\t1.597E-5\n4.63157\t1.5969E-5\n4.63513\t1.5967E-5\n4.63665\t1.5967E-5\n4.63954\t1.5965E-5\n4.64205\t1.5964E-5\n4.64402\t1.5963E-5\n4.64702\t1.5961E-5\n4.64918\t1.596E-5\n4.65218\t1.5958E-5\n4.65414\t1.5957E-5\n4.65726\t1.5955E-5\n4.65926\t1.5954E-5\n4.66214\t1.5952E-5\n4.66418\t1.5951E-5\n4.6663\t1.595E-5\n4.6689\t1.5949E-5\n4.67162\t1.5947E-5\n4.6735\t1.5946E-5\n4.6755\t1.5945E-5\n4.67834\t1.5943E-5\n4.6793\t1.5943E-5\n4.68214\t1.5941E-5\n4.68462\t1.594E-5\n4.68666\t1.5939E-5\n4.69022\t1.5937E-5\n4.6921\t1.5936E-5\n4.69414\t1.5935E-5\n4.69658\t1.5933E-5\n4.69938\t1.5932E-5\n4.70298\t1.593E-5\n4.70486\t1.5929E-5\n4.70694\t1.5927E-5\n4.70946\t1.5926E-5\n4.7123\t1.5924E-5\n4.71418\t1.5923E-5\n4.71674\t1.5922E-5\n4.71966\t1.592E-5\n4.72202\t1.5919E-5\n4.72406\t1.5918E-5\n4.72694\t1.5916E-5\n4.72902\t1.5915E-5\n4.73198\t1.5913E-5\n4.73414\t1.5912E-5\n4.7367\t1.5911E-5\n4.7403\t1.5909E-5\n4.74178\t1.5908E-5\n4.74466\t1.5906E-5\n4.74746\t1.5904E-5\n4.74898\t1.5904E-5\n4.75218\t1.5902E-5\n4.75494\t1.59E-5\n4.75678\t1.5899E-5\n4.75918\t1.5898E-5\n4.76234\t1.5896E-5\n4.76474\t1.5895E-5\n4.76666\t1.5894E-5\n4.76934\t1.5892E-5\n4.77183\t1.5891E-5\n4.77475\t1.5889E-5\n4.77743\t1.5887E-5\n4.77927\t1.5886E-5\n4.78214\t1.5885E-5\n4.78467\t1.5883E-5\n4.78723\t1.5882E-5\n4.78959\t1.588E-5\n4.79167\t1.5879E-5\n4.79471\t1.5877E-5\n4.79711\t1.5876E-5\n4.79907\t1.5875E-5\n4.80255\t1.5873E-5\n4.80435\t1.5872E-5\n4.80707\t1.587E-5\n4.80951\t1.5869E-5\n4.81143\t1.5868E-5\n4.81495\t1.5866E-5\n4.81679\t1.5865E-5\n4.81967\t1.5863E-5\n4.82219\t1.5862E-5\n4.82411\t1.5861E-5\n4.82707\t1.5859E-5\n4.82903\t1.5858E-5\n4.83199\t1.5856E-5\n4.83399\t1.5855E-5\n4.83707\t1.5853E-5\n4.83943\t1.5852E-5\n4.84231\t1.585E-5\n4.84431\t1.5849E-5\n4.84639\t1.5848E-5\n4.84923\t1.5846E-5\n4.85179\t1.5844E-5\n4.85415\t1.5843E-5\n4.85663\t1.5842E-5\n4.85907\t1.584E-5\n4.86191\t1.5839E-5\n4.86427\t1.5837E-5\n4.86727\t1.5835E-5\n4.87027\t1.5834E-5\n4.87215\t1.5833E-5\n4.87411\t1.5831E-5\n4.87659\t1.583E-5\n4.87951\t1.5828E-5\n4.88151\t1.5827E-5\n4.88399\t1.5826E-5\n4.88679\t1.5824E-5\n4.88931\t1.5823E-5\n4.89223\t1.5821E-5\n4.89416\t1.582E-5\n4.89667\t1.5818E-5\n4.89967\t1.5816E-5\n4.90207\t1.5815E-5\n4.90404\t1.5814E-5\n4.90704\t1.5812E-5\n4.9094\t1.5811E-5\n4.91227\t1.5809E-5\n4.91476\t1.5808E-5\n4.91668\t1.5806E-5\n4.91972\t1.5805E-5\n4.92168\t1.5804E-5\n4.92456\t1.5802E-5\n4.9272\t1.58E-5\n4.92908\t1.5799E-5\n4.93152\t1.5798E-5\n4.934\t1.5796E-5\n4.93688\t1.5795E-5\n4.93928\t1.5793E-5\n4.94232\t1.5791E-5\n4.9442\t1.579E-5\n4.94656\t1.5789E-5\n4.94976\t1.5787E-5\n4.95172\t1.5786E-5\n4.95468\t1.5784E-5\n4.95668\t1.5783E-5\n4.95912\t1.5781E-5\n4.96204\t1.578E-5\n4.96452\t1.5778E-5\n4.96656\t1.5777E-5\n4.96904\t1.5775E-5\n4.97152\t1.5774E-5\n4.97452\t1.5772E-5\n4.97692\t1.5771E-5\n4.97864\t1.577E-5\n4.98156\t1.5768E-5\n4.984\t1.5766E-5\n4.98688\t1.5765E-5\n4.98936\t1.5763E-5\n4.99224\t1.5761E-5\n4.9942\t1.576E-5\n4.99728\t1.5758E-5\n4.9992\t1.5757E-5\n5.00232\t1.5755E-5\n5.00516\t1.5754E-5\n5.00892\t1.5751E-5\n5.01064\t1.575E-5\n5.01336\t1.5749E-5\n5.01472\t1.5748E-5\n5.01672\t1.5747E-5\n5.01968\t1.5745E-5\n5.02208\t1.5744E-5\n5.02404\t1.5742E-5\n5.02744\t1.574E-5\n5.02928\t1.5739E-5\n5.03248\t1.5737E-5\n5.03408\t1.5736E-5\n5.03693\t1.5735E-5\n5.04013\t1.5733E-5\n5.04197\t1.5731E-5\n5.04489\t1.573E-5\n5.04701\t1.5728E-5\n5.04897\t1.5727E-5\n5.05225\t1.5725E-5\n5.05433\t1.5724E-5\n5.05725\t1.5722E-5\n5.05961\t1.5721E-5\n5.06293\t1.5719E-5\n5.06505\t1.5717E-5\n5.06657\t1.5717E-5\n5.06977\t1.5715E-5\n5.07217\t1.5713E-5\n5.07405\t1.5712E-5\n5.07773\t1.571E-5\n5.07961\t1.5709E-5\n5.08153\t1.5707E-5\n5.08361\t1.5706E-5\n5.08653\t1.5704E-5\n5.08949\t1.5703E-5\n5.09249\t1.5701E-5\n5.09433\t1.57E-5\n5.09641\t1.5698E-5\n5.09945\t1.5696E-5\n5.10201\t1.5695E-5\n5.10401\t1.5694E-5\n5.10697\t1.5692E-5\n5.10937\t1.569E-5\n5.11225\t1.5689E-5\n5.11485\t1.5687E-5\n5.11677\t1.5686E-5\n5.11925\t1.5684E-5\n5.12177\t1.5683E-5\n5.12477\t1.5681E-5\n5.12713\t1.5679E-5\n5.12917\t1.5678E-5\n5.13209\t1.5676E-5\n5.13449\t1.5675E-5\n5.13609\t1.5674E-5\n5.13945\t1.5672E-5\n5.14189\t1.567E-5\n5.14549\t1.5668E-5\n5.14729\t1.5667E-5\n5.14917\t1.5666E-5\n5.15169\t1.5664E-5\n5.15469\t1.5662E-5\n5.15677\t1.5661E-5\n5.15933\t1.5659E-5\n5.16229\t1.5658E-5\n5.16421\t1.5656E-5\n5.16725\t1.5654E-5\n5.16914\t1.5653E-5\n5.17169\t1.5652E-5\n5.17478\t1.565E-5\n5.17709\t1.5648E-5\n5.17962\t1.5647E-5\n5.18157\t1.5646E-5\n5.18402\t1.5644E-5\n5.1869\t1.5642E-5\n5.1897\t1.564E-5\n5.19162\t1.5639E-5\n5.19446\t1.5637E-5\n5.19666\t1.5636E-5\n5.19962\t1.5634E-5\n5.20194\t1.5633E-5\n5.20414\t1.5631E-5\n5.20714\t1.563E-5\n5.2097\t1.5628E-5\n5.2119\t1.5627E-5\n5.21458\t1.5625E-5\n5.2165\t1.5624E-5\n5.22006\t1.5621E-5\n5.22194\t1.562E-5\n5.22482\t1.5618E-5\n5.22738\t1.5617E-5\n5.22926\t1.5616E-5\n5.2327\t1.5613E-5\n5.23478\t1.5612E-5\n5.23666\t1.5611E-5\n5.23906\t1.5609E-5\n5.24162\t1.5608E-5\n5.24514\t1.5606E-5\n5.24694\t1.5604E-5\n5.24958\t1.5603E-5\n5.25198\t1.5601E-5\n5.25446\t1.56E-5\n5.25746\t1.5598E-5\n5.25898\t1.5597E-5\n5.26174\t1.5595E-5\n5.26426\t1.5593E-5\n5.26726\t1.5592E-5\n5.26922\t1.559E-5\n5.27226\t1.5588E-5\n5.27418\t1.5587E-5\n5.27626\t1.5586E-5\n5.27922\t1.5584E-5\n5.2817\t1.5582E-5\n5.28414\t1.5581E-5\n5.28774\t1.5578E-5\n5.28962\t1.5577E-5\n5.2915\t1.5576E-5\n5.29454\t1.5574E-5\n5.2965\t1.5573E-5\n5.29978\t1.5571E-5\n5.30315\t1.5569E-5\n5.30611\t1.5567E-5\n5.30846\t1.5565E-5\n5.31095\t1.5564E-5\n5.31346\t1.5562E-5\n5.31678\t1.556E-5\n5.31783\t1.5559E-5\n5.31967\t1.5558E-5\n5.32207\t1.5556E-5\n5.32403\t1.5555E-5\n5.32751\t1.5553E-5\n5.32939\t1.5552E-5\n5.33195\t1.555E-5\n5.33411\t1.5549E-5\n5.33739\t1.5547E-5\n5.34015\t1.5545E-5\n5.34199\t1.5544E-5\n5.34395\t1.5542E-5\n5.34699\t1.554E-5\n5.34899\t1.5539E-5\n5.35239\t1.5537E-5\n5.35439\t1.5536E-5\n5.35727\t1.5534E-5\n5.35927\t1.5532E-5\n5.36191\t1.5531E-5\n5.36443\t1.5529E-5\n5.36735\t1.5527E-5\n5.36935\t1.5526E-5\n5.37183\t1.5524E-5\n5.37479\t1.5522E-5\n5.37747\t1.5521E-5\n5.37935\t1.5519E-5\n5.38215\t1.5518E-5\n5.38587\t1.5515E-5\n5.38779\t1.5514E-5\n5.39203\t1.5511E-5\n5.39275\t1.5511E-5\n5.39423\t1.551E-5\n5.39755\t1.5508E-5\n5.40035\t1.5506E-5\n5.40283\t1.5504E-5\n5.40567\t1.5502E-5\n5.40839\t1.55E-5\n5.40927\t1.55E-5\n5.41131\t1.5499E-5\n5.41387\t1.5497E-5\n5.41731\t1.5495E-5\n5.41919\t1.5493E-5\n5.42227\t1.5491E-5\n5.42467\t1.549E-5\n5.42659\t1.5489E-5\n5.43015\t1.5486E-5\n5.43199\t1.5485E-5\n5.43491\t1.5483E-5\n5.43679\t1.5482E-5\n5.43891\t1.548E-5\n5.44175\t1.5479E-5\n5.44395\t1.5477E-5\n5.44652\t1.5475E-5\n5.44896\t1.5474E-5\n5.45184\t1.5472E-5\n5.45536\t1.547E-5\n5.45683\t1.5469E-5\n5.45996\t1.5467E-5\n5.462\t1.5465E-5\n5.46484\t1.5463E-5\n5.46832\t1.5461E-5\n5.4692\t1.546E-5\n5.47196\t1.5459E-5\n5.47404\t1.5457E-5\n5.4766\t1.5456E-5\n5.47972\t1.5453E-5\n5.48164\t1.5452E-5\n5.48468\t1.545E-5\n5.48704\t1.5449E-5\n5.48912\t1.5447E-5\n5.49264\t1.5445E-5\n5.49416\t1.5444E-5\n5.49728\t1.5442E-5\n5.49976\t1.544E-5\n5.50168\t1.5439E-5\n5.50532\t1.5436E-5\n5.50724\t1.5435E-5\n5.50912\t1.5434E-5\n5.51188\t1.5432E-5\n5.51484\t1.543E-5\n5.51676\t1.5429E-5\n5.51936\t1.5427E-5\n5.52152\t1.5426E-5\n5.52412\t1.5424E-5\n5.52712\t1.5422E-5\n5.52912\t1.5421E-5\n5.53152\t1.5419E-5\n5.53444\t1.5417E-5\n5.53688\t1.5415E-5\n5.53976\t1.5413E-5\n5.54176\t1.5412E-5\n5.54432\t1.541E-5\n5.5468\t1.5409E-5\n5.54936\t1.5407E-5\n5.55228\t1.5405E-5\n5.55416\t1.5404E-5\n5.55668\t1.5402E-5\n5.55972\t1.54E-5\n5.56172\t1.5399E-5\n5.5648\t1.5397E-5\n5.56668\t1.5395E-5\n5.56908\t1.5394E-5\n5.57273\t1.5391E-5\n5.57605\t1.5389E-5\n5.578\t1.5388E-5\n5.58057\t1.5386E-5\n5.58293\t1.5384E-5\n5.58689\t1.5382E-5\n5.58784\t1.5381E-5\n5.59045\t1.5379E-5\n5.59401\t1.5377E-5\n5.59633\t1.5375E-5\n5.59813\t1.5374E-5\n5.60141\t1.5372E-5\n5.60309\t1.5371E-5\n5.60593\t1.5369E-5\n5.60829\t1.5367E-5\n5.61033\t1.5366E-5\n5.61325\t1.5364E-5\n5.61797\t1.536E-5\n5.61797\t1.536E-5\n5.62041\t1.5359E-5\n5.62477\t1.5356E-5\n5.62561\t1.5355E-5\n5.62853\t1.5353E-5\n5.63165\t1.5351E-5\n5.63353\t1.535E-5\n5.63545\t1.5349E-5\n5.63833\t1.5347E-5\n5.64085\t1.5345E-5\n5.64277\t1.5344E-5\n5.64705\t1.5341E-5\n5.64801\t1.534E-5\n5.65049\t1.5338E-5\n5.65301\t1.5337E-5\n5.65561\t1.5335E-5\n5.65905\t1.5332E-5\n5.66165\t1.5331E-5\n5.66361\t1.5329E-5\n5.66601\t1.5328E-5\n5.66797\t1.5326E-5\n5.67057\t1.5324E-5\n5.67297\t1.5323E-5\n5.67693\t1.532E-5\n5.67797\t1.5319E-5\n5.68037\t1.5318E-5\n5.68417\t1.5315E-5\n5.68589\t1.5314E-5\n5.68729\t1.5313E-5\n5.68917\t1.5312E-5\n5.69229\t1.5309E-5\n5.69469\t1.5308E-5\n5.69657\t1.5306E-5\n5.70017\t1.5304E-5\n5.70209\t1.5303E-5\n5.70397\t1.5301E-5\n5.70642\t1.53E-5\n5.70901\t1.5298E-5\n5.7127\t1.5295E-5\n5.71473\t1.5294E-5\n5.71666\t1.5293E-5\n5.71906\t1.5291E-5\n5.72198\t1.5289E-5\n5.72397\t1.5287E-5\n5.72637\t1.5286E-5\n5.72938\t1.5284E-5\n5.73194\t1.5282E-5\n5.73382\t1.5281E-5\n5.73638\t1.5279E-5\n5.73886\t1.5277E-5\n5.74138\t1.5275E-5\n5.7449\t1.5273E-5\n5.74674\t1.5272E-5\n5.75018\t1.5269E-5\n5.75222\t1.5268E-5\n5.7541\t1.5266E-5\n5.7565\t1.5265E-5\n5.76026\t1.5262E-5\n5.76366\t1.526E-5\n5.7669\t1.5257E-5\n5.76786\t1.5257E-5\n5.77126\t1.5254E-5\n5.77374\t1.5253E-5\n5.77594\t1.5251E-5\n5.77842\t1.5249E-5\n5.78038\t1.5248E-5\n5.78254\t1.5247E-5\n5.78458\t1.5245E-5\n5.78654\t1.5244E-5\n5.78958\t1.5242E-5\n5.79194\t1.524E-5\n5.79482\t1.5238E-5\n5.7969\t1.5236E-5\n5.7999\t1.5234E-5\n5.80214\t1.5233E-5\n5.80478\t1.5231E-5\n5.8067\t1.5229E-5\n5.80966\t1.5227E-5\n5.81134\t1.5226E-5\n5.81426\t1.5224E-5\n5.81722\t1.5222E-5\n5.81914\t1.5221E-5\n5.82162\t1.5219E-5\n5.82462\t1.5217E-5\n5.82654\t1.5215E-5\n5.82898\t1.5214E-5\n5.83182\t1.5212E-5\n5.83434\t1.521E-5\n5.83691\t1.5208E-5\n5.84002\t1.5206E-5\n5.84195\t1.5204E-5\n5.84454\t1.5203E-5\n5.84739\t1.5201E-5\n5.84934\t1.5199E-5\n5.85283\t1.5197E-5\n5.8547\t1.5195E-5\n5.85663\t1.5194E-5\n5.85915\t1.5192E-5\n5.86203\t1.519E-5\n5.86639\t1.5187E-5\n5.86827\t1.5186E-5\n5.87223\t1.5183E-5\n5.87359\t1.5182E-5\n5.87547\t1.5181E-5\n5.88003\t1.5177E-5\n5.88095\t1.5177E-5\n5.88283\t1.5175E-5\n5.88739\t1.5172E-5\n5.88843\t1.5171E-5\n5.88927\t1.5171E-5\n5.89223\t1.5169E-5\n5.89479\t1.5167E-5\n5.89667\t1.5165E-5\n5.90011\t1.5163E-5\n5.90207\t1.5162E-5\n5.90407\t1.516E-5\n5.90647\t1.5158E-5\n5.90947\t1.5156E-5\n5.91147\t1.5155E-5\n5.91439\t1.5153E-5\n5.91703\t1.5151E-5\n5.91951\t1.5149E-5\n5.92215\t1.5147E-5\n5.92271\t1.5147E-5\n5.92595\t1.5144E-5\n5.92787\t1.5143E-5\n5.93215\t1.514E-5\n5.93307\t1.5139E-5\n5.93615\t1.5137E-5\n5.93963\t1.5134E-5\n5.94055\t1.5134E-5\n5.94303\t1.5132E-5\n5.94587\t1.513E-5\n5.94835\t1.5128E-5\n5.95027\t1.5127E-5\n5.95315\t1.5125E-5\n5.95571\t1.5123E-5\n5.95875\t1.5121E-5\n5.96131\t1.5119E-5\n5.96351\t1.5117E-5\n5.96599\t1.5115E-5\n5.96799\t1.5114E-5\n5.97059\t1.5112E-5\n5.97304\t1.511E-5\n5.97664\t1.5108E-5\n5.97823\t1.5106E-5\n5.98063\t1.5105E-5\n5.98288\t1.5103E-5\n5.9854\t1.5101E-5\n5.98727\t1.51E-5\n5.98916\t1.5098E-5\n5.99164\t1.5097E-5\n5.9946\t1.5094E-5\n5.99648\t1.5093E-5\n6.00004\t1.509E-5\n6.00184\t1.5089E-5\n6.00424\t1.5087E-5\n6.00732\t1.5085E-5\n6.0092\t1.5084E-5\n6.0116\t1.5082E-5\n6.01416\t1.508E-5\n6.0172\t1.5078E-5\n6.01912\t1.5076E-5\n6.0234\t1.5073E-5\n6.02432\t1.5073E-5\n6.0272\t1.5071E-5\n6.0298\t1.5069E-5\n6.03164\t1.5067E-5\n6.03444\t1.5065E-5\n6.03704\t1.5063E-5\n6.039\t1.5062E-5\n6.04232\t1.5059E-5\n6.04436\t1.5058E-5\n6.04728\t1.5056E-5\n6.04968\t1.5054E-5\n6.05168\t1.5053E-5\n6.05516\t1.505E-5\n6.05696\t1.5049E-5\n6.06008\t1.5046E-5\n6.06148\t1.5045E-5\n6.06404\t1.5043E-5\n6.06596\t1.5042E-5\n6.068\t1.504E-5\n6.06992\t1.5039E-5\n6.07276\t1.5037E-5\n6.076\t1.5035E-5\n6.07792\t1.5033E-5\n6.08236\t1.503E-5\n6.08324\t1.5029E-5\n6.08608\t1.5027E-5\n6.08916\t1.5025E-5\n6.09112\t1.5023E-5\n6.09304\t1.5022E-5\n6.09584\t1.502E-5\n6.09848\t1.5018E-5\n6.10036\t1.5016E-5\n6.10356\t1.5014E-5\n6.10585\t1.5012E-5\n6.10788\t1.5011E-5\n6.10896\t1.501E-5\n6.11189\t1.5008E-5\n6.11536\t1.5005E-5\n6.11721\t1.5004E-5\n6.11929\t1.5002E-5\n6.12173\t1.5E-5\n6.1246\t1.4998E-5\n6.12625\t1.4997E-5\n6.12925\t1.4995E-5\n6.13213\t1.4993E-5\n6.13469\t1.4991E-5\n6.13661\t1.4989E-5\n6.13993\t1.4987E-5\n6.14205\t1.4985E-5\n6.14401\t1.4984E-5\n6.14653\t1.4982E-5\n6.14949\t1.498E-5\n6.15153\t1.4978E-5\n6.15493\t1.4976E-5\n6.15749\t1.4974E-5\n6.15989\t1.4972E-5\n6.16145\t1.4971E-5\n6.16401\t1.4969E-5\n6.16653\t1.4967E-5\n6.16941\t1.4965E-5\n6.17193\t1.4963E-5\n6.17397\t1.4961E-5\n6.17681\t1.4959E-5\n6.17933\t1.4957E-5\n6.18185\t1.4955E-5\n6.18429\t1.4953E-5\n6.18669\t1.4952E-5\n6.18921\t1.495E-5\n6.19165\t1.4948E-5\n6.19529\t1.4945E-5\n6.19829\t1.4943E-5\n6.20225\t1.494E-5\n6.20313\t1.4939E-5\n6.20549\t1.4937E-5\n6.20917\t1.4935E-5\n6.21161\t1.4933E-5\n6.21341\t1.4931E-5\n6.21665\t1.4929E-5\n6.21813\t1.4928E-5\n6.22101\t1.4926E-5\n6.22329\t1.4924E-5\n6.22541\t1.4922E-5\n6.22725\t1.4921E-5\n6.22913\t1.4919E-5\n6.23329\t1.4916E-5\n6.23593\t1.4914E-5\n6.23681\t1.4914E-5\n6.23933\t1.4912E-5\n6.2423\t1.4909E-5\n6.24473\t1.4908E-5\n6.24685\t1.4906E-5\n6.24982\t1.4904E-5\n6.25229\t1.4902E-5\n6.25434\t1.49E-5\n6.25738\t1.4898E-5\n6.25925\t1.4896E-5\n6.26226\t1.4894E-5\n6.26461\t1.4892E-5\n6.26718\t1.489E-5\n6.2697\t1.4888E-5\n6.27158\t1.4887E-5\n6.27406\t1.4885E-5\n6.27658\t1.4883E-5\n6.27954\t1.4881E-5\n6.28186\t1.4879E-5\n6.2849\t1.4877E-5\n6.28678\t1.4875E-5\n6.28882\t1.4874E-5\n6.29178\t1.4871E-5\n6.2943\t1.487E-5\n6.29718\t1.4867E-5\n6.29914\t1.4866E-5\n6.30166\t1.4864E-5\n6.30446\t1.4862E-5\n6.30706\t1.486E-5\n6.30866\t1.4858E-5\n6.31298\t1.4855E-5\n6.31502\t1.4854E-5\n6.31686\t1.4852E-5\n6.31926\t1.485E-5\n6.3227\t1.4848E-5\n6.32462\t1.4846E-5\n6.32702\t1.4844E-5\n6.33014\t1.4842E-5\n6.33278\t1.484E-5\n6.33426\t1.4839E-5\n6.33686\t1.4837E-5\n6.3393\t1.4835E-5\n6.34178\t1.4833E-5\n6.34426\t1.4831E-5\n6.34726\t1.4829E-5\n6.34914\t1.4827E-5\n6.35162\t1.4825E-5\n6.35454\t1.4823E-5\n6.35698\t1.4821E-5\n6.35938\t1.4819E-5\n6.36238\t1.4817E-5\n6.36482\t1.4815E-5\n6.36686\t1.4813E-5\n6.37038\t1.4811E-5\n6.37218\t1.4809E-5\n6.3747\t1.4807E-5\n6.37674\t1.4806E-5\n6.37959\t1.4803E-5\n6.38167\t1.4802E-5\n6.38471\t1.4799E-5\n6.38659\t1.4798E-5\n6.38867\t1.4796E-5\n6.39155\t1.4794E-5\n6.39403\t1.4792E-5\n6.39695\t1.479E-5\n6.39999\t1.4787E-5\n6.40183\t1.4786E-5\n6.40487\t1.4784E-5\n6.40683\t1.4782E-5\n6.40963\t1.478E-5\n6.41219\t1.4778E-5\n6.41415\t1.4776E-5\n6.41699\t1.4774E-5\n6.41947\t1.4772E-5\n6.42247\t1.477E-5\n6.42511\t1.4768E-5\n6.42715\t1.4766E-5\n6.42907\t1.4765E-5\n6.43239\t1.4762E-5\n6.43451\t1.476E-5\n6.43655\t1.4759E-5\n6.43987\t1.4756E-5\n6.44235\t1.4754E-5\n6.44479\t1.4752E-5\n6.44667\t1.4751E-5\n6.44975\t1.4748E-5\n6.45227\t1.4746E-5\n6.45427\t1.4745E-5\n6.45859\t1.4741E-5\n6.46051\t1.474E-5\n6.46443\t1.4737E-5\n6.46587\t1.4735E-5\n6.46787\t1.4734E-5\n6.46979\t1.4732E-5\n6.47231\t1.473E-5\n6.47423\t1.4729E-5\n6.47707\t1.4727E-5\n6.48075\t1.4724E-5\n6.48343\t1.4722E-5\n6.48431\t1.4721E-5\n6.48683\t1.4719E-5\n6.48983\t1.4716E-5\n6.49219\t1.4715E-5\n6.49427\t1.4713E-5\n6.49715\t1.4711E-5\n6.49947\t1.4709E-5\n6.50247\t1.4706E-5\n6.50451\t1.4705E-5\n6.50739\t1.4702E-5\n6.50899\t1.4701E-5\n6.51156\t1.4699E-5\n6.51439\t1.4697E-5\n6.51692\t1.4695E-5\n6.51988\t1.4692E-5\n6.52176\t1.4691E-5\n6.52427\t1.4689E-5\n6.52676\t1.4687E-5\n6.52911\t1.4685E-5\n6.53224\t1.4683E-5\n6.53412\t1.4681E-5\n6.53676\t1.4679E-5\n6.5398\t1.4677E-5\n6.54224\t1.4675E-5\n6.54416\t1.4673E-5\n6.54672\t1.4671E-5\n6.54944\t1.4669E-5\n6.55228\t1.4667E-5\n6.55444\t1.4665E-5\n6.55736\t1.4662E-5\n6.55976\t1.466E-5\n6.56176\t1.4659E-5\n6.56472\t1.4656E-5\n6.56716\t1.4655E-5\n6.56908\t1.4653E-5\n6.57176\t1.4651E-5\n6.57468\t1.4648E-5\n6.57664\t1.4647E-5\n6.57912\t1.4645E-5\n6.58208\t1.4642E-5\n6.58464\t1.464E-5\n6.5866\t1.4639E-5\n6.5894\t1.4637E-5\n6.59196\t1.4635E-5\n6.59432\t1.4633E-5\n6.59776\t1.463E-5\n6.59984\t1.4628E-5\n6.60172\t1.4627E-5\n6.60476\t1.4624E-5\n6.60704\t1.4622E-5\n6.609\t1.4621E-5\n6.6124\t1.4618E-5\n6.6148\t1.4616E-5\n6.61732\t1.4614E-5\n6.6192\t1.4612E-5\n6.62224\t1.461E-5\n6.6242\t1.4608E-5\n6.62716\t1.4606E-5\n6.62984\t1.4604E-5\n6.63172\t1.4602E-5\n6.63456\t1.46E-5\n6.63668\t1.4598E-5\n6.63968\t1.4596E-5\n6.64201\t1.4594E-5\n6.64596\t1.4591E-5\n6.64684\t1.459E-5\n6.64928\t1.4588E-5\n6.6524\t1.4585E-5\n6.65433\t1.4584E-5\n6.65673\t1.4582E-5\n6.66005\t1.4579E-5\n6.6634\t1.4576E-5\n6.66577\t1.4574E-5\n6.66845\t1.4572E-5\n6.66985\t1.4571E-5\n6.67177\t1.457E-5\n6.67437\t1.4567E-5\n6.67685\t1.4565E-5\n6.67973\t1.4563E-5\n6.68181\t1.4561E-5\n6.68481\t1.4559E-5\n6.68669\t1.4557E-5\n6.68885\t1.4556E-5\n6.69177\t1.4553E-5\n6.69417\t1.4551E-5\n6.69717\t1.4549E-5\n6.69973\t1.4547E-5\n6.70153\t1.4545E-5\n6.70505\t1.4542E-5\n6.70697\t1.4541E-5\n6.70869\t1.4539E-5\n6.71213\t1.4536E-5\n6.71409\t1.4535E-5\n6.71749\t1.4532E-5\n6.71953\t1.453E-5\n6.72153\t1.4529E-5\n6.72497\t1.4526E-5\n6.72701\t1.4524E-5\n6.73053\t1.4521E-5\n6.73161\t1.452E-5\n6.73513\t1.4517E-5\n6.73717\t1.4516E-5\n6.73909\t1.4514E-5\n6.74245\t1.4511E-5\n6.74489\t1.4509E-5\n6.74677\t1.4508E-5\n6.75037\t1.4505E-5\n6.75213\t1.4503E-5\n6.75425\t1.4502E-5\n6.75661\t1.45E-5\n6.75917\t1.4497E-5\n6.76225\t1.4495E-5\n6.76429\t1.4493E-5\n6.76693\t1.4491E-5\n6.76989\t1.4489E-5\n6.77185\t1.4487E-5\n6.77433\t1.4485E-5\n6.77722\t1.4482E-5\n6.77981\t1.448E-5\n6.78174\t1.4479E-5\n6.78421\t1.4477E-5\n6.78669\t1.4475E-5\n6.78965\t1.4472E-5\n6.79205\t1.447E-5\n6.79406\t1.4468E-5\n6.79634\t1.4466E-5\n6.7997\t1.4464E-5\n6.80178\t1.4462E-5\n6.80426\t1.446E-5\n6.80722\t1.4457E-5\n6.80918\t1.4456E-5\n6.8123\t1.4453E-5\n6.81418\t1.4452E-5\n6.81666\t1.4449E-5\n6.81958\t1.4447E-5\n6.82302\t1.4444E-5\n6.82454\t1.4443E-5\n6.82654\t1.4441E-5\n6.82982\t1.4438E-5\n6.8335\t1.4435E-5\n6.83582\t1.4433E-5\n6.83974\t1.443E-5\n6.84062\t1.4429E-5\n6.84302\t1.4427E-5\n6.84658\t1.4424E-5\n6.84838\t1.4423E-5\n6.8509\t1.4421E-5\n6.85322\t1.4419E-5\n6.85598\t1.4416E-5\n6.85738\t1.4415E-5\n6.85926\t1.4414E-5\n6.86238\t1.4411E-5\n6.86478\t1.4409E-5\n6.8667\t1.4407E-5\n6.87022\t1.4404E-5\n6.8721\t1.4403E-5\n6.87418\t1.4401E-5\n6.8767\t1.4399E-5\n6.87918\t1.4397E-5\n6.88258\t1.4394E-5\n6.88454\t1.4392E-5\n6.88654\t1.4391E-5\n6.88934\t1.4388E-5\n6.89246\t1.4386E-5\n6.89454\t1.4384E-5\n6.8969\t1.4382E-5\n6.89994\t1.4379E-5\n6.90234\t1.4377E-5\n6.90422\t1.4376E-5\n6.9073\t1.4373E-5\n6.9097\t1.4371E-5\n6.91162\t1.4369E-5\n6.91543\t1.4366E-5\n6.91847\t1.4363E-5\n6.91931\t1.4363E-5\n6.9219\t1.436E-5\n6.92439\t1.4358E-5\n6.92827\t1.4355E-5\n6.92887\t1.4355E-5\n6.93178\t1.4352E-5\n6.93475\t1.435E-5\n6.93655\t1.4348E-5\n6.93959\t1.4345E-5\n6.94247\t1.4343E-5\n6.94447\t1.4341E-5\n6.94659\t1.4339E-5\n6.94943\t1.4337E-5\n6.95195\t1.4335E-5\n6.95499\t1.4332E-5\n6.95703\t1.433E-5\n6.95951\t1.4328E-5\n6.96235\t1.4326E-5\n6.96471\t1.4324E-5\n6.96671\t1.4322E-5\n6.97031\t1.4319E-5\n6.97235\t1.4317E-5\n6.97435\t1.4316E-5\n6.97683\t1.4313E-5\n6.97975\t1.4311E-5\n6.98179\t1.4309E-5\n6.98423\t1.4307E-5\n6.98703\t1.4305E-5\n6.98963\t1.4302E-5\n6.99155\t1.4301E-5\n6.99435\t1.4298E-5\n6.99687\t1.4296E-5\n6.99983\t1.4294E-5\n7.00223\t1.4292E-5\n7.00427\t1.429E-5\n7.00719\t1.4287E-5\n7.00971\t1.4285E-5\n7.01163\t1.4284E-5\n7.01535\t1.428E-5\n7.01731\t1.4279E-5\n7.01931\t1.4277E-5\n7.02175\t1.4275E-5\n7.02423\t1.4273E-5\n7.02775\t1.427E-5\n7.02967\t1.4268E-5\n7.03127\t1.4267E-5\n7.03427\t1.4264E-5\n7.03727\t1.4261E-5\n7.03979\t1.4259E-5\n7.04179\t1.4257E-5\n7.04427\t1.4255E-5\n7.04719\t1.4253E-5\n7.04948\t1.4251E-5\n7.05235\t1.4248E-5\n7.05424\t1.4247E-5\n7.05771\t1.4244E-5\n7.0596\t1.4242E-5\n7.06248\t1.4239E-5\n7.065\t1.4237E-5\n7.06652\t1.4236E-5\n7.06992\t1.4233E-5\n7.07196\t1.4231E-5\n7.07392\t1.4229E-5\n7.07736\t1.4226E-5\n7.07944\t1.4225E-5\n7.08172\t1.4223E-5\n7.08376\t1.4221E-5\n7.08668\t1.4218E-5\n7.08916\t1.4216E-5\n7.0922\t1.4213E-5\n7.09416\t1.4212E-5\n7.09664\t1.421E-5\n7.09956\t1.4207E-5\n7.10208\t1.4205E-5\n7.10412\t1.4203E-5\n7.107\t1.4201E-5\n7.10948\t1.4198E-5\n7.11144\t1.4197E-5\n7.11476\t1.4194E-5\n7.1164\t1.4192E-5\n7.11932\t1.419E-5\n7.12172\t1.4188E-5\n7.12476\t1.4185E-5\n7.1272\t1.4183E-5\n7.12908\t1.4181E-5\n7.13228\t1.4178E-5\n7.13404\t1.4177E-5\n7.13684\t1.4174E-5\n7.14036\t1.4171E-5\n7.14224\t1.417E-5\n7.14416\t1.4168E-5\n7.1466\t1.4166E-5\n7.14968\t1.4163E-5\n7.15156\t1.4161E-5\n7.15508\t1.4158E-5\n7.15704\t1.4157E-5\n7.15908\t1.4155E-5\n7.16212\t1.4152E-5\n7.16404\t1.415E-5\n7.16752\t1.4147E-5\n7.16952\t1.4146E-5\n7.17196\t1.4143E-5\n7.17488\t1.4141E-5\n7.17693\t1.4139E-5\n7.17933\t1.4137E-5\n7.1822\t1.4134E-5\n7.18477\t1.4132E-5\n7.18664\t1.413E-5\n7.18953\t1.4128E-5\n7.19204\t1.4126E-5\n7.19401\t1.4124E-5\n7.19741\t1.4121E-5\n7.19941\t1.4119E-5\n7.20233\t1.4116E-5\n7.20473\t1.4114E-5\n7.20669\t1.4113E-5\n7.21021\t1.4109E-5\n7.21213\t1.4108E-5\n7.21369\t1.4106E-5\n7.21709\t1.4103E-5\n7.21985\t1.4101E-5\n7.22245\t1.4099E-5\n7.22433\t1.4097E-5\n7.22725\t1.4094E-5\n7.22985\t1.4092E-5\n7.23177\t1.409E-5\n7.23557\t1.4087E-5\n7.23765\t1.4085E-5\n7.23913\t1.4084E-5\n7.24153\t1.4081E-5\n7.24449\t1.4079E-5\n7.24657\t1.4077E-5\n7.24989\t1.4074E-5\n7.25185\t1.4072E-5\n7.25433\t1.407E-5\n7.25713\t1.4068E-5\n7.25997\t1.4065E-5\n7.26245\t1.4063E-5\n7.26433\t1.4061E-5\n7.26685\t1.4059E-5\n7.26973\t1.4056E-5\n7.27209\t1.4054E-5\n7.27481\t1.4052E-5\n7.27689\t1.405E-5\n7.27933\t1.4048E-5\n7.28253\t1.4045E-5\n7.28493\t1.4043E-5\n7.28681\t1.4041E-5\n7.28973\t1.4038E-5\n7.29177\t1.4036E-5\n7.29469\t1.4034E-5\n7.29729\t1.4031E-5\n7.29921\t1.403E-5\n7.30213\t1.4027E-5\n7.30461\t1.4025E-5\n7.30665\t1.4023E-5\n7.31001\t1.402E-5\n7.31197\t1.4018E-5\n7.31426\t1.4016E-5\n7.31666\t1.4014E-5\n7.31921\t1.4012E-5\n7.3227\t1.4008E-5\n7.32461\t1.4007E-5\n7.32658\t1.4005E-5\n7.32962\t1.4002E-5\n7.33153\t1.4001E-5\n7.33506\t1.3997E-5\n7.33689\t1.3996E-5\n7.33982\t1.3993E-5\n7.34246\t1.3991E-5\n7.34434\t1.3989E-5\n7.34778\t1.3986E-5\n7.34934\t1.3984E-5\n7.35226\t1.3982E-5\n7.35474\t1.3979E-5\n7.35678\t1.3978E-5\n7.36026\t1.3974E-5\n7.36186\t1.3973E-5\n7.36498\t1.397E-5\n7.36658\t1.3969E-5\n7.36926\t1.3966E-5\n7.37286\t1.3963E-5\n7.37434\t1.3962E-5\n7.37726\t1.3959E-5\n7.37982\t1.3957E-5\n7.38138\t1.3955E-5\n7.3847\t1.3952E-5\n7.38666\t1.395E-5\n7.38926\t1.3948E-5\n7.39166\t1.3946E-5\n7.39422\t1.3943E-5\n7.39666\t1.3941E-5\n7.39918\t1.3939E-5\n7.40278\t1.3936E-5\n7.40458\t1.3934E-5\n7.40702\t1.3932E-5\n7.4103\t1.3929E-5\n7.41326\t1.3926E-5\n7.41634\t1.3923E-5\n7.41858\t1.3921E-5\n7.4205\t1.3919E-5\n7.4233\t1.3917E-5\n7.42554\t1.3915E-5\n7.42742\t1.3913E-5\n7.42982\t1.3911E-5\n7.4319\t1.3909E-5\n7.43538\t1.3906E-5\n7.43726\t1.3904E-5\n7.4393\t1.3902E-5\n7.44166\t1.39E-5\n7.44474\t1.3897E-5\n7.44766\t1.3894E-5\n7.44947\t1.3893E-5\n7.45238\t1.389E-5\n7.45498\t1.3888E-5\n7.45686\t1.3886E-5\n7.46023\t1.3883E-5\n7.46183\t1.3881E-5\n7.46439\t1.3879E-5\n7.46674\t1.3877E-5\n7.46983\t1.3874E-5\n7.47223\t1.3872E-5\n7.47411\t1.387E-5\n7.47711\t1.3867E-5\n7.47967\t1.3865E-5\n7.48123\t1.3863E-5\n7.48475\t1.386E-5\n7.48635\t1.3859E-5\n7.48763\t1.3858E-5\n7.48967\t1.3856E-5\n7.49163\t1.3854E-5\n7.49415\t1.3852E-5\n7.49655\t1.3849E-5\n7.49955\t1.3847E-5\n7.50227\t1.3844E-5\n7.50415\t1.3842E-5\n7.50715\t1.3839E-5\n7.50951\t1.3837E-5\n7.51227\t1.3835E-5\n7.51491\t1.3832E-5\n7.51679\t1.3831E-5\n7.51971\t1.3828E-5\n7.52231\t1.3825E-5\n7.52423\t1.3824E-5\n7.52719\t1.3821E-5\n7.52915\t1.3819E-5\n7.53235\t1.3816E-5\n7.53475\t1.3814E-5\n7.53671\t1.3812E-5\n7.54015\t1.3809E-5\n7.54163\t1.3807E-5\n7.54463\t1.3805E-5\n7.54715\t1.3802E-5\n7.54911\t1.38E-5\n7.55271\t1.3797E-5\n7.55459\t1.3795E-5\n7.55679\t1.3793E-5\n7.56059\t1.379E-5\n7.56351\t1.3787E-5\n7.56691\t1.3784E-5\n7.56795\t1.3783E-5\n7.56987\t1.3781E-5\n7.57175\t1.3779E-5\n7.57427\t1.3777E-5\n7.57724\t1.3774E-5\n7.57964\t1.3772E-5\n7.58163\t1.377E-5\n7.58419\t1.3768E-5\n7.58719\t1.3765E-5\n7.58875\t1.3763E-5\n7.59179\t1.376E-5\n7.59492\t1.3757E-5\n7.59751\t1.3755E-5\n7.5994\t1.3753E-5\n7.60227\t1.3751E-5\n7.60488\t1.3748E-5\n7.60675\t1.3746E-5\n7.6102\t1.3743E-5\n7.61216\t1.3741E-5\n7.61416\t1.3739E-5\n7.6166\t1.3737E-5\n7.61952\t1.3734E-5\n7.62152\t1.3732E-5\n7.62484\t1.3729E-5\n7.62652\t1.3728E-5\n7.62956\t1.3725E-5\n7.63244\t1.3722E-5\n7.63508\t1.372E-5\n7.63676\t1.3718E-5\n7.63984\t1.3715E-5\n7.6424\t1.3713E-5\n7.64428\t1.3711E-5\n7.64772\t1.3708E-5\n7.64976\t1.3706E-5\n7.65164\t1.3704E-5\n7.65408\t1.3702E-5\n7.6566\t1.3699E-5\n7.66004\t1.3696E-5\n7.66192\t1.3694E-5\n7.665\t1.3691E-5\n7.6674\t1.3689E-5\n7.66928\t1.3687E-5\n7.67288\t1.3684E-5\n7.67432\t1.3682E-5\n7.67716\t1.368E-5\n7.67932\t1.3678E-5\n7.68236\t1.3675E-5\n7.68476\t1.3672E-5\n7.68672\t1.3671E-5\n7.68972\t1.3668E-5\n7.69216\t1.3665E-5\n7.69412\t1.3664E-5\n7.69756\t1.366E-5\n7.69908\t1.3659E-5\n7.70208\t1.3656E-5\n7.70448\t1.3654E-5\n7.70696\t1.3651E-5\n7.70948\t1.3649E-5\n7.71244\t1.3646E-5\n7.71432\t1.3644E-5\n7.71684\t1.3642E-5\n7.71988\t1.3639E-5\n7.72237\t1.3637E-5\n7.72436\t1.3635E-5\n7.72693\t1.3632E-5\n7.72936\t1.363E-5\n7.73244\t1.3627E-5\n7.7348\t1.3625E-5\n7.73673\t1.3623E-5\n7.74161\t1.3618E-5\n7.74305\t1.3617E-5\n7.74689\t1.3613E-5\n7.74841\t1.3612E-5\n7.75033\t1.361E-5\n7.75357\t1.3607E-5\n7.75517\t1.3605E-5\n7.75801\t1.3602E-5\n7.76181\t1.3599E-5\n7.76273\t1.3598E-5\n7.76553\t1.3595E-5\n7.76805\t1.3593E-5\n7.77113\t1.359E-5\n7.77301\t1.3588E-5\n7.77549\t1.3586E-5\n7.77809\t1.3583E-5\n7.78149\t1.358E-5\n7.78441\t1.3577E-5\n7.78533\t1.3576E-5\n7.78829\t1.3573E-5\n7.79209\t1.357E-5\n7.79305\t1.3569E-5\n7.79553\t1.3566E-5\n7.79833\t1.3564E-5\n7.80073\t1.3561E-5\n7.80313\t1.3559E-5\n7.80669\t1.3555E-5\n7.80865\t1.3554E-5\n7.81101\t1.3551E-5\n7.81449\t1.3548E-5\n7.81549\t1.3547E-5\n7.81801\t1.3545E-5\n7.81989\t1.3543E-5\n7.82193\t1.3541E-5\n7.82445\t1.3538E-5\n7.82733\t1.3535E-5\n7.82945\t1.3533E-5\n7.83237\t1.3531E-5\n7.83425\t1.3529E-5\n7.83673\t1.3526E-5\n7.83901\t1.3524E-5\n7.84109\t1.3522E-5\n7.84309\t1.352E-5\n7.84569\t1.3518E-5\n7.84813\t1.3515E-5\n7.85173\t1.3512E-5\n7.8537\t1.351E-5\n7.85606\t1.3508E-5\n7.85837\t1.3505E-5\n7.86086\t1.3503E-5\n7.86322\t1.3501E-5\n7.8671\t1.3497E-5\n7.86806\t1.3496E-5\n7.8705\t1.3493E-5\n7.87362\t1.349E-5\n7.8771\t1.3487E-5\n7.87798\t1.3486E-5\n7.88086\t1.3483E-5\n7.88394\t1.348E-5\n7.88586\t1.3478E-5\n7.88962\t1.3475E-5\n7.89066\t1.3474E-5\n7.89354\t1.3471E-5\n7.8955\t1.3469E-5\n7.89846\t1.3466E-5\n7.90046\t1.3464E-5\n7.90198\t1.3463E-5\n7.90446\t1.346E-5\n7.90738\t1.3457E-5\n7.90942\t1.3455E-5\n7.91254\t1.3452E-5\n7.91438\t1.3451E-5\n7.91678\t1.3448E-5\n7.91978\t1.3445E-5\n7.92182\t1.3443E-5\n7.9247\t1.344E-5\n7.92678\t1.3438E-5\n7.92926\t1.3436E-5\n7.93218\t1.3433E-5\n7.9347\t1.3431E-5\n7.93666\t1.3429E-5\n7.93954\t1.3426E-5\n7.94206\t1.3423E-5\n7.94502\t1.342E-5\n7.9475\t1.3418E-5\n7.94954\t1.3416E-5\n7.95246\t1.3413E-5\n7.95446\t1.3411E-5\n7.95706\t1.3409E-5\n7.95914\t1.3406E-5\n7.9617\t1.3404E-5\n7.96534\t1.34E-5\n7.96722\t1.3398E-5\n7.96934\t1.3396E-5\n7.97186\t1.3394E-5\n7.97494\t1.3391E-5\n7.97686\t1.3389E-5\n7.97942\t1.3386E-5\n7.98235\t1.3383E-5\n7.98475\t1.3381E-5\n7.98678\t1.3379E-5\n7.98934\t1.3377E-5\n7.99234\t1.3374E-5\n7.99431\t1.3372E-5\n7.99679\t1.3369E-5\n7.99975\t1.3366E-5\n8.00175\t1.3364E-5\n8.00423\t1.3362E-5\n8.00671\t1.3359E-5\n8.00915\t1.3357E-5\n8.01239\t1.3354E-5\n8.01463\t1.3351E-5\n8.01675\t1.3349E-5\n8.01931\t1.3347E-5\n8.02171\t1.3344E-5\n8.02411\t1.3342E-5\n8.02703\t1.3339E-5\n8.02943\t1.3337E-5\n8.03247\t1.3334E-5\n8.03491\t1.3331E-5\n8.03687\t1.3329E-5\n8.03995\t1.3326E-5\n8.04235\t1.3324E-5\n8.04423\t1.3322E-5\n8.04847\t1.3318E-5\n8.05047\t1.3316E-5\n8.05239\t1.3314E-5\n8.05587\t1.331E-5\n8.05739\t1.3309E-5\n8.05927\t1.3307E-5\n8.06355\t1.3303E-5\n8.06543\t1.3301E-5\n8.06943\t1.3297E-5\n8.07039\t1.3296E-5\n8.07287\t1.3293E-5\n8.07715\t1.3289E-5\n8.07811\t1.3288E-5\n8.08103\t1.3285E-5\n8.08443\t1.3282E-5\n8.08539\t1.3281E-5\n8.08851\t1.3278E-5\n8.08995\t1.3276E-5\n8.09195\t1.3274E-5\n8.09443\t1.3272E-5\n8.09687\t1.3269E-5\n8.09991\t1.3266E-5\n8.10235\t1.3264E-5\n8.10459\t1.3261E-5\n8.10735\t1.3259E-5\n8.10975\t1.3256E-5\n8.11167\t1.3254E-5\n8.11527\t1.3251E-5\n8.11723\t1.3249E-5\n8.11911\t1.3247E-5\n8.12268\t1.3243E-5\n8.12452\t1.3241E-5\n8.12759\t1.3238E-5\n8.1296\t1.3236E-5\n8.1316\t1.3234E-5\n8.13451\t1.3231E-5\n8.13684\t1.3229E-5\n8.14032\t1.3225E-5\n8.14224\t1.3223E-5\n8.1442\t1.3221E-5\n8.14672\t1.3219E-5\n8.14956\t1.3216E-5\n8.15284\t1.3213E-5\n8.15476\t1.3211E-5\n8.15664\t1.3209E-5\n8.15916\t1.3206E-5\n8.16216\t1.3203E-5\n8.16408\t1.3201E-5\n8.16744\t1.3198E-5\n8.16932\t1.3196E-5\n8.17172\t1.3194E-5\n8.1748\t1.319E-5\n8.17632\t1.3189E-5\n8.17932\t1.3186E-5\n8.18236\t1.3183E-5\n8.18476\t1.318E-5\n8.18664\t1.3178E-5\n8.19036\t1.3175E-5\n8.1916\t1.3173E-5\n8.19444\t1.317E-5\n8.19696\t1.3168E-5\n8.19996\t1.3165E-5\n8.2018\t1.3163E-5\n8.20428\t1.316E-5\n8.20732\t1.3157E-5\n8.20972\t1.3155E-5\n8.21164\t1.3153E-5\n8.21464\t1.315E-5\n8.21664\t1.3148E-5\n8.2192\t1.3145E-5\n8.2218\t1.3143E-5\n8.22472\t1.314E-5\n8.22668\t1.3138E-5\n8.22916\t1.3135E-5\n8.23204\t1.3132E-5\n8.23452\t1.313E-5\n8.23704\t1.3127E-5\n8.24048\t1.3123E-5\n8.2426\t1.3121E-5\n8.24468\t1.3119E-5\n8.24712\t1.3117E-5\n8.24912\t1.3115E-5\n8.25204\t1.3112E-5\n8.25444\t1.3109E-5\n8.25752\t1.3106E-5\n8.25992\t1.3104E-5\n8.26177\t1.3102E-5\n8.26485\t1.3098E-5\n8.26728\t1.3096E-5\n8.26921\t1.3094E-5\n8.27276\t1.309E-5\n8.27457\t1.3088E-5\n8.27681\t1.3086E-5\n8.27889\t1.3084E-5\n8.28113\t1.3082E-5\n8.28305\t1.308E-5\n8.28585\t1.3077E-5\n8.28829\t1.3074E-5\n8.29077\t1.3072E-5\n8.29281\t1.307E-5\n8.29601\t1.3066E-5\n8.29689\t1.3065E-5\n8.29925\t1.3063E-5\n8.30217\t1.306E-5\n8.30465\t1.3057E-5\n8.30661\t1.3055E-5\n8.30957\t1.3052E-5\n8.31173\t1.305E-5\n8.31417\t1.3048E-5\n8.31665\t1.3045E-5\n8.31953\t1.3042E-5\n8.32253\t1.3039E-5\n8.32461\t1.3037E-5\n8.32657\t1.3035E-5\n8.33005\t1.3031E-5\n8.33205\t1.3029E-5\n8.33405\t1.3027E-5\n8.33697\t1.3024E-5\n8.34001\t1.3021E-5\n8.34249\t1.3018E-5\n8.34441\t1.3016E-5\n8.34793\t1.3013E-5\n8.34969\t1.3011E-5\n8.35177\t1.3009E-5\n8.35429\t1.3006E-5\n8.35725\t1.3003E-5\n8.35977\t1.3E-5\n8.36173\t1.2998E-5\n8.36461\t1.2995E-5\n8.36665\t1.2993E-5\n8.36965\t1.299E-5\n8.37205\t1.2988E-5\n8.37489\t1.2985E-5\n8.37697\t1.2982E-5\n8.37945\t1.298E-5\n8.38241\t1.2977E-5\n8.38497\t1.2974E-5\n8.38746\t1.2971E-5\n8.38977\t1.2969E-5\n8.39237\t1.2966E-5\n8.3943\t1.2964E-5\n8.39773\t1.2961E-5\n8.39978\t1.2959E-5\n8.40169\t1.2957E-5\n8.40462\t1.2954E-5\n8.40769\t1.295E-5\n8.41005\t1.2948E-5\n8.41194\t1.2946E-5\n8.41502\t1.2943E-5\n8.41746\t1.294E-5\n8.41938\t1.2938E-5\n8.4229\t1.2934E-5\n8.42474\t1.2933E-5\n8.42666\t1.293E-5\n8.42918\t1.2928E-5\n8.43218\t1.2925E-5\n8.43422\t1.2923E-5\n8.43674\t1.292E-5\n8.43926\t1.2917E-5\n8.44166\t1.2915E-5\n8.4445\t1.2912E-5\n8.44798\t1.2908E-5\n8.44986\t1.2906E-5\n8.4519\t1.2904E-5\n8.45434\t1.2901E-5\n8.45722\t1.2898E-5\n8.4593\t1.2896E-5\n8.46182\t1.2894E-5\n8.4641\t1.2891E-5\n8.46774\t1.2887E-5\n8.46954\t1.2885E-5\n8.47202\t1.2883E-5\n8.4745\t1.288E-5\n8.47702\t1.2878E-5\n8.47906\t1.2875E-5\n8.48206\t1.2872E-5\n8.48414\t1.287E-5\n8.48662\t1.2867E-5\n8.48958\t1.2864E-5\n8.49166\t1.2862E-5\n8.49458\t1.2859E-5\n8.49658\t1.2857E-5\n8.4991\t1.2854E-5\n8.50186\t1.2851E-5\n8.50438\t1.2849E-5\n8.50734\t1.2845E-5\n8.50922\t1.2843E-5\n8.51174\t1.2841E-5\n8.51426\t1.2838E-5\n8.5167\t1.2836E-5\n8.51974\t1.2832E-5\n8.52194\t1.283E-5\n8.52454\t1.2827E-5\n8.52683\t1.2825E-5\n8.53026\t1.2821E-5\n8.53178\t1.282E-5\n8.53491\t1.2816E-5\n8.53739\t1.2814E-5\n8.53927\t1.2812E-5\n8.5429\t1.2808E-5\n8.54479\t1.2806E-5\n8.54667\t1.2804E-5\n8.54887\t1.2801E-5\n8.55195\t1.2798E-5\n8.55423\t1.2796E-5\n8.55671\t1.2793E-5\n8.56027\t1.2789E-5\n8.56267\t1.2787E-5\n8.56423\t1.2785E-5\n8.56723\t1.2782E-5\n8.56963\t1.2779E-5\n8.57163\t1.2777E-5\n8.57507\t1.2773E-5\n8.57695\t1.2771E-5\n8.58003\t1.2768E-5\n8.58243\t1.2766E-5\n8.58431\t1.2764E-5\n8.58743\t1.276E-5\n8.58935\t1.2758E-5\n8.59219\t1.2755E-5\n8.59547\t1.2752E-5\n8.59855\t1.2748E-5\n8.59943\t1.2747E-5\n8.60191\t1.2745E-5\n8.60483\t1.2742E-5\n8.60727\t1.2739E-5\n8.60923\t1.2737E-5\n8.61175\t1.2734E-5\n8.61415\t1.2732E-5\n8.61707\t1.2728E-5\n8.61923\t1.2726E-5\n8.62207\t1.2723E-5\n8.62571\t1.2719E-5\n8.62659\t1.2718E-5\n8.62939\t1.2715E-5\n8.63263\t1.2712E-5\n8.63447\t1.271E-5\n8.63779\t1.2706E-5\n8.63951\t1.2704E-5\n8.64247\t1.2701E-5\n8.64483\t1.2699E-5\n8.64687\t1.2696E-5\n8.65031\t1.2693E-5\n8.65219\t1.2691E-5\n8.65415\t1.2689E-5\n8.65663\t1.2686E-5\n8.65947\t1.2683E-5\n8.66304\t1.2679E-5\n8.66491\t1.2677E-5\n8.66675\t1.2675E-5\n8.66919\t1.2672E-5\n8.67211\t1.2669E-5\n8.67548\t1.2666E-5\n8.67752\t1.2663E-5\n8.68\t1.2661E-5\n8.68196\t1.2659E-5\n8.68508\t1.2655E-5\n8.68744\t1.2653E-5\n8.68928\t1.2651E-5\n8.69236\t1.2647E-5\n8.69468\t1.2645E-5\n8.6968\t1.2642E-5\n8.69992\t1.2639E-5\n8.70184\t1.2637E-5\n8.70484\t1.2634E-5\n8.70684\t1.2632E-5\n8.70984\t1.2628E-5\n8.71224\t1.2626E-5\n8.7142\t1.2624E-5\n8.71732\t1.262E-5\n8.71924\t1.2618E-5\n8.72236\t1.2615E-5\n8.7248\t1.2612E-5\n8.72672\t1.261E-5\n8.73032\t1.2606E-5\n8.7324\t1.2604E-5\n8.73428\t1.2602E-5\n8.73632\t1.26E-5\n8.73932\t1.2596E-5\n8.74268\t1.2593E-5\n8.7446\t1.2591E-5\n8.7472\t1.2588E-5\n8.74916\t1.2586E-5\n8.75216\t1.2582E-5\n8.7546\t1.258E-5\n8.75712\t1.2577E-5\n8.75912\t1.2575E-5\n8.7616\t1.2572E-5\n8.76448\t1.2569E-5\n8.76696\t1.2566E-5\n8.76988\t1.2563E-5\n8.7718\t1.2561E-5\n8.77424\t1.2558E-5\n8.77728\t1.2555E-5\n8.77972\t1.2552E-5\n8.78168\t1.255E-5\n8.78408\t1.2547E-5\n8.78745\t1.2544E-5\n8.7894\t1.2542E-5\n8.7924\t1.2538E-5\n8.79433\t1.2536E-5\n8.79724\t1.2533E-5\n8.79932\t1.2531E-5\n8.80185\t1.2528E-5\n8.80429\t1.2525E-5\n8.8074\t1.2522E-5\n8.8098\t1.2519E-5\n8.81185\t1.2517E-5\n8.81481\t1.2514E-5\n8.81721\t1.2511E-5\n8.81921\t1.2509E-5\n8.82265\t1.2505E-5\n8.82417\t1.2503E-5\n8.82893\t1.2498E-5\n8.83073\t1.2496E-5\n8.83405\t1.2492E-5\n8.83537\t1.2491E-5\n8.83849\t1.2488E-5\n8.84005\t1.2486E-5\n8.84213\t1.2484E-5\n8.84413\t1.2481E-5\n8.84741\t1.2478E-5\n8.84945\t1.2475E-5\n8.85233\t1.2472E-5\n8.85481\t1.247E-5\n8.85677\t1.2467E-5\n8.86049\t1.2463E-5\n8.86237\t1.2461E-5\n8.86429\t1.2459E-5\n8.86681\t1.2456E-5\n8.86969\t1.2453E-5\n8.87137\t1.2451E-5\n8.87477\t1.2447E-5\n8.87669\t1.2445E-5\n8.87933\t1.2442E-5\n8.88241\t1.2439E-5\n8.88485\t1.2436E-5\n8.88697\t1.2434E-5\n8.88989\t1.2431E-5\n8.89189\t1.2429E-5\n8.89489\t1.2425E-5\n8.89741\t1.2422E-5\n8.89933\t1.242E-5\n8.90237\t1.2417E-5\n8.90477\t1.2414E-5\n8.90665\t1.2412E-5\n8.91021\t1.2408E-5\n8.91229\t1.2406E-5\n8.91421\t1.2404E-5\n8.91741\t1.24E-5\n8.91929\t1.2398E-5\n8.92273\t1.2394E-5\n8.92489\t1.2392E-5\n8.92714\t1.2389E-5\n8.92945\t1.2387E-5\n8.93265\t1.2383E-5\n8.93417\t1.2382E-5\n8.93742\t1.2378E-5\n8.93946\t1.2376E-5\n8.94162\t1.2373E-5\n8.94441\t1.237E-5\n8.94806\t1.2366E-5\n8.94994\t1.2364E-5\n8.95182\t1.2362E-5\n8.95442\t1.2359E-5\n8.95698\t1.2356E-5\n8.96038\t1.2352E-5\n8.96246\t1.235E-5\n8.96438\t1.2348E-5\n8.9669\t1.2345E-5\n8.96994\t1.2342E-5\n8.97242\t1.2339E-5\n8.9743\t1.2337E-5\n8.97734\t1.2333E-5\n8.97978\t1.2331E-5\n8.98166\t1.2328E-5\n8.9859\t1.2324E-5\n8.9887\t1.2321E-5\n8.99238\t1.2316E-5\n8.99302\t1.2316E-5\n8.9949\t1.2314E-5\n8.9969\t1.2311E-5\n8.99946\t1.2308E-5\n9.00198\t1.2306E-5\n9.00438\t1.2303E-5\n9.0081\t1.2299E-5\n9.01082\t1.2296E-5\n9.0123\t1.2294E-5\n9.01426\t1.2292E-5\n9.01678\t1.2289E-5\n9.01926\t1.2286E-5\n9.0229\t1.2282E-5\n9.02478\t1.228E-5\n9.0267\t1.2278E-5\n9.02886\t1.2275E-5\n9.03182\t1.2272E-5\n9.03526\t1.2268E-5\n9.03686\t1.2266E-5\n9.03978\t1.2263E-5\n9.04222\t1.226E-5\n9.04414\t1.2258E-5\n9.04762\t1.2254E-5\n9.04914\t1.2252E-5\n9.05214\t1.2249E-5\n9.05486\t1.2246E-5\n9.05674\t1.2244E-5\n9.05994\t1.224E-5\n9.06186\t1.2238E-5\n9.06474\t1.2235E-5\n9.06727\t1.2232E-5\n9.06923\t1.223E-5\n9.07255\t1.2226E-5\n9.0745\t1.2224E-5\n9.07743\t1.222E-5\n9.07983\t1.2218E-5\n9.08191\t1.2215E-5\n9.08499\t1.2212E-5\n9.08691\t1.221E-5\n9.08999\t1.2206E-5\n9.09239\t1.2203E-5\n9.09427\t1.2201E-5\n9.09783\t1.2197E-5\n9.09975\t1.2195E-5\n9.10167\t1.2193E-5\n9.10527\t1.2189E-5\n9.10707\t1.2187E-5\n9.11039\t1.2183E-5\n9.11243\t1.2181E-5\n9.11399\t1.2179E-5\n9.11663\t1.2176E-5\n9.11959\t1.2173E-5\n9.12163\t1.217E-5\n9.12499\t1.2166E-5\n9.12699\t1.2164E-5\n9.12943\t1.2161E-5\n9.13231\t1.2158E-5\n9.13435\t1.2156E-5\n9.13683\t1.2153E-5\n9.13979\t1.215E-5\n9.14235\t1.2147E-5\n9.14423\t1.2144E-5\n9.14707\t1.2141E-5\n9.14967\t1.2138E-5\n9.15167\t1.2136E-5\n9.15539\t1.2132E-5\n9.15751\t1.2129E-5\n9.15947\t1.2127E-5\n9.16187\t1.2124E-5\n9.16495\t1.2121E-5\n9.16647\t1.2119E-5\n9.16983\t1.2115E-5\n9.17215\t1.2112E-5\n9.17427\t1.211E-5\n9.17727\t1.2107E-5\n9.17999\t1.2104E-5\n9.18187\t1.2101E-5\n9.18435\t1.2099E-5\n9.18683\t1.2096E-5\n9.18984\t1.2092E-5\n9.19247\t1.2089E-5\n9.19447\t1.2087E-5\n9.19739\t1.2084E-5\n9.1998\t1.2081E-5\n9.20188\t1.2078E-5\n9.20527\t1.2074E-5\n9.20711\t1.2072E-5\n9.2102\t1.2069E-5\n9.21127\t1.2068E-5\n9.21508\t1.2063E-5\n9.21772\t1.206E-5\n9.21956\t1.2058E-5\n9.22208\t1.2055E-5\n9.22476\t1.2052E-5\n9.22672\t1.205E-5\n9.22912\t1.2047E-5\n9.23168\t1.2044E-5\n9.2348\t1.204E-5\n9.23664\t1.2038E-5\n9.23968\t1.2035E-5\n9.24208\t1.2032E-5\n9.24496\t1.2029E-5\n9.24768\t1.2026E-5\n9.24952\t1.2023E-5\n9.25244\t1.202E-5\n9.25496\t1.2017E-5\n9.25684\t1.2015E-5\n9.26028\t1.2011E-5\n9.26216\t1.2009E-5\n9.26504\t1.2005E-5\n9.2674\t1.2003E-5\n9.2694\t1.2E-5\n9.2728\t1.1996E-5\n9.27472\t1.1994E-5\n9.27668\t1.1992E-5\n9.27916\t1.1989E-5\n9.28168\t1.1986E-5\n9.28524\t1.1982E-5\n9.28712\t1.198E-5\n9.2896\t1.1977E-5\n9.29212\t1.1974E-5\n9.29416\t1.1972E-5\n9.29704\t1.1968E-5\n9.30016\t1.1965E-5\n9.30204\t1.1963E-5\n9.30444\t1.196E-5\n9.30752\t1.1956E-5\n9.30988\t1.1953E-5\n9.31176\t1.1951E-5\n9.31472\t1.1948E-5\n9.3172\t1.1945E-5\n9.3188\t1.1943E-5\n9.3224\t1.1939E-5\n9.32432\t1.1937E-5\n9.3272\t1.1933E-5\n9.32961\t1.193E-5\n9.33216\t1.1927E-5\n9.33465\t1.1925E-5\n9.33668\t1.1922E-5\n9.33964\t1.1919E-5\n9.34204\t1.1916E-5\n9.34461\t1.1913E-5\n9.34701\t1.191E-5\n9.34949\t1.1907E-5\n9.35273\t1.1903E-5\n9.35453\t1.1901E-5\n9.35701\t1.1898E-5\n9.35953\t1.1895E-5\n9.36245\t1.1892E-5\n9.36489\t1.1889E-5\n9.36693\t1.1887E-5\n9.36945\t1.1884E-5\n9.37185\t1.1881E-5\n9.37505\t1.1877E-5\n9.37749\t1.1874E-5\n9.37937\t1.1872E-5\n9.38245\t1.1869E-5\n9.38485\t1.1866E-5\n9.38673\t1.1864E-5\n9.39025\t1.1859E-5\n9.39213\t1.1857E-5\n9.39493\t1.1854E-5\n9.39753\t1.1851E-5\n9.39937\t1.1849E-5\n9.40241\t1.1845E-5\n9.40453\t1.1843E-5\n9.40749\t1.1839E-5\n9.40989\t1.1836E-5\n9.41181\t1.1834E-5\n9.41525\t1.183E-5\n9.41673\t1.1828E-5\n9.41929\t1.1825E-5\n9.42189\t1.1822E-5\n9.42477\t1.1819E-5\n9.42725\t1.1816E-5\n9.42945\t1.1813E-5\n9.43233\t1.181E-5\n9.43489\t1.1807E-5\n9.43737\t1.1804E-5\n9.43989\t1.1801E-5\n9.44193\t1.1799E-5\n9.44485\t1.1795E-5\n9.44729\t1.1792E-5\n9.44929\t1.179E-5\n9.45193\t1.1787E-5\n9.45481\t1.1783E-5\n9.45685\t1.1781E-5\n9.45897\t1.1778E-5\n9.46182\t1.1775E-5\n9.46454\t1.1772E-5\n9.4675\t1.1768E-5\n9.46941\t1.1766E-5\n9.47198\t1.1763E-5\n9.47489\t1.176E-5\n9.4769\t1.1757E-5\n9.47993\t1.1754E-5\n9.4819\t1.1751E-5\n9.48394\t1.1749E-5\n9.48694\t1.1745E-5\n9.48938\t1.1742E-5\n9.4923\t1.1739E-5\n9.4943\t1.1737E-5\n9.49698\t1.1733E-5\n9.49942\t1.173E-5\n9.50382\t1.1725E-5\n9.5061\t1.1723E-5\n9.50842\t1.172E-5\n9.51042\t1.1717E-5\n9.51326\t1.1714E-5\n9.51722\t1.1709E-5\n9.51818\t1.1708E-5\n9.52114\t1.1705E-5\n9.52454\t1.1701E-5\n9.5259\t1.1699E-5\n9.52818\t1.1696E-5\n9.5327\t1.1691E-5\n9.53362\t1.169E-5\n9.53546\t1.1688E-5\n9.53946\t1.1683E-5\n9.54042\t1.1682E-5\n9.54346\t1.1678E-5\n9.5465\t1.1674E-5\n9.5487\t1.1672E-5\n9.55054\t1.167E-5\n9.5533\t1.1666E-5\n9.55558\t1.1664E-5\n9.55746\t1.1661E-5\n9.55946\t1.1659E-5\n9.56254\t1.1655E-5\n9.5649\t1.1652E-5\n9.56678\t1.165E-5\n9.5699\t1.1646E-5\n9.5723\t1.1643E-5\n9.57422\t1.1641E-5\n9.57782\t1.1637E-5\n9.57926\t1.1635E-5\n9.5821\t1.1632E-5\n9.58542\t1.1628E-5\n9.58762\t1.1625E-5\n9.58998\t1.1622E-5\n9.59202\t1.162E-5\n9.59506\t1.1616E-5\n9.5975\t1.1613E-5\n9.5995\t1.1611E-5\n9.60307\t1.1607E-5\n9.60502\t1.1604E-5\n9.6071\t1.1602E-5\n9.60974\t1.1599E-5\n9.6113\t1.1597E-5\n9.61423\t1.1593E-5\n9.61671\t1.159E-5\n9.61975\t1.1586E-5\n9.62227\t1.1583E-5\n9.62423\t1.1581E-5\n9.62715\t1.1578E-5\n9.62971\t1.1574E-5\n9.63167\t1.1572E-5\n9.63507\t1.1568E-5\n9.63707\t1.1566E-5\n9.64003\t1.1562E-5\n9.64243\t1.1559E-5\n9.64443\t1.1557E-5\n9.64791\t1.1553E-5\n9.64979\t1.155E-5\n9.65175\t1.1548E-5\n9.65423\t1.1545E-5\n9.65675\t1.1542E-5\n9.65991\t1.1538E-5\n9.66183\t1.1536E-5\n9.66479\t1.1532E-5\n9.66743\t1.1529E-5\n9.66931\t1.1527E-5\n9.67271\t1.1523E-5\n9.67471\t1.152E-5\n9.67667\t1.1518E-5\n9.67999\t1.1514E-5\n9.68199\t1.1511E-5\n9.68559\t1.1507E-5\n9.68755\t1.1505E-5\n9.68951\t1.1502E-5\n9.69207\t1.1499E-5\n9.69451\t1.1496E-5\n9.69819\t1.1492E-5\n9.70003\t1.1489E-5\n9.70199\t1.1487E-5\n9.70455\t1.1484E-5\n9.70755\t1.148E-5\n9.70943\t1.1478E-5\n9.71263\t1.1474E-5\n9.71447\t1.1472E-5\n9.71683\t1.1469E-5\n9.71959\t1.1466E-5\n9.72175\t1.1463E-5\n9.72419\t1.146E-5\n9.72707\t1.1456E-5\n9.72923\t1.1454E-5\n9.73211\t1.145E-5\n9.73447\t1.1447E-5\n9.73687\t1.1445E-5\n9.7398\t1.1441E-5\n9.7424\t1.1438E-5\n9.74428\t1.1435E-5\n9.74711\t1.1432E-5\n9.75056\t1.1428E-5\n9.75244\t1.1426E-5\n9.75436\t1.1423E-5\n9.75692\t1.142E-5\n9.75992\t1.1416E-5\n9.76228\t1.1413E-5\n9.76424\t1.1411E-5\n9.7672\t1.1407E-5\n9.7692\t1.1405E-5\n9.77212\t1.1401E-5\n9.77456\t1.1398E-5\n9.77744\t1.1395E-5\n9.77944\t1.1392E-5\n9.78156\t1.139E-5\n9.78488\t1.1386E-5\n9.78664\t1.1384E-5\n9.7896\t1.138E-5\n9.792\t1.1377E-5\n9.79508\t1.1373E-5\n9.79696\t1.1371E-5\n9.7994\t1.1368E-5\n9.80252\t1.1364E-5\n9.80488\t1.1361E-5\n9.8068\t1.1359E-5\n9.81056\t1.1354E-5\n9.81296\t1.1351E-5\n9.81648\t1.1347E-5\n9.81876\t1.1344E-5\n9.82068\t1.1342E-5\n9.82316\t1.1339E-5\n9.82628\t1.1335E-5\n9.8282\t1.1333E-5\n9.83212\t1.1328E-5\n9.83308\t1.1327E-5\n9.83604\t1.1323E-5\n9.83952\t1.1319E-5\n9.84056\t1.1317E-5\n9.84356\t1.1314E-5\n9.84556\t1.1311E-5\n9.84756\t1.1309E-5\n9.84944\t1.1306E-5\n9.85188\t1.1303E-5\n9.85444\t1.13E-5\n9.85708\t1.1297E-5\n9.85996\t1.1293E-5\n9.86204\t1.1291E-5\n9.86453\t1.1288E-5\n9.86736\t1.1284E-5\n9.86996\t1.1281E-5\n9.87184\t1.1279E-5\n9.8748\t1.1275E-5\n9.87692\t1.1272E-5\n9.87932\t1.1269E-5\n9.88277\t1.1265E-5\n9.88469\t1.1263E-5\n9.88725\t1.126E-5\n9.88961\t1.1257E-5\n9.89277\t1.1253E-5\n9.89533\t1.125E-5\n9.89717\t1.1247E-5\n9.90029\t1.1243E-5\n9.90169\t1.1242E-5\n9.90453\t1.1238E-5\n9.90809\t1.1234E-5\n9.90997\t1.1231E-5\n9.91185\t1.1229E-5\n9.91433\t1.1226E-5\n9.91733\t1.1222E-5\n9.91921\t1.122E-5\n9.92173\t1.1217E-5\n9.92457\t1.1213E-5\n9.92701\t1.121E-5\n9.93021\t1.1206E-5\n9.93205\t1.1204E-5\n9.93445\t1.1201E-5\n9.93705\t1.1198E-5\n9.93953\t1.1195E-5\n9.94237\t1.1191E-5\n9.94521\t1.1188E-5\n9.94705\t1.1185E-5\n9.95001\t1.1182E-5\n9.95257\t1.1178E-5\n9.95445\t1.1176E-5\n9.95785\t1.1172E-5\n9.96001\t1.1169E-5\n9.96189\t1.1167E-5\n9.96397\t1.1164E-5\n9.96697\t1.116E-5\n9.97045\t1.1156E-5\n9.97233\t1.1154E-5\n9.97441\t1.1151E-5\n9.97685\t1.1148E-5\n9.97981\t1.1144E-5\n9.98177\t1.1142E-5\n9.98445\t1.1139E-5\n9.98669\t1.1136E-5\n9.99017\t1.1131E-5\n9.99201\t1.1129E-5\n9.99489\t1.1125E-5\n9.99749\t1.1122E-5\n9.99937\t1.112E-5\n10.00237\t1.1116E-5\n10.00437\t1.1114E-5\n10.00741\t1.111E-5\n10.00985\t1.1107E-5\n10.01185\t1.1104E-5\n10.01494\t1.11E-5\n10.01646\t1.1098E-5\n10.01902\t1.1095E-5\n10.02242\t1.1091E-5\n10.02434\t1.1089E-5\n10.02682\t1.1085E-5\n10.02986\t1.1082E-5\n10.03174\t1.1079E-5\n10.03434\t1.1076E-5\n10.03742\t1.1072E-5\n10.03986\t1.1069E-5\n10.0419\t1.1066E-5\n10.04442\t1.1063E-5\n10.04654\t1.1061E-5\n10.0491\t1.1057E-5\n10.05254\t1.1053E-5\n10.05442\t1.1051E-5\n10.05798\t1.1046E-5\n10.0599\t1.1044E-5\n10.06178\t1.1041E-5\n10.06438\t1.1038E-5\n10.06742\t1.1034E-5\n10.06894\t1.1032E-5\n10.07198\t1.1028E-5\n10.0749\t1.1025E-5\n10.07734\t1.1022E-5\n10.0793\t1.1019E-5\n10.08278\t1.1015E-5\n10.08458\t1.1013E-5\n10.0877\t1.1009E-5\n10.08962\t1.1006E-5\n10.0925\t1.1003E-5\n10.09462\t1.1E-5\n10.09714\t1.0997E-5\n10.10062\t1.0992E-5\n10.1027\t1.099E-5\n10.10458\t1.0987E-5\n10.10698\t1.0984E-5\n10.11006\t1.098E-5\n10.11198\t1.0978E-5\n10.11442\t1.0975E-5\n10.11682\t1.0972E-5\n10.11934\t1.0968E-5\n10.12186\t1.0965E-5\n10.12546\t1.0961E-5\n10.12726\t1.0958E-5\n10.12982\t1.0955E-5\n10.13242\t1.0952E-5\n10.1343\t1.0949E-5\n10.13778\t1.0945E-5\n10.13938\t1.0943E-5\n10.14191\t1.094E-5\n10.14431\t1.0937E-5\n10.14738\t1.0933E-5\n10.14982\t1.093E-5\n10.15171\t1.0927E-5\n10.15467\t1.0924E-5\n10.15675\t1.0921E-5\n10.15963\t1.0917E-5\n10.16175\t1.0915E-5\n10.16471\t1.0911E-5\n10.16803\t1.0906E-5\n10.17007\t1.0904E-5\n10.17259\t1.0901E-5\n10.17499\t1.0898E-5\n10.17703\t1.0895E-5\n10.18043\t1.0891E-5\n10.18231\t1.0888E-5\n10.18447\t1.0886E-5\n10.18691\t1.0882E-5\n10.18979\t1.0879E-5\n10.19175\t1.0876E-5\n10.19427\t1.0873E-5\n10.19711\t1.0869E-5\n10.19959\t1.0866E-5\n10.20211\t1.0863E-5\n10.20511\t1.0859E-5\n10.20711\t1.0857E-5\n10.20979\t1.0853E-5\n10.21215\t1.085E-5\n10.21587\t1.0845E-5\n10.21827\t1.0842E-5\n10.22187\t1.0838E-5\n10.22379\t1.0835E-5\n10.22619\t1.0832E-5\n10.22815\t1.083E-5\n10.23119\t1.0826E-5\n10.23359\t1.0823E-5\n10.23547\t1.082E-5\n10.23811\t1.0817E-5\n10.24051\t1.0814E-5\n10.24447\t1.0809E-5\n10.24551\t1.0807E-5\n10.24791\t1.0804E-5\n10.25119\t1.08E-5\n10.25427\t1.0796E-5\n10.25615\t1.0794E-5\n10.25847\t1.0791E-5\n10.26147\t1.0787E-5\n10.26359\t1.0784E-5\n10.26411\t1.0783E-5\n10.26784\t1.0778E-5\n10.26971\t1.0776E-5\n10.27264\t1.0772E-5\n10.27523\t1.0769E-5\n10.27708\t1.0767E-5\n10.28016\t1.0763E-5\n10.28212\t1.076E-5\n10.28475\t1.0757E-5\n10.28712\t1.0754E-5\n10.2896\t1.075E-5\n10.29204\t1.0747E-5\n10.29496\t1.0743E-5\n10.297\t1.0741E-5\n10.29944\t1.0738E-5\n10.3024\t1.0734E-5\n10.305\t1.073E-5\n10.30688\t1.0728E-5\n10.3094\t1.0725E-5\n10.31152\t1.0722E-5\n10.31444\t1.0718E-5\n10.31684\t1.0715E-5\n10.31976\t1.0711E-5\n10.32284\t1.0707E-5\n10.32428\t1.0706E-5\n10.3274\t1.0701E-5\n10.32976\t1.0698E-5\n10.33192\t1.0696E-5\n10.33512\t1.0691E-5\n10.337\t1.0689E-5\n10.33996\t1.0685E-5\n10.34204\t1.0682E-5\n10.34504\t1.0679E-5\n10.34744\t1.0675E-5\n10.34944\t1.0673E-5\n10.3524\t1.0669E-5\n10.3548\t1.0666E-5\n10.35676\t1.0663E-5\n10.36028\t1.0659E-5\n10.36212\t1.0656E-5\n10.36516\t1.0652E-5\n10.36756\t1.0649E-5\n10.36944\t1.0647E-5\n10.37304\t1.0642E-5\n10.37496\t1.064E-5\n10.37684\t1.0637E-5\n10.37932\t1.0634E-5\n10.38236\t1.063E-5\n10.38432\t1.0627E-5\n10.38684\t1.0624E-5\n10.3894\t1.0621E-5\n10.39184\t1.0618E-5\n10.39504\t1.0613E-5\n10.39692\t1.0611E-5\n10.3994\t1.0608E-5\n10.40232\t1.0604E-5\n10.40481\t1.0601E-5\n10.40669\t1.0598E-5\n10.40929\t1.0595E-5\n10.41184\t1.0592E-5\n10.41464\t1.0588E-5\n10.41689\t1.0585E-5\n10.4194\t1.0582E-5\n10.42285\t1.0577E-5\n10.42489\t1.0574E-5\n10.42681\t1.0572E-5\n10.42917\t1.0569E-5\n10.43213\t1.0565E-5\n10.43521\t1.0561E-5\n10.43705\t1.0558E-5\n10.44005\t1.0555E-5\n10.44249\t1.0551E-5\n10.44441\t1.0549E-5\n10.44757\t1.0545E-5\n10.44949\t1.0542E-5\n10.45193\t1.0539E-5\n10.45453\t1.0536E-5\n10.45749\t1.0532E-5\n10.46033\t1.0528E-5\n10.46193\t1.0526E-5\n10.46385\t1.0523E-5\n10.46713\t1.0519E-5\n10.47029\t1.0515E-5\n10.47153\t1.0513E-5\n10.47429\t1.051E-5\n10.47781\t1.0505E-5\n10.47933\t1.0503E-5\n10.48225\t1.0499E-5\n10.48433\t1.0496E-5\n10.48689\t1.0493E-5\n10.48933\t1.049E-5\n10.49233\t1.0486E-5\n10.49425\t1.0483E-5\n10.49761\t1.0479E-5\n10.49965\t1.0476E-5\n10.50213\t1.0473E-5\n10.50497\t1.0469E-5\n10.50705\t1.0466E-5\n10.50949\t1.0463E-5\n10.51237\t1.0459E-5\n10.51497\t1.0456E-5\n10.51689\t1.0453E-5\n10.51977\t1.045E-5\n10.52245\t1.0446E-5\n10.52433\t1.0444E-5\n10.52781\t1.0439E-5\n10.52973\t1.0436E-5\n10.53173\t1.0434E-5\n10.53417\t1.0431E-5\n10.53673\t1.0427E-5\n10.53985\t1.0423E-5\n10.54177\t1.042E-5\n10.54477\t1.0417E-5\n10.54722\t1.0413E-5\n10.55013\t1.0409E-5\n10.55274\t1.0406E-5\n10.55461\t1.0403E-5\n10.55754\t1.04E-5\n10.56018\t1.0396E-5\n10.5621\t1.0394E-5\n10.56426\t1.0391E-5\n10.56818\t1.0385E-5\n10.57002\t1.0383E-5\n10.57202\t1.038E-5\n10.57506\t1.0376E-5\n10.57698\t1.0374E-5\n10.57942\t1.0371E-5\n10.5825\t1.0366E-5\n10.5849\t1.0363E-5\n10.5869\t1.0361E-5\n10.59002\t1.0356E-5\n10.59246\t1.0353E-5\n10.5943\t1.0351E-5\n10.59786\t1.0346E-5\n10.59934\t1.0344E-5\n10.6023\t1.034E-5\n10.60478\t1.0337E-5\n10.6067\t1.0334E-5\n10.61002\t1.033E-5\n10.61362\t1.0325E-5\n10.6145\t1.0324E-5\n10.61694\t1.0321E-5\n10.61998\t1.0316E-5\n10.62186\t1.0314E-5\n10.62418\t1.0311E-5\n10.6271\t1.0307E-5\n10.62954\t1.0304E-5\n10.63242\t1.03E-5\n10.63446\t1.0297E-5\n10.63694\t1.0294E-5\n10.63982\t1.029E-5\n10.64246\t1.0286E-5\n10.64438\t1.0284E-5\n10.64698\t1.028E-5\n10.64946\t1.0277E-5\n10.65194\t1.0274E-5\n10.65534\t1.0269E-5\n10.65698\t1.0267E-5\n10.65982\t1.0263E-5\n10.66186\t1.026E-5\n10.66498\t1.0256E-5\n10.66746\t1.0253E-5\n10.66938\t1.025E-5\n10.67194\t1.0247E-5\n10.67494\t1.0243E-5\n10.67726\t1.024E-5\n10.67891\t1.0238E-5\n10.68174\t1.0234E-5\n10.68459\t1.023E-5\n10.68711\t1.0227E-5\n10.69011\t1.0223E-5\n10.69171\t1.022E-5\n10.69527\t1.0216E-5\n10.69751\t1.0213E-5\n10.69991\t1.0209E-5\n10.70195\t1.0207E-5\n10.70487\t1.0203E-5\n10.70687\t1.02E-5\n10.70943\t1.0197E-5\n10.71155\t1.0194E-5\n10.71439\t1.019E-5\n10.71799\t1.0185E-5\n10.71947\t1.0183E-5\n10.72235\t1.0179E-5\n10.72583\t1.0174E-5\n10.72871\t1.0171E-5\n10.73211\t1.0166E-5\n10.73303\t1.0165E-5\n10.73611\t1.0161E-5\n10.73755\t1.0159E-5\n10.73951\t1.0156E-5\n10.74243\t1.0152E-5\n10.74491\t1.0149E-5\n10.74687\t1.0146E-5\n10.75039\t1.0141E-5\n10.75183\t1.0139E-5\n10.75443\t1.0136E-5\n10.75747\t1.0132E-5\n10.75939\t1.0129E-5\n10.76187\t1.0126E-5\n10.76487\t1.0122E-5\n10.76679\t1.0119E-5\n10.77107\t1.0113E-5\n10.77303\t1.0111E-5\n10.77495\t1.0108E-5\n10.77759\t1.0104E-5\n10.77947\t1.0102E-5\n10.78187\t1.0099E-5\n10.78495\t1.0094E-5\n10.78739\t1.0091E-5\n10.78927\t1.0089E-5\n10.79227\t1.0085E-5\n10.79467\t1.0081E-5\n10.79759\t1.0077E-5\n10.80031\t1.0074E-5\n10.80216\t1.0071E-5\n10.80503\t1.0067E-5\n10.80767\t1.0064E-5\n10.80955\t1.0061E-5\n10.813\t1.0056E-5\n10.81455\t1.0054E-5\n10.81752\t1.005E-5\n10.81992\t1.0047E-5\n10.82192\t1.0044E-5\n10.82492\t1.004E-5\n10.82684\t1.0038E-5\n10.82944\t1.0034E-5\n10.83192\t1.0031E-5\n10.83488\t1.0027E-5\n10.837\t1.0024E-5\n10.83956\t1.002E-5\n10.84304\t1.0015E-5\n10.84528\t1.0012E-5\n10.84712\t1.001E-5\n10.84948\t1.0007E-5\n10.85204\t1.0003E-5\n10.85568\t9.9982E-6\n10.85756\t9.9956E-6\n10.85956\t9.9929E-6\n10.86208\t9.9894E-6\n10.86512\t9.9853E-6\n10.8674\t9.9821E-6\n10.86988\t9.9788E-6\n10.87172\t9.9762E-6\n10.87528\t9.9714E-6\n10.8768\t9.9693E-6\n10.87968\t9.9653E-6\n10.88284\t9.961E-6\n10.88468\t9.9585E-6\n10.88772\t9.9543E-6\n10.88976\t9.9515E-6\n10.89168\t9.9489E-6\n10.89512\t9.9442E-6\n10.8972\t9.9413E-6\n10.8992\t9.9386E-6\n10.90164\t9.9353E-6\n10.9042\t9.9317E-6\n10.90684\t9.9281E-6\n10.90972\t9.9242E-6\n10.9134\t9.9191E-6\n10.91428\t9.9179E-6\n10.9168\t9.9144E-6\n10.91932\t9.911E-6\n10.92232\t9.9069E-6\n10.92428\t9.9042E-6\n10.92772\t9.8994E-6\n10.92952\t9.897E-6\n10.93248\t9.8929E-6\n10.93448\t9.8901E-6\n10.93797\t9.8853E-6\n10.93964\t9.883E-6\n10.94272\t9.8788E-6\n10.94513\t9.8755E-6\n10.94701\t9.8729E-6\n10.95025\t9.8684E-6\n10.95209\t9.8659E-6\n10.95481\t9.8621E-6\n10.95753\t9.8584E-6\n10.9594\t9.8558E-6\n10.96289\t9.851E-6\n10.96489\t9.8482E-6\n10.96681\t9.8456E-6\n10.96925\t9.8422E-6\n10.97217\t9.8382E-6\n10.97397\t9.8357E-6\n10.97597\t9.8329E-6\n10.97997\t9.8274E-6\n10.98085\t9.8262E-6\n10.98369\t9.8223E-6\n10.98569\t9.8195E-6\n10.98837\t9.8158E-6\n10.99077\t9.8125E-6\n10.99437\t9.8075E-6\n10.99653\t9.8045E-6\n10.99837\t9.8019E-6\n11.00233\t9.7965E-6\n11.00373\t9.7945E-6\n11.00565\t9.7919E-6\n11.00953\t9.7865E-6\n11.01101\t9.7844E-6\n11.01313\t9.7815E-6\n11.01761\t9.7753E-6\n11.01813\t9.7746E-6\n11.02101\t9.7706E-6\n11.02421\t9.7661E-6\n11.02613\t9.7635E-6\n11.02701\t9.7622E-6\n11.03041\t9.7575E-6\n11.03205\t9.7552E-6\n11.03497\t9.7512E-6\n11.03741\t9.7478E-6\n11.03937\t9.7451E-6\n11.04289\t9.7402E-6\n11.04437\t9.7381E-6\n11.04741\t9.7339E-6\n11.04989\t9.7304E-6\n11.05141\t9.7283E-6\n11.05493\t9.7234E-6\n11.05685\t9.7208E-6\n11.05929\t9.7174E-6\n11.06177\t9.7139E-6\n11.06481\t9.7097E-6\n11.06721\t9.7063E-6\n11.06925\t9.7035E-6\n11.07217\t9.6994E-6\n11.07457\t9.6961E-6\n11.07757\t9.6919E-6\n11.07997\t9.6885E-6\n11.08186\t9.6859E-6\n11.08501\t9.6815E-6\n11.08702\t9.6787E-6\n11.08989\t9.6747E-6\n11.0925\t9.671E-6\n11.09438\t9.6684E-6\n11.0973\t9.6643E-6\n11.09942\t9.6614E-6\n11.10194\t9.6579E-6\n11.10438\t9.6544E-6\n11.10706\t9.6507E-6\n11.11058\t9.6458E-6\n11.1125\t9.6431E-6\n11.11458\t9.6402E-6\n11.11702\t9.6368E-6\n11.1199\t9.6327E-6\n11.12194\t9.6299E-6\n11.12446\t9.6263E-6\n11.12694\t9.6229E-6\n11.12954\t9.6192E-6\n11.13242\t9.6152E-6\n11.13398\t9.613E-6\n11.1381\t9.6072E-6\n11.14066\t9.6036E-6\n11.14346\t9.5997E-6\n11.14598\t9.5962E-6\n11.14934\t9.5914E-6\n11.15222\t9.5874E-6\n11.15326\t9.5859E-6\n11.1555\t9.5828E-6\n11.15986\t9.5767E-6\n11.16046\t9.5758E-6\n11.16394\t9.5709E-6\n11.16626\t9.5677E-6\n11.16882\t9.5641E-6\n11.17098\t9.561E-6\n11.1725\t9.5589E-6\n11.17454\t9.556E-6\n11.17702\t9.5525E-6\n11.1799\t9.5485E-6\n11.18186\t9.5457E-6\n11.18438\t9.5422E-6\n11.1869\t9.5386E-6\n11.18942\t9.5351E-6\n11.19246\t9.5308E-6\n11.19434\t9.5281E-6\n11.1969\t9.5245E-6\n11.1999\t9.5203E-6\n11.2023\t9.5169E-6\n11.20434\t9.514E-6\n11.20734\t9.5098E-6\n11.20982\t9.5063E-6\n11.21179\t9.5035E-6\n11.2155\t9.4983E-6\n11.21739\t9.4956E-6\n11.21934\t9.4928E-6\n11.22187\t9.4893E-6\n11.22471\t9.4852E-6\n11.22831\t9.4801E-6\n11.23015\t9.4775E-6\n11.23203\t9.4749E-6\n11.23459\t9.4713E-6\n11.23751\t9.4671E-6\n11.23939\t9.4645E-6\n11.24151\t9.4615E-6\n11.24407\t9.4578E-6\n11.24663\t9.4542E-6\n11.24959\t9.45E-6\n11.25211\t9.4464E-6\n11.25503\t9.4423E-6\n11.25707\t9.4394E-6\n11.25951\t9.436E-6\n11.26247\t9.4318E-6\n11.26455\t9.4288E-6\n11.26799\t9.4239E-6\n11.26947\t9.4218E-6\n11.27203\t9.4182E-6\n11.27503\t9.4139E-6\n11.27743\t9.4105E-6\n11.27943\t9.4077E-6\n11.28239\t9.4035E-6\n11.28479\t9.4E-6\n11.28687\t9.3971E-6\n11.29035\t9.3921E-6\n11.29215\t9.3896E-6\n11.29527\t9.3851E-6\n11.29775\t9.3816E-6\n11.29967\t9.3789E-6\n11.30255\t9.3748E-6\n11.30443\t9.3721E-6\n11.30731\t9.368E-6\n11.30983\t9.3644E-6\n11.31183\t9.3616E-6\n11.31511\t9.3569E-6\n11.31779\t9.3531E-6\n11.31987\t9.3501E-6\n11.32131\t9.348E-6\n11.32363\t9.3447E-6\n11.32611\t9.3412E-6\n11.32867\t9.3375E-6\n11.32955\t9.3363E-6\n11.33263\t9.3319E-6\n11.33503\t9.3284E-6\n11.33695\t9.3257E-6\n11.34008\t9.3212E-6\n11.34248\t9.3178E-6\n11.34439\t9.3151E-6\n11.34799\t9.3099E-6\n11.34983\t9.3073E-6\n11.35176\t9.3045E-6\n11.35527\t9.2995E-6\n11.35712\t9.2969E-6\n11.36056\t9.2919E-6\n11.36303\t9.2884E-6\n11.36496\t9.2856E-6\n11.36692\t9.2828E-6\n11.37\t9.2784E-6\n11.37192\t9.2757E-6\n11.374\t9.2727E-6\n11.37656\t9.269E-6\n11.37996\t9.2641E-6\n11.3818\t9.2615E-6\n11.3854\t9.2563E-6\n11.38692\t9.2542E-6\n11.38984\t9.25E-6\n11.39244\t9.2462E-6\n11.39432\t9.2435E-6\n11.39772\t9.2386E-6\n11.39972\t9.2358E-6\n11.40172\t9.2329E-6\n11.40424\t9.2293E-6\n11.4072\t9.225E-6\n11.40992\t9.2211E-6\n11.4118\t9.2184E-6\n11.41488\t9.214E-6\n11.41688\t9.2111E-6\n11.41984\t9.2068E-6\n11.42244\t9.2031E-6\n11.42432\t9.2004E-6\n11.42724\t9.1962E-6\n11.4298\t9.1925E-6\n11.4318\t9.1896E-6\n11.43532\t9.1845E-6\n11.43732\t9.1817E-6\n11.43952\t9.1785E-6\n11.44192\t9.175E-6\n11.44444\t9.1714E-6\n11.44708\t9.1676E-6\n11.44992\t9.1635E-6\n11.45196\t9.1605E-6\n11.45508\t9.156E-6\n11.45696\t9.1533E-6\n11.45944\t9.1497E-6\n11.4618\t9.1463E-6\n11.46464\t9.1422E-6\n11.46732\t9.1383E-6\n11.46924\t9.1356E-6\n11.47264\t9.1306E-6\n11.47464\t9.1278E-6\n11.4776\t9.1235E-6\n11.4796\t9.1206E-6\n11.48272\t9.1161E-6\n11.48508\t9.1126E-6\n11.48665\t9.1104E-6\n11.48921\t9.1067E-6\n11.49265\t9.1017E-6\n11.49457\t9.0989E-6\n11.49709\t9.0952E-6\n11.50001\t9.091E-6\n11.50193\t9.0882E-6\n11.50445\t9.0846E-6\n11.50749\t9.0802E-6\n11.50997\t9.0766E-6\n11.51205\t9.0735E-6\n11.51501\t9.0692E-6\n11.51737\t9.0658E-6\n11.51945\t9.0628E-6\n11.52293\t9.0577E-6\n11.52489\t9.0549E-6\n11.52685\t9.052E-6\n11.52933\t9.0484E-6\n11.53217\t9.0443E-6\n11.53581\t9.039E-6\n11.53761\t9.0364E-6\n11.53953\t9.0336E-6\n11.54205\t9.0299E-6\n11.54473\t9.026E-6\n11.54813\t9.0211E-6\n11.55021\t9.0181E-6\n11.55265\t9.0145E-6\n11.55505\t9.011E-6\n11.55709\t9.008E-6\n11.56053\t9.003E-6\n11.56249\t9.0002E-6\n11.56453\t8.9972E-6\n11.56701\t8.9936E-6\n11.56993\t8.9893E-6\n11.57197\t8.9863E-6\n11.57441\t8.9828E-6\n11.57689\t8.9791E-6\n11.58109\t8.973E-6\n11.58313\t8.97E-6\n11.58501\t8.9673E-6\n11.58765\t8.9634E-6\n11.59017\t8.9597E-6\n11.59257\t8.9562E-6\n11.59457\t8.9533E-6\n11.59753\t8.949E-6\n11.59997\t8.9454E-6\n11.60201\t8.9424E-6\n11.60553\t8.9373E-6\n11.60698\t8.9352E-6\n11.61005\t8.9307E-6\n11.61245\t8.9271E-6\n11.61437\t8.9243E-6\n11.61793\t8.9191E-6\n11.61986\t8.9163E-6\n11.62177\t8.9135E-6\n11.62537\t8.9082E-6\n11.62682\t8.9061E-6\n11.6303\t8.901E-6\n11.63238\t8.8979E-6\n11.63434\t8.8951E-6\n11.63642\t8.892E-6\n11.63978\t8.8871E-6\n11.64318\t8.8821E-6\n11.6451\t8.8793E-6\n11.6471\t8.8763E-6\n11.64958\t8.8727E-6\n11.65254\t8.8683E-6\n11.6545\t8.8654E-6\n11.65698\t8.8618E-6\n11.65946\t8.8581E-6\n11.66198\t8.8544E-6\n11.6649\t8.8501E-6\n11.66682\t8.8473E-6\n11.67094\t8.8413E-6\n11.67342\t8.8376E-6\n11.67618\t8.8335E-6\n11.6783\t8.8304E-6\n11.6817\t8.8254E-6\n11.68366\t8.8225E-6\n11.68522\t8.8202E-6\n11.68762\t8.8167E-6\n11.68922\t8.8143E-6\n11.69214\t8.81E-6\n11.69458\t8.8064E-6\n11.69706\t8.8028E-6\n11.69958\t8.799E-6\n11.70246\t8.7948E-6\n11.7055\t8.7903E-6\n11.70766\t8.7871E-6\n11.70958\t8.7843E-6\n11.71198\t8.7807E-6\n11.71578\t8.7751E-6\n11.71922\t8.77E-6\n11.7221\t8.7658E-6\n11.72314\t8.7642E-6\n11.72506\t8.7614E-6\n11.72742\t8.7579E-6\n11.7301\t8.7539E-6\n11.73246\t8.7504E-6\n11.73438\t8.7476E-6\n11.73738\t8.7431E-6\n11.73986\t8.7395E-6\n11.74182\t8.7366E-6\n11.74542\t8.7312E-6\n11.74722\t8.7286E-6\n11.74971\t8.7249E-6\n11.75218\t8.7212E-6\n11.75475\t8.7174E-6\n11.75719\t8.7138E-6\n11.7603\t8.7092E-6\n11.76223\t8.7063E-6\n11.76443\t8.703E-6\n11.76699\t8.6992E-6\n11.76951\t8.6955E-6\n11.77243\t8.6912E-6\n11.77447\t8.6881E-6\n11.77695\t8.6844E-6\n11.77987\t8.6801E-6\n11.78247\t8.6762E-6\n11.78435\t8.6734E-6\n11.78683\t8.6698E-6\n11.78955\t8.6657E-6\n11.79175\t8.6624E-6\n11.79503\t8.6576E-6\n11.79715\t8.6544E-6\n11.79923\t8.6513E-6\n11.80215\t8.6469E-6\n11.80531\t8.6422E-6\n11.80675\t8.6401E-6\n11.80959\t8.6359E-6\n11.81335\t8.6303E-6\n11.81447\t8.6286E-6\n11.81739\t8.6242E-6\n11.81979\t8.6207E-6\n11.82183\t8.6176E-6\n11.82467\t8.6134E-6\n11.82679\t8.6102E-6\n11.82979\t8.6057E-6\n11.83227\t8.602E-6\n11.83523\t8.5976E-6\n11.83707\t8.5949E-6\n11.83943\t8.5913E-6\n11.84239\t8.5869E-6\n11.84511\t8.5828E-6\n11.84711\t8.5799E-6\n11.85067\t8.5745E-6\n11.85251\t8.5718E-6\n11.85443\t8.5689E-6\n11.85695\t8.5651E-6\n11.85995\t8.5606E-6\n11.86187\t8.5578E-6\n11.86435\t8.5541E-6\n11.86695\t8.5502E-6\n11.86951\t8.5463E-6\n11.87264\t8.5416E-6\n11.87507\t8.538E-6\n11.87695\t8.5352E-6\n11.87959\t8.5312E-6\n11.88207\t8.5275E-6\n11.88455\t8.5238E-6\n11.88708\t8.52E-6\n11.89004\t8.5155E-6\n11.89195\t8.5127E-6\n11.89615\t8.5064E-6\n11.89804\t8.5035E-6\n11.90248\t8.4969E-6\n11.90336\t8.4955E-6\n11.90628\t8.4911E-6\n11.90948\t8.4863E-6\n11.91148\t8.4833E-6\n11.91352\t8.4803E-6\n11.91656\t8.4757E-6\n11.91856\t8.4727E-6\n11.92004\t8.4705E-6\n11.92248\t8.4668E-6\n11.92448\t8.4638E-6\n11.92752\t8.4592E-6\n11.92944\t8.4563E-6\n11.93248\t8.4517E-6\n11.93492\t8.448E-6\n11.9368\t8.4452E-6\n11.94044\t8.4397E-6\n11.94192\t8.4375E-6\n11.94484\t8.4331E-6\n11.94736\t8.4293E-6\n11.94952\t8.426E-6\n11.95292\t8.4209E-6\n11.95504\t8.4177E-6\n11.95692\t8.4149E-6\n11.959\t8.4117E-6\n11.96192\t8.4073E-6\n11.96544\t8.402E-6\n11.96724\t8.3993E-6\n11.96936\t8.3961E-6\n11.97188\t8.3923E-6\n11.97432\t8.3886E-6\n11.97696\t8.3846E-6\n11.97908\t8.3814E-6\n11.98\t8.38E-6"
  in  "use independent curve":bool
  out "bkg and subtracted data":T1(graph)
  in  "remove bkg":bool=TRUE
  in  "Bbkg final":dbl=5.0 format="%.2f"
  in  "Bbkg initial":dbl=4.0 format="%.2f"
  in  "poly. order":i32=2
  in  "bkg removal method":T2(ring)
  in  "integration method":T3=1 items=["Trapezoidal Rule", "Simpson's Rule", "Simpson's 3/8 Rule", "Bode Rule"]
  in  "export":T4(ring)=enum."write to clipboard"
  out "raw data/bkg":T5(graph)
  in  "interpol. method":i32(ring)=2 items=["nearest", "linear", "spline", "cubic Hermite", "Lagrange"]
  in  "stop":bool
  in  "use variables":bool
  in  "Interpolation #":i32=5000
  in  "export data":bool
  in  "smoothing factor":i32=1
  in  "final":dbl=5.0 format="%.2f"
  in  "init":dbl format="%.2f"
  out "integrated":cluster{"xi used":dbl[], "Integral X":dbl[]}[](graph)
  in  "variable":string="4.2\n3.5\n3"
  # "(0) Data are clipped defined by the 'init' and 'final'.\n(1) Boxcar averaging (use 'smoothing factor' for adjustment)\n(3) Background removal if necessary. Background removal is done by polynomial (normal or Chebychev).\n            i) fitting is done for the range given by 'Bbkg init' and 'Bbkg final'.\n            ii) the background curve is extended to the whole data range."
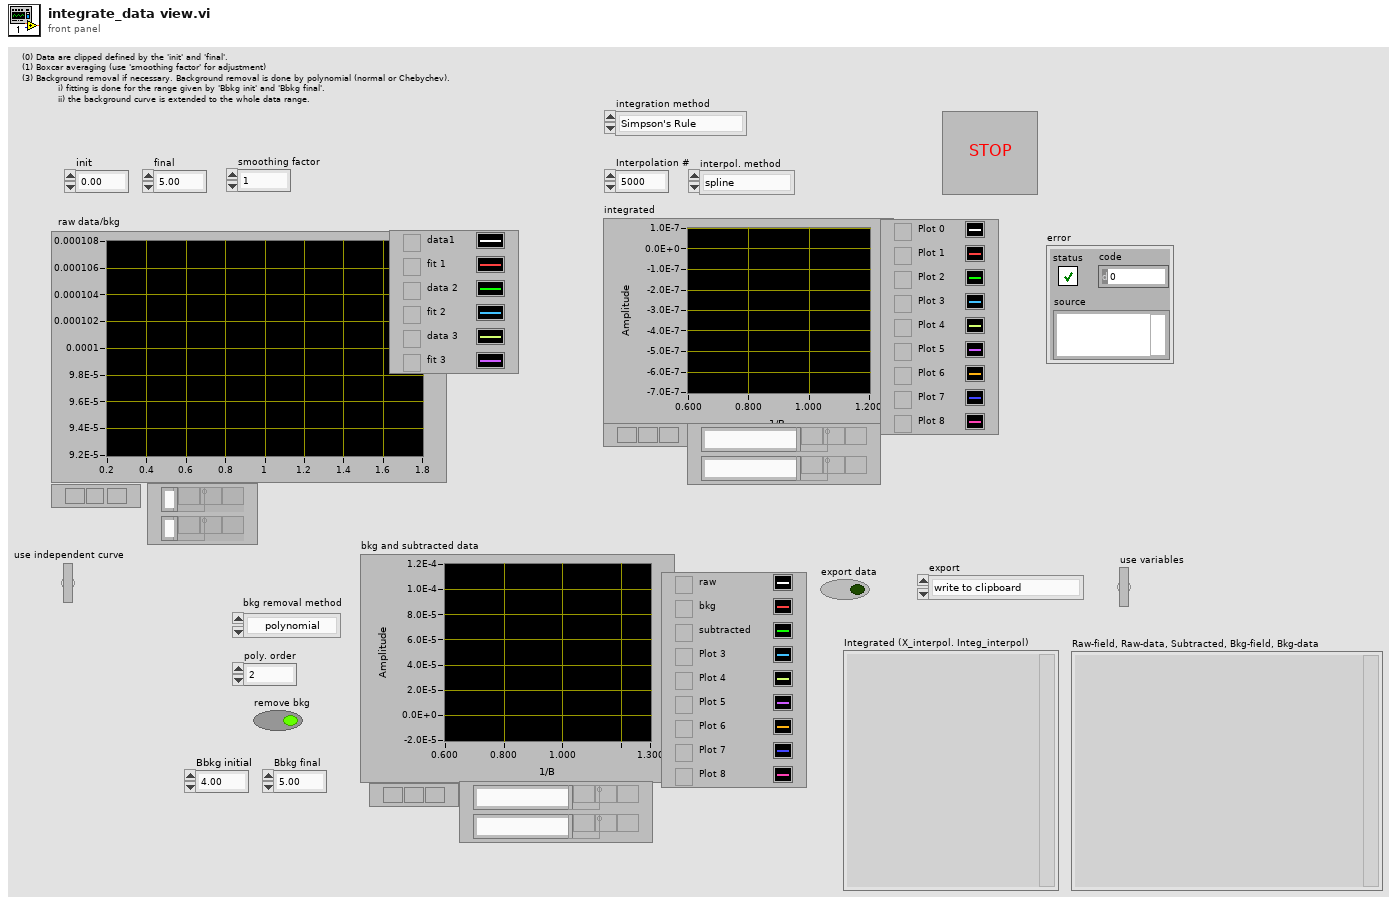
[diagram p1: front panel]
types:
  T1 = cluster{"all rows":dbl[], "extended data":dbl[]}[]
  T2 = enum16{"polynomial", "Cheby poly", "use indep curve "}
  T3 = typedef "NI_AALPro.lvlib/Integral Method.ctl" = i32
  T4 = enum16{"Save as Ascill file", "write to clipboard", "write to Igor ITX file"}
  T5 = cluster{"Ramp Pattern":dbl[], "Power Spectrum":dbl[]}[]
  T6 = enum16{"Save as Ascill file", "write to clipboard", "do not export"}
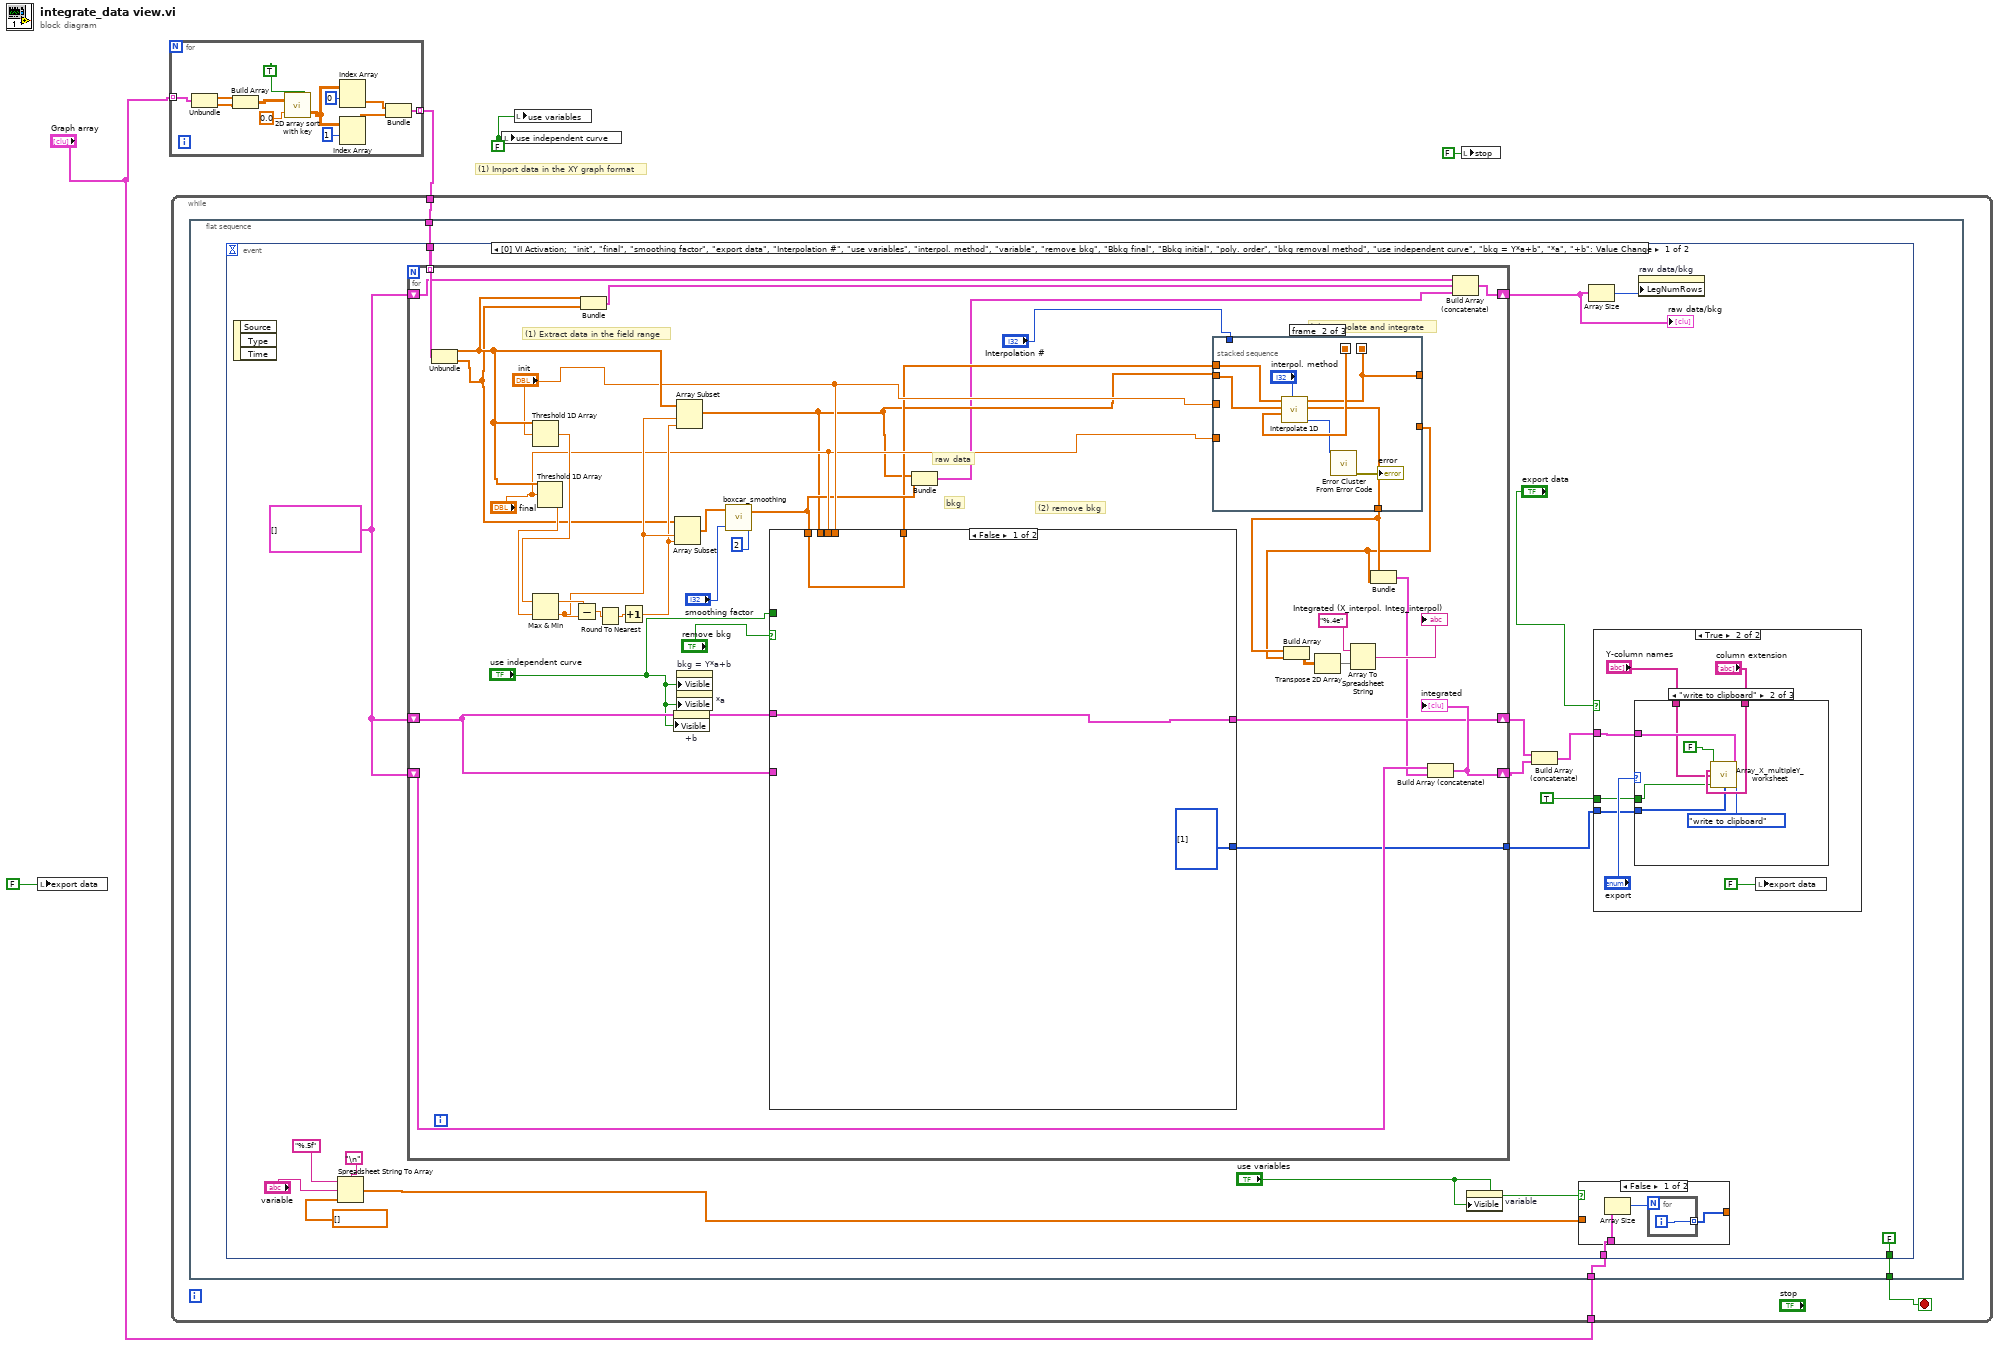
[diagram p0: block diagram]
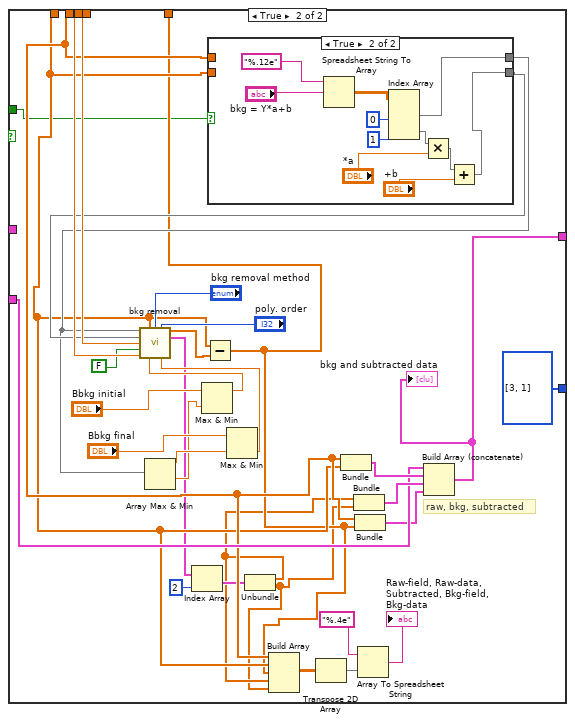
[diagram p3: hidden frame]
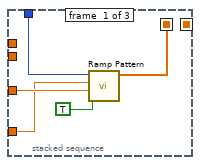
[diagram p5: hidden frame]
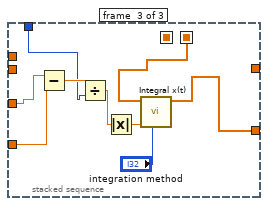
[diagram p6: hidden frame]
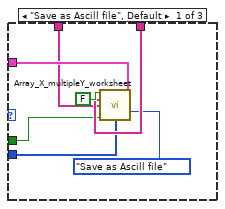
[diagram p8: hidden frame]
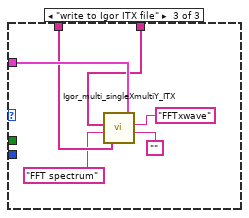
[diagram p9: hidden frame]
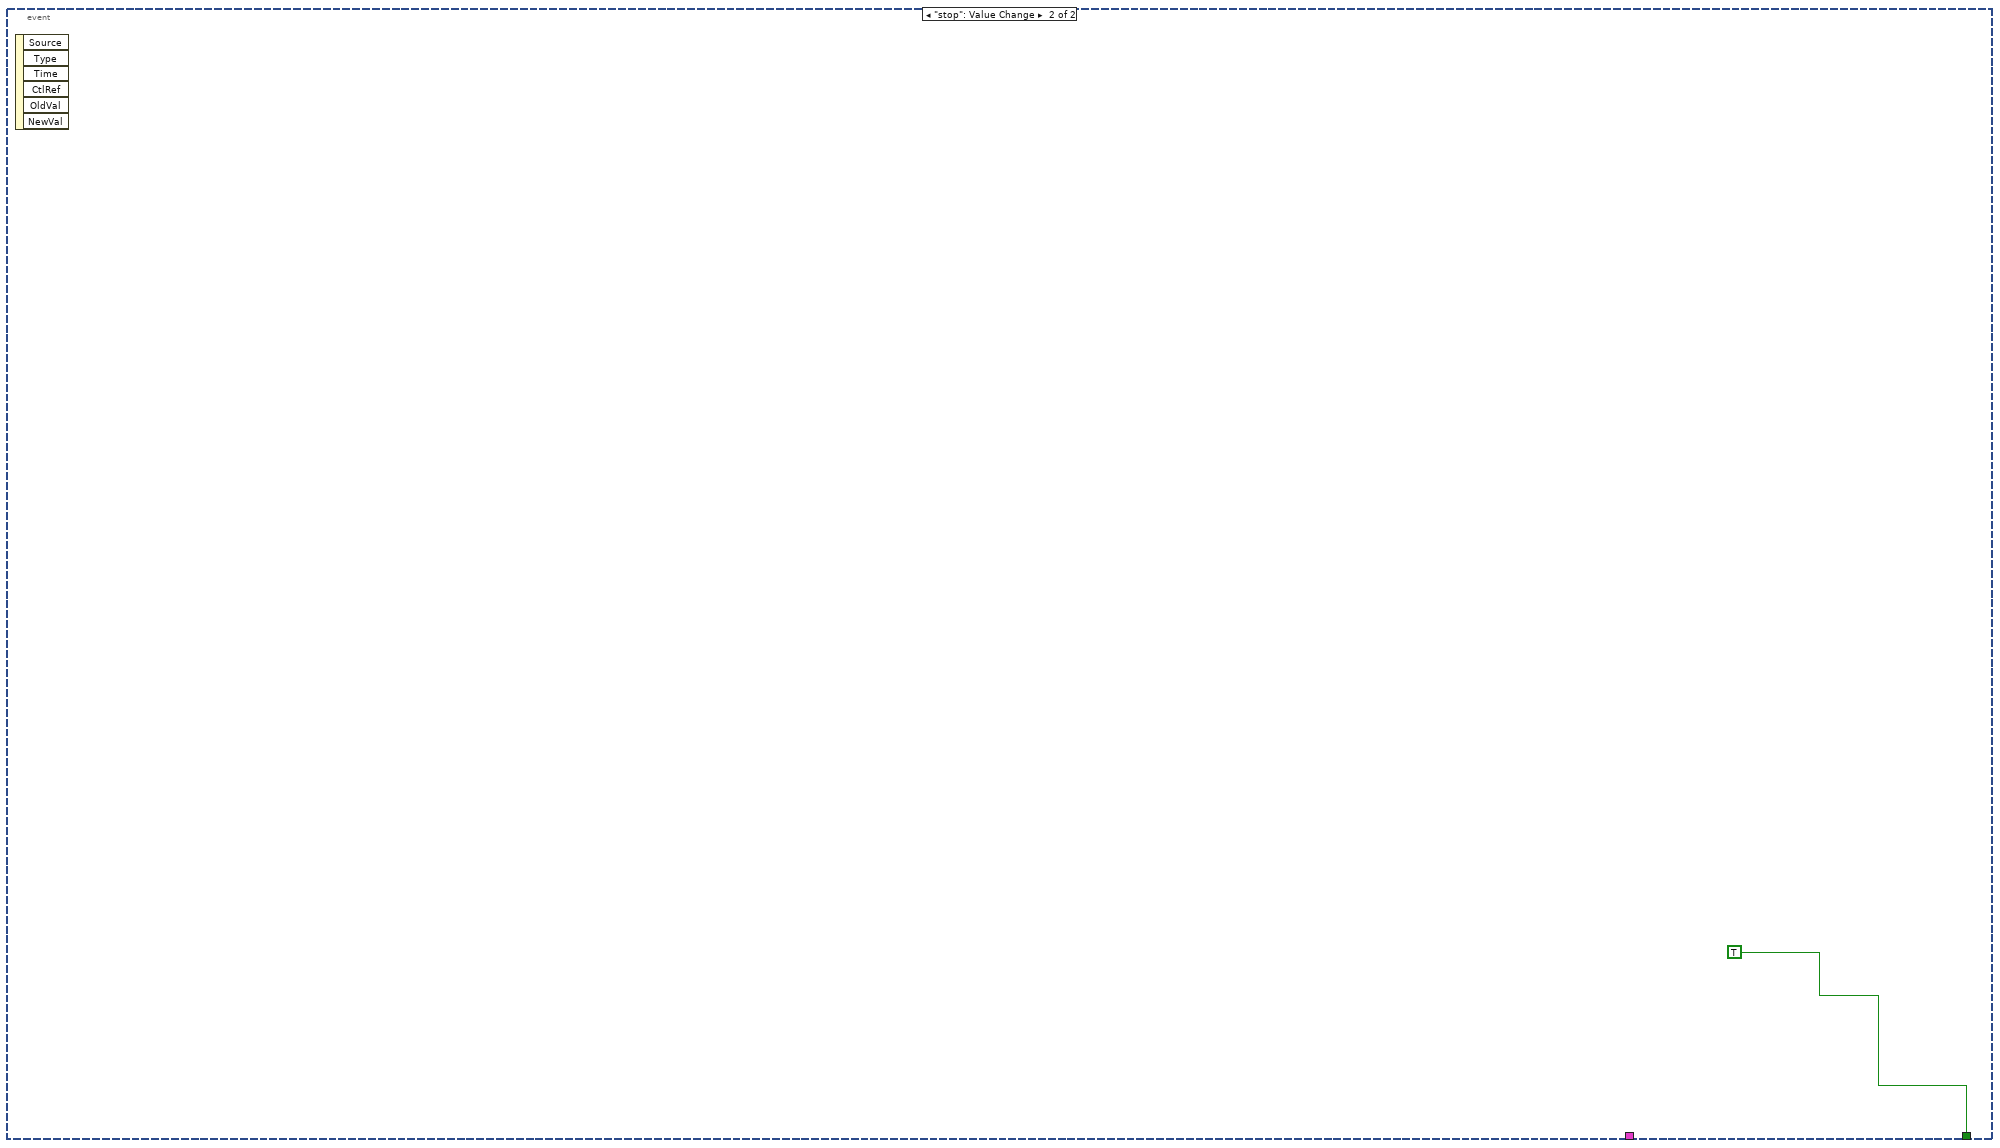
[diagram p10: hidden frame]
diagram:
  w1 = FALSE ("use independent curve")
  # "(1) Import data in the XY graph format"
  n1 = local write "export data"(FALSE ("export spectrum")) -> ()
  n2 = for {
    tunnel: "Graph array" -> [w17] mode=indexing
    tunnel: [w6] -> w4 mode=indexing
    n3 = Unbundle(w17) -> ("output"=w15:dbl[], "output"=w14:dbl[])
    n4 = Build Array(w15, w14) -> (w13:dbl[][])
    n5 = call "2D array sort with key.vi"("ascending"=TRUE, "key row"=0.0, "input"=w13) -> ("output"=w11:dbl[][])
    n6 = Index Array(array=w11, index (row)=0) -> (element=w8:dbl[])  [unwired: 1 in]
    n7 = Index Array(array=w11, index (row)=1) -> (element=w7:dbl[])  [unwired: 1 in]
    n8 = Bundle("output"=w8, "output"=w7) -> (w6:cluster{"output":dbl[], "output":dbl[]})  [unwired: 1 in]
  }
  n9 = while {
    tunnel: w4 -> [w20]
    tunnel: "Graph array" -> [w19]
    stop <- w18 stop-if-true
    n10 = flat-sequence {
      tunnel: w20 -> [w23]
      tunnel: w19 -> [w22]
      tunnel: [w21] -> w18
      frame #0 {
        n11 = event shown="[0] VI Activation;  \"init\", \"final\", \"smoothing factor\", \"export data\", \"Interpolation #\", \"use variables\", \"interpol. method\", \"variable\", \"remove bkg\", \"Bbkg final\", \"Bbkg initial\", \"poly. order\", \"bkg removal method\", \"use independent curve\", \"bkg = Y*a+b\", \"*a\", \"+b\": Value Change" {
          selector: _ -> [_ _]
          dyn-events: _ -> [_ _]
          timeout: _ -> [_ _]
          tunnel: w23 -> [w36 _]
          tunnel: w22 -> [w34 _]
          tunnel: [FALSE ("stop (press twice)") TRUE ("stop (press twice)")] -> w21
          event VI Activation; "init", "final", "smoothing factor", "export data", "Interpolation #", "use variables", "interpol. method", "variable", "remove bkg", "Bbkg final", "Bbkg initial", "poly. order", "bkg removal method", "use independent curve", "bkg = Y*a+b", "*a", "+b": Value Change {
            w26 = cluster{"all rows":sgl[], "all rows":sgl[]}[] []
            n12 = event-data() -> ()  [unwired: 1 in, 3 out]
            n13 = Spreadsheet String To Array(delimiter (Tab)="\n", format string="%.5f", spreadsheet string="variable", array type (2D Dbl)=dbl[] []) -> (array=w35:dbl[])
            n14 = for {
              shift-right: [w50] -> w29
              shift-left: w26 -> [w82]
              tunnel: w36 -> [w75] mode=indexing
              shift-right: [w73] -> w33
              shift-left: w26 -> [w72]
              shift-right: [w49] -> w28
              shift-left: w26 -> [w61]
              tunnel: [w47] -> w25
              # "(2) remove bkg"
              # "(3) interpolate and integrate"
              # "(1) Extract data in the field range"
              # "bkg"
              # "raw data"
              n15 = Unbundle(w75) -> ("output"=w71:dbl[], "output"=w69:dbl[])
              n16 = Threshold 1D Array(2:"init", 3:w71) -> (0:w81:dbl)  [unwired: 1 in]
              n17 = Threshold 1D Array(2:"final", 3:w71) -> (0:w80:dbl)  [unwired: 1 in]
              n18 = Max & Min(x=w81, y=w80) -> (max(x,y)=w79:dbl, min(x,y)=w77:dbl)
              n19 = Subtract(x=w79, y=w77) -> (x-y=w78:dbl)
              n20 = Bundle("output"=w71, "output"=w69) -> (w70:cluster{"output":dbl[], "output":dbl[]})  [unwired: 1 in]
              n21 = Round To Nearest(number=w78) -> (nearest integer value=w83:dbl)
              n22 = Increment(x=w83) -> (x+1=w76:dbl)
              n23 = property on="+b" class="DigNum (strict)"("Visible"="use independent curve") -> ()  [unwired: 2 in, 2 out]
              n24 = Array Subset(array=w69, index=w77, length=w76) -> (w68:dbl[])
              n25 = Array Subset(array=w71, index=w77, length=w76) -> (w59:dbl[])
              n26 = property on="bkg = Y*a+b" class="Str"("Visible"="use independent curve") -> ()  [unwired: 2 in, 2 out]
              n27 = property on="*a" class="DigNum (strict)"("Visible"="use independent curve") -> ()  [unwired: 2 in, 2 out]
              n28 = call "boxcar_smoothing.vi"("iteration Number"=2, "smooth factor"="smoothing factor", "raw data"=w68) -> ("smoothed"=w62:dbl[])  [unwired: 1 in]
              n29 = case shown="False" "remove bkg" {
                tunnel: w59 -> [_ w97]
                tunnel: w62 -> [w86 w96]
                tunnel: "init" -> [_ w119]
                tunnel: "final" -> [_ w118]
                tunnel: [w86 w91] -> w60
                tunnel: [w85 w105] -> w49
                tunnel: w61 -> [_ w106]
                tunnel: w61 -> [w85 _]
                tunnel: "use independent curve" -> [_ w88]
                tunnel: [u16[] [1] u16[] [3, 1]] -> w47
                frame False {
                }
                frame True {
                  # "raw, bkg, subtracted"
                  n30 = case shown="True" w88 {
                    tunnel: w97 -> [w121 _]
                    tunnel: [w121 w127] -> w102
                    tunnel: w96 -> [w120 _]
                    tunnel: [w120 w122] -> w103
                    frame False {
                    }
                    frame True {
                      n31 = Spreadsheet String To Array(format string="%.12e", spreadsheet string="bkg = Y*a+b") -> (array=w130:dbl[][])  [unwired: 2 in]
                      n32 = Index Array(array=w130, index (col) #1=0 ("disabled index (col)"), index (col) #2=1 ("index (col)")) -> (element #1=w127:dbl[], element #2=w126:dbl[])  [unwired: 2 in]
                      n33 = Multiply(x=w126, y="*a") -> (x*y=w125:dbl[])
                      n34 = Add(x=w125, y="+b") -> (x+y=w122:dbl[])
                    }
                  }
                  n35 = Array Max & Min(array=w102) -> (max value=w113:dbl, min value=w112:dbl)  [unwired: 2 out]
                  n36 = Max & Min(x="Bbkg initial", y=w112) -> (max(x,y)=w109:dbl)  [unwired: 1 out]
                  n37 = Max & Min(x="Bbkg final", y=w113) -> (min(x,y)=w110:dbl)  [unwired: 1 out]
                  n38 = call "bkg removal.vi"("Bfield"=w102, "array to be subtracted"=w96, "bkg removal method"="bkg removal method", "poly. order"="poly. order", "Data"=w103, "B initial"=w119, "inverse"=FALSE, "B final"=w118, "Bbkg initial"=w109, "Bbkg final"=w110) -> ("extended data"=w95:dbl[], "XY Graph"=w94:cluster{"Bfield":dbl[], "Data":dbl[]}[])  [unwired: 3 in, 1 out]
                  n39 = Index Array(array=w94, index=2) -> (element=w92:cluster{"Bfield":dbl[], "Data":dbl[]})
                  n40 = Subtract(x=w96, y=w95) -> (x-y=w91:dbl[])
                  n41 = Unbundle(w92) -> ("Bfield"=w90:dbl[], "Data"=w89:dbl[])
                  n42 = Build Array(w97, w96, w91, w90, w89) -> (w101:dbl[][])
                  n43 = Transpose 2D Array(2D array=w101) -> (transposed array=w99:dbl[][])
                  n44 = Bundle(w97, "smoothed"=w96) -> (w108:cluster{dbl[], "smoothed":dbl[]})  [unwired: 1 in]
                  n45 = Bundle("Bfield"=w90, "Data"=w89) -> (w107:cluster{"Bfield":dbl[], "Data":dbl[]})  [unwired: 1 in]
                  n46 = Bundle(w97, w91) -> (w104:cluster{dbl[], dbl[]})  [unwired: 1 in]
                  n47 = Array To Spreadsheet String(array=w99, 3:"%.4e" ("format string")) -> (spreadsheet string=→"Raw-field, Raw-data, Subtracted, Bkg-field, Bkg-data":string)  [unwired: 1 in]
                  n48 = Build Array (concatenate)(w106, w108, w107, w104) -> (w105:cluster{"Bfield":dbl[], "Data":dbl[]}[])
                  "bkg and subtracted data" <- w105
                }
              }
              n49 = Bundle(w59, "smoothed"=w62) -> (w58:cluster{dbl[], "smoothed":dbl[]})  [unwired: 1 in]
              n50 = stacked-sequence {
                seq-local: [w133 _ _] -> [_ w143 _]
                seq-local: [_ w140 _] -> [_ _ w149]
                tunnel: w60 -> [_ w145 _]
                tunnel: w59 -> [_ w142 _]
                tunnel: "Interpolation #" -> [w137 _ w150]
                tunnel: "init" -> [w136 _ w153]
                tunnel: "final" -> [w135 _ w152]
                tunnel: [_ _ w147] -> w56
                tunnel: [_ w141 _] -> w57
                tunnel: [_ w140 _] -> _
                frame #0 {
                  n51 = call-poly <vilib>:"Ramp Pattern.vi"("exclude end?"=TRUE, "start"=w136, "end"=w135, "samples"=w137) -> ("Ramp Pattern"=w133:dbl[])  [unwired: 6 in, 1 out]
                }
                frame #1 {
                  n52 = call <vilib>:"Interpolate 1D.vi"("method"="interpol. method", "xi"=w143, "X"=w142, "Y"=w145) -> ("error"=w138:i32, "xi used"=w141:dbl[], "yi"=w140:dbl[])  [unwired: 5 in]
                  n53 = call <vilib>:"Error Cluster From Error Code.vi"("error code (0)"=w138) -> ("error out"=→"error":errorcluster)  [unwired: 8 in]
                }
                frame #2 {
                  n54 = Subtract(x=w153, y=w152) -> (x-y=w151:dbl)
                  n55 = Divide(x=w151, y=w150) -> (x/y=w148:dbl)
                  n56 = Absolute Value(x=w148) -> (abs(x)=w146:dbl)
                  n57 = call <vilib>:"Integral x(t).vi"("integration method"="integration method", "dt"=w146, "X"=w149) -> ("Integral X"=w147:dbl[])  [unwired: 7 in, 1 out]
                }
              }
              n58 = Build Array(w57, w56) -> (w55:dbl[][])
              n59 = Transpose 2D Array(2D array=w55) -> (transposed array=w53:dbl[][])
              n60 = Array To Spreadsheet String(array=w53, 3:"%.4e" ("format string")) -> (spreadsheet string=→"Integrated (X_interpol. Integ_interpol)":string)  [unwired: 1 in]
              n61 = Bundle("xi used"=w57, "Integral X"=w56) -> (w48:cluster{"xi used":dbl[], "Integral X":dbl[]})  [unwired: 1 in]
              n62 = Build Array (concatenate)(w82, w48) -> (w50:cluster{"xi used":dbl[], "Integral X":dbl[]}[])
              "integrated" <- w50
              n63 = Build Array (concatenate)(w72, w70, w58) -> (w73:cluster{"output":dbl[], "smoothed":dbl[]}[])
            }
            "raw data/bkg" <- w33
            n64 = property on="variable" class="Str"("Visible"="use variables") -> ()  [unwired: 2 in, 2 out]
            n65 = Build Array (concatenate)(w28, w29) -> (w24:cluster{"xi used":dbl[], "Integral X":dbl[]}[])
            n66 = case shown="False" "use variables" {
              tunnel: w35 -> [_ w46]
              tunnel: [w43 w46] -> _
              tunnel: w34 -> [w42 _]
              frame False {
                n67 = Array Size(array=w42) -> (size(s)=w44:i32)
                n68 = for {
                  N: w44 -> [_]
                  tunnel: [w45] -> w43 mode=indexing
                  i -> [w45]
                }
              }
              frame True {
              }
            }
            n69 = Array Size(array=w33) -> (size(s)=w32:i32)
            n70 = case shown="True" "export data" {
              tunnel: w24 -> [_ w160]
              tunnel: TRUE ("appended graphs") -> [_ w156]
              tunnel: w25 -> [_ w155]
              frame False {
              }
              frame True {
                n71 = case shown="\"write to clipboard\"" "export" {
                  tunnel: w160 -> [w168 w175 w181]
                  tunnel: "column extension" -> [w166 w173 w180]
                  tunnel: "Y-column names" -> [w165 w172 w179]
                  tunnel: w156 -> [w163 w170 _]
                  tunnel: w155 -> [w162 w169 _]
                  frame "Save as Ascill file", Default {
                    n72 = call "Array_X_multipleY_worksheet.vi"("Sort?"=FALSE, "graph file"=w168, "column extension"=w166, "Y-column names"=w165, "export"=T6."Save as Ascill file", "appended graphs"=w163, "plot# per file"=w162) -> ()  [unwired: 7 in, 2 out]
                  }
                  frame "write to clipboard" {
                    n73 = call "Array_X_multipleY_worksheet.vi"("Sort?"=FALSE, "graph file"=w175, "column extension"=w173, "Y-column names"=w172, "export"=T6."write to clipboard", "appended graphs"=w170, "plot# per file"=w169) -> ()  [unwired: 7 in, 2 out]
                  }
                  frame "write to Igor ITX file" {
                    n74 = call "Igor_multi_singleXmultiY_ITX.vi"("message"="", "x-column name"="FFTxwave", "graph file"=w181, "Y-column names"=w179, "window name"="FFT spectrum", "column extension"=w180) -> ()  [unwired: 1 in, 1 out]
                  }
                }
                n75 = local write "export data"(FALSE ("export spectrum")) -> ()
              }
            }
            n76 = property on="raw data/bkg" class="XYGraph (strict)"("LegNumRows"=w32) -> ()  [unwired: 2 in, 2 out]
          }
          event "stop": Value Change {
            n77 = event-data() -> ()  [unwired: 1 in, 6 out]
          }
        }
      }
    }
  }
  n78 = local write "use independent curve"(w1) -> ()
  n79 = local write "use variables"(w1) -> ()
  n80 = local write "stop"(FALSE ("stop")) -> ()
